vi "参数生成器.vi"() -> ()   [LabVIEW 2013]
uses:
  <vilib>/Utility/config.llb/Write Key (String).vi
  <vilib>/Utility/config.llb/Read Key (String).vi
  <vilib>/Utility/file.llb/Read From Spreadsheet File (string).vi
  <vilib>/Utility/config.llb/Write Key (Path).vi
  <vilib>/Utility/config.llb/NI_LVConfig.lvlib
panel:
  in  "均衡参数设置":bool
  in  "error in":errorcluster caption="错误输入"
  out "临时从板数据":string[](array[string])
  in  "自动记录":bool
  in  "通道电压清零":bool
  in  "自动计算通道电压":bool
  out "均衡参数":T1={"充电结束电压(90%)"=3.0, "充电结束电压(91%)"=3.0, "充电结束电压(92%)"=3.0, "充电结束电压(93%)"=3.0, "充电结束电压(94%)"=3.0, "均衡计算-电压高阀值1级"=3.0, "均衡计算-电压高阀值2级"=3.0, "均衡计算-电压低阀值1级"=3.0, "均衡计算-电压低阀值2级"=3.0, "均衡计算-最低电压阀值"=3.0, "均衡停止-最低电压阀值"=3.0, "均衡计算-电压极差阀值"=3.0, "充电结束电压(95%)"=3.0, "充电结束电压(96%)"=3.0, "充电结束电压(97%)"=3.0, "充电结束电压(98%)"=3.0, "充电结束电压(99%)"=3.0, "充电结束电压(100%)"=3.0} {"充电结束电压(100%)" min=0 max=5 format="%#.4f"; "充电结束电压(99%)" min=0 max=5 format="%#.4f"; "充电结束电压(98%)" min=0 max=5 format="%#.4f"; "充电结束电压(97%)" min=0 max=5 format="%#.4f"; "充电结束电压(96%)" min=0 max=5 format="%#.4f"; "充电结束电压(95%)" min=0 max=5 format="%#.4f"; "均衡计算-电压极差阀值" min=0 max=5 format="%#.4f"; "均衡停止-最低电压阀值" min=0 max=5 format="%#.4f"; "均衡计算-最低电压阀值" min=0 max=5 format="%#.4f"; "均衡计算-电压低阀值2级" min=0 max=5 format="%#.4f"; "充电结束电压(94%)" min=0 max=5 format="%#.4f"; "充电结束电压(93%)" min=0 max=5 format="%#.4f"; "均衡计算-电压低阀值1级" min=0 max=5 format="%#.4f"; "均衡计算-电压高阀值1级" min=0 max=5 format="%#.4f"; "均衡计算-电压高阀值2级" min=0 max=5 format="%#.4f"; "充电结束电压(92%)" min=0 max=5 format="%#.4f"; "充电结束电压(91%)" min=0 max=5 format="%#.4f"; "充电结束电压(90%)" min=0 max=5 format="%#.4f"}
  in  "布尔":bool
  in  "全部记录":bool
  in  "查看":bool
  in  "读从板信息":bool
  in  "字符串":string
  out "MD5 message-digest":string="c47cafb9475eca419ba2638971991389" caption="MD5信息摘要"
  out "从板表头":string[](array[string])=["从板板号", "电压个数", "电压起始值", "温度个数", "温度起始值", "第一个保险通道", "第一个保险位置", "第二个保险通道", "第二个保险位置", "第三个保险通道", "第三个保险位置", "第四个保险通道", "第四个保险位置", "第五个保险通道", "第五个保险位置", "第六个保险通道", "第六个保险位置", "第七个保险通道", "第七个保险位置", "第八个保险通道", "第八个保险位置", "第九个保险通道", "第九个保险位置", "第十个保险通道", "第十个保险位置", "第1通道电压个数", "第2通道电压个数", "第3通道电压个数", "第4通道电压个数", "第5通道电压个数", "第6通道电压个数", "第7通道电压个数", "第8通道电压个数", "第9通道电压个数", "第10通道电压个数", "第11通道电压个数", "第12通道电压个数", "第13通道电压个数", "第14通道电压个数", "第15通道电压个数", "第16通道电压个数", "第17通道电压个数", "第18通道电压个数", "第19通道电压个数", "第20通道电压个数", "风机开启温度", "风机关闭温度", "加热开启温度", "加热关闭温度", "风机开启温差", "风机关闭温差", "加热关闭温差", "电压过高一级", "电压过低一级", "温度过高一级", "温度过低一级", "电压不均衡一级", "温度不均衡一级", "SOC过低一级", "电压过高二级", "电压过低二级", "温度过高二级", "温度过低二级", "电压不均衡二级", "温度不均衡二级", "SOC过低二级", "电压过高三级", "电压过低三级", "温度过高三级", "温度过低三级", "电压不均衡三级", "温度不均衡三级", "SOC过低三级", "均衡计算-电压高阀值1级", "均衡计算-电压高阀值2级", "均衡计算-电压低阀值1级", "均衡计算-电压低阀值2级", "均衡计算-最低电压阀值", "均衡停止-最低电压阀值", "均衡计算-电压极差阀值", "充电结束电压(90%)", "充电结束电压(91%)", "充电结束电压(92%)", "充电结束电压(93%)", "充电结束电压(94%)", "充电结束电压(95%)", "充电结束电压(96%)", "充电结束电压(97%)", "充电结束电压(98%)", "充电结束电压(99%)", "充电结束电压(100%)"]
  out "输出数组":string[][](array[string])=[["1", "2", "3", " ", " ", " ", " ", " ", " ", " ", " ", " ", " ", " ", " ", " ", " ", " ", " ", " ", " ", " ", " ", " ", " ", " ", " ", " ", " ", " "], ["10", "10", "10", " ", " ", " ", " ", " ", " ", " ", " ", " ", " ", " ", " ", " ", " ", " ", " ", " ", " ", " ", " ", " ", " ", " ", " ", " ", " ", " "], ["", "0", "0", " ", " ", " ", " ", " ", " ", " ", " ", " ", " ", " ", " ", " ", " ", " ", " ", " ", " ", " ", " ", " ", " ", " ", " ", " ", " ", " "], ["2", "2", "2", " ", " ", " ", " ", " ", " ", " ", " ", " ", " ", " ", " ", " ", " ", " ", " ", " ", " ", " ", " ", " ", " ", " ", " ", " ", " ", " "], ["", "0", "0", " ", " ", " ", " ", " ", " ", " ", " ", " ", " ", " ", " ", " ", " ", " ", " ", " ", " ", " ", " ", " ", " ", " ", " ", " ", " ", " "], [" ", " ", " ", " ", " ", " ", " ", " ", " ", " ", " ", " ", " ", " ", " ", " ", " ", " ", " ", " ", " ", " ", " ", " ", " ", " ", " ", " ", " ", " "], [" ", " ", " ", " ", " ", " ", " ", " ", " ", " ", " ", " ", " ", " ", " ", " ", " ", " ", " ", " ", " ", " ", " ", " ", " ", " ", " ", " ", " ", " "], [" ", " ", " ", " ", " ", " ", " ", " ", " ", " ", " ", " ", " ", " ", " ", " ", " ", " ", " ", " ", " ", " ", " ", " ", " ", " ", " ", " ", " ", " "], [" ", " ", " ", " ", " ", " ", " ", " ", " ", " ", " ", " ", " ", " ", " ", " ", " ", " ", " ", " ", " ", " ", " ", " ", " ", " ", " ", " ", " ", " "], [" ", " ", " ", " ", " ", " ", " ", " ", " ", " ", " ", " ", " ", " ", " ", " ", " ", " ", " ", " ", " ", " ", " ", " ", " ", " ", " ", " ", " ", " "], [" ", " ", " ", " ", " ", " ", " ", " ", " ", " ", " ", " ", " ", " ", " ", " ", " ", " ", " ", " ", " ", " ", " ", " ", " ", " ", " ", " ", " ", " "], [" ", " ", " ", " ", " ", " ", " ", " ", " ", " ", " ", " ", " ", " ", " ", " ", " ", " ", " ", " ", " ", " ", " ", " ", " ", " ", " ", " ", " ", " "], [" ", " ", " ", " ", " ", " ", " ", " ", " ", " ", " ", " ", " ", " ", " ", " ", " ", " ", " ", " ", " ", " ", " ", " ", " ", " ", " ", " ", " ", " "], [" ", " ", " ", " ", " ", " ", " ", " ", " ", " ", " ", " ", " ", " ", " ", " ", " ", " ", " ", " ", " ", " ", " ", " ", " ", " ", " ", " ", " ", " "], [" ", " ", " ", " ", " ", " ", " ", " ", " ", " ", " ", " ", " ", " ", " ", " ", " ", " ", " ", " ", " ", " ", " ", " ", " ", " ", " ", " ", " ", " "], [" ", " ", " ", " ", " ", " ", " ", " ", " ", " ", " ", " ", " ", " ", " ", " ", " ", " ", " ", " ", " ", " ", " ", " ", " ", " ", " ", " ", " ", " "], [" ", " ", " ", " ", " ", " ", " ", " ", " ", " ", " ", " ", " ", " ", " ", " ", " ", " ", " ", " ", " ", " ", " ", " ", " ", " ", " ", " ", " ", " "], [" ", " ", " ", " ", " ", " ", " ", " ", " ", " ", " ", " ", " ", " ", " ", " ", " ", " ", " ", " ", " ", " ", " ", " ", " ", " ", " ", " ", " ", " "], [" ", " ", " ", " ", " ", " ", " ", " ", " ", " ", " ", " ", " ", " ", " ", " ", " ", " ", " ", " ", " ", " ", " ", " ", " ", " ", " ", " ", " ", " "], [" ", " ", " ", " ", " ", " ", " ", " ", " ", " ", " ", " ", " ", " ", " ", " ", " ", " ", " ", " ", " ", " ", " ", " ", " ", " ", " ", " ", " ", " "], [" ", " ", " ", " ", " ", " ", " ", " ", " ", " ", " ", " ", " ", " ", " ", " ", " ", " ", " ", " ", " ", " ", " ", " ", " ", " ", " ", " ", " ", " "], [" ", " ", " ", " ", " ", " ", " ", " ", " ", " ", " ", " ", " ", " ", " ", " ", " ", " ", " ", " ", " ", " ", " ", " ", " ", " ", " ", " ", " ", " "], [" ", " ", " ", " ", " ", " ", " ", " ", " ", " ", " ", " ", " ", " ", " ", " ", " ", " ", " ", " ", " ", " ", " ", " ", " ", " ", " ", " ", " ", " "], [" ", " ", " ", " ", " ", " ", " ", " ", " ", " ", " ", " ", " ", " ", " ", " ", " ", " ", " ", " ", " ", " ", " ", " ", " ", " ", " ", " ", " ", " "], [" ", " ", " ", " ", " ", " ", " ", " ", " ", " ", " ", " ", " ", " ", " ", " ", " ", " ", " ", " ", " ", " ", " ", " ", " ", " ", " ", " ", " ", " "], [" ", " ", " ", " ", " ", " ", " ", " ", " ", " ", " ", " ", " ", " ", " ", " ", " ", " ", " ", " ", " ", " ", " ", " ", " ", " ", " ", " ", " ", " "], [" ", " ", " ", " ", " ", " ", " ", " ", " ", " ", " ", " ", " ", " ", " ", " ", " ", " ", " ", " ", " ", " ", " ", " ", " ", " ", " ", " ", " ", " "], [" ", " ", " ", " ", " ", " ", " ", " ", " ", " ", " ", " ", " ", " ", " ", " ", " ", " ", " ", " ", " ", " ", " ", " ", " ", " ", " ", " ", " ", " "], [" ", " ", " ", " ", " ", " ", " ", " ", " ", " ", " ", " ", " ", " ", " ", " ", " ", " ", " ", " ", " ", " ", " ", " ", " ", " ", " ", " ", " ", " "], [" ", " ", " ", " ", " ", " ", " ", " ", " ", " ", " ", " ", " ", " ", " ", " ", " ", " ", " ", " ", " ", " ", " ", " ", " ", " ", " ", " ", " ", " "], [" ", " ", " ", " ", " ", " ", " ", " ", " ", " ", " ", " ", " ", " ", " ", " ", " ", " ", " ", " ", " ", " ", " ", " ", " ", " ", " ", " ", " ", " "], [" ", " ", " ", " ", " ", " ", " ", " ", " ", " ", " ", " ", " ", " ", " ", " ", " ", " ", " ", " ", " ", " ", " ", " ", " ", " ", " ", " ", " ", " "], [" ", " ", " ", " ", " ", " ", " ", " ", " ", " ", " ", " ", " ", " ", " ", " ", " ", " ", " ", " ", " ", " ", " ", " ", " ", " ", " ", " ", " ", " "], [" ", " ", " ", " ", " ", " ", " ", " ", " ", " ", " ", " ", " ", " ", " ", " ", " ", " ", " ", " ", " ", " ", " ", " ", " ", " ", " ", " ", " ", " "], [" ", " ", " ", " ", " ", " ", " ", " ", " ", " ", " ", " ", " ", " ", " ", " ", " ", " ", " ", " ", " ", " ", " ", " ", " ", " ", " ", " ", " ", " "], [" ", " ", " ", " ", " ", " ", " ", " ", " ", " ", " ", " ", " ", " ", " ", " ", " ", " ", " ", " ", " ", " ", " ", " ", " ", " ", " ", " ", " ", " "], [" ", " ", " ", " ", " ", " ", " ", " ", " ", " ", " ", " ", " ", " ", " ", " ", " ", " ", " ", " ", " ", " ", " ", " ", " ", " ", " ", " ", " ", " "], [" ", " ", " ", " ", " ", " ", " ", " ", " ", " ", " ", " ", " ", " ", " ", " ", " ", " ", " ", " ", " ", " ", " ", " ", " ", " ", " ", " ", " ", " "], [" ", " ", " ", " ", " ", " ", " ", " ", " ", " ", " ", " ", " ", " ", " ", " ", " ", " ", " ", " ", " ", " ", " ", " ", " ", " ", " ", " ", " ", " "], [" ", " ", " ", " ", " ", " ", " ", " ", " ", " ", " ", " ", " ", " ", " ", " ", " ", " ", " ", " ", " ", " ", " ", " ", " ", " ", " ", " ", " ", " "], [" ", " ", " ", " ", " ", " ", " ", " ", " ", " ", " ", " ", " ", " ", " ", " ", " ", " ", " ", " ", " ", " ", " ", " ", " ", " ", " ", " ", " ", " "], [" ", " ", " ", " ", " ", " ", " ", " ", " ", " ", " ", " ", " ", " ", " ", " ", " ", " ", " ", " ", " ", " ", " ", " ", " ", " ", " ", " ", " ", " "], [" ", " ", " ", " ", " ", " ", " ", " ", " ", " ", " ", " ", " ", " ", " ", " ", " ", " ", " ", " ", " ", " ", " ", " ", " ", " ", " ", " ", " ", " "], [" ", " ", " ", " ", " ", " ", " ", " ", " ", " ", " ", " ", " ", " ", " ", " ", " ", " ", " ", " ", " ", " ", " ", " ", " ", " ", " ", " ", " ", " "], [" ", " ", " ", " ", " ", " ", " ", " ", " ", " ", " ", " ", " ", " ", " ", " ", " ", " ", " ", " ", " ", " ", " ", " ", " ", " ", " ", " ", " ", " "], ["35", "35", "35", " ", " ", " ", " ", " ", " ", " ", " ", " ", " ", " ", " ", " ", " ", " ", " ", " ", " ", " ", " ", " ", " ", " ", " ", " ", " ", " "], ["30", "30", "30", " ", " ", " ", " ", " ", " ", " ", " ", " ", " ", " ", " ", " ", " ", " ", " ", " ", " ", " ", " ", " ", " ", " ", " ", " ", " ", " "], ["0", "0", "0", " ", " ", " ", " ", " ", " ", " ", " ", " ", " ", " ", " ", " ", " ", " ", " ", " ", " ", " ", " ", " ", " ", " ", " ", " ", " ", " "], ["5", "5", "5", " ", " ", " ", " ", " ", " ", " ", " ", " ", " ", " ", " ", " ", " ", " ", " ", " ", " ", " ", " ", " ", " ", " ", " ", " ", " ", " "], ["5", "5", "5", " ", " ", " ", " ", " ", " ", " ", " ", " ", " ", " ", " ", " ", " ", " ", " ", " ", " ", " ", " ", " ", " ", " ", " ", " ", " ", " "], ["3", "3", "3", " ", " ", " ", " ", " ", " ", " ", " ", " ", " ", " ", " ", " ", " ", " ", " ", " ", " ", " ", " ", " ", " ", " ", " ", " ", " ", " "], ["10", "10", "10", " ", " ", " ", " ", " ", " ", " ", " ", " ", " ", " ", " ", " ", " ", " ", " ", " ", " ", " ", " ", " ", " ", " ", " ", " ", " ", " "], ["4.23", "4.23", "4.23", " ", " ", " ", " ", " ", " ", " ", " ", " ", " ", " ", " ", " ", " ", " ", " ", " ", " ", " ", " ", " ", " ", " ", " ", " ", " ", " "], ["3", "3", "3", " ", " ", " ", " ", " ", " ", " ", " ", " ", " ", " ", " ", " ", " ", " ", " ", " ", " ", " ", " ", " ", " ", " ", " ", " ", " ", " "], ["50", "50", "50", " ", " ", " ", " ", " ", " ", " ", " ", " ", " ", " ", " ", " ", " ", " ", " ", " ", " ", " ", " ", " ", " ", " ", " ", " ", " ", " "], ["-20", "-20", "-20", " ", " ", " ", " ", " ", " ", " ", " ", " ", " ", " ", " ", " ", " ", " ", " ", " ", " ", " ", " ", " ", " ", " ", " ", " ", " ", " "], ["0.5", "0.5", "0.5", " ", " ", " ", " ", " ", " ", " ", " ", " ", " ", " ", " ", " ", " ", " ", " ", " ", " ", " ", " ", " ", " ", " ", " ", " ", " ", " "], ["25", "25", "25", " ", " ", " ", " ", " ", " ", " ", " ", " ", " ", " ", " ", " ", " ", " ", " ", " ", " ", " ", " ", " ", " ", " ", " ", " ", " ", " "], ["30", "30", "30", " ", " ", " ", " ", " ", " ", " ", " ", " ", " ", " ", " ", " ", " ", " ", " ", " ", " ", " ", " ", " ", " ", " ", " ", " ", " ", " "], ["4.25", "4.25", "4.25", " ", " ", " ", " ", " ", " ", " ", " ", " ", " ", " ", " ", " ", " ", " ", " ", " ", " ", " ", " ", " ", " ", " ", " ", " ", " ", " "], ["2.75", "2.75", "2.75", " ", " ", " ", " ", " ", " ", " ", " ", " ", " ", " ", " ", " ", " ", " ", " ", " ", " ", " ", " ", " ", " ", " ", " ", " ", " ", " "], ["55", "55", "55", " ", " ", " ", " ", " ", " ", " ", " ", " ", " ", " ", " ", " ", " ", " ", " ", " ", " ", " ", " ", " ", " ", " ", " ", " ", " ", " "], ["-30", "-30", "-30", " ", " ", " ", " ", " ", " ", " ", " ", " ", " ", " ", " ", " ", " ", " ", " ", " ", " ", " ", " ", " ", " ", " ", " ", " ", " ", " "], ["1", "1", "1", " ", " ", " ", " ", " ", " ", " ", " ", " ", " ", " ", " ", " ", " ", " ", " ", " ", " ", " ", " ", " ", " ", " ", " ", " ", " ", " "], ["30", "30", "30", " ", " ", " ", " ", " ", " ", " ", " ", " ", " ", " ", " ", " ", " ", " ", " ", " ", " ", " ", " ", " ", " ", " ", " ", " ", " ", " "], ["20", "20", "20", " ", " ", " ", " ", " ", " ", " ", " ", " ", " ", " ", " ", " ", " ", " ", " ", " ", " ", " ", " ", " ", " ", " ", " ", " ", " ", " "], ["4.3", "4.3", "4.3", " ", " ", " ", " ", " ", " ", " ", " ", " ", " ", " ", " ", " ", " ", " ", " ", " ", " ", " ", " ", " ", " ", " ", " ", " ", " ", " "], ["2.5", "2.5", "2.5", " ", " ", " ", " ", " ", " ", " ", " ", " ", " ", " ", " ", " ", " ", " ", " ", " ", " ", " ", " ", " ", " ", " ", " ", " ", " ", " "], ["60", "60", "60", " ", " ", " ", " ", " ", " ", " ", " ", " ", " ", " ", " ", " ", " ", " ", " ", " ", " ", " ", " ", " ", " ", " ", " ", " ", " ", " "], ["-40", "-40", "-40", " ", " ", " ", " ", " ", " ", " ", " ", " ", " ", " ", " ", " ", " ", " ", " ", " ", " ", " ", " ", " ", " ", " ", " ", " ", " ", " "], ["1.5", "1.5", "1.5", " ", " ", " ", " ", " ", " ", " ", " ", " ", " ", " ", " ", " ", " ", " ", " ", " ", " ", " ", " ", " ", " ", " ", " ", " ", " ", " "], ["35", "35", "35", " ", " ", " ", " ", " ", " ", " ", " ", " ", " ", " ", " ", " ", " ", " ", " ", " ", " ", " ", " ", " ", " ", " ", " ", " ", " ", " "], ["10", "10", "10", " ", " ", " ", " ", " ", " ", " ", " ", " ", " ", " ", " ", " ", " ", " ", " ", " ", " ", " ", " ", " ", " ", " ", " ", " ", " ", " "], ["3", "4.23", "4.23", " ", " ", " ", " ", " ", " ", " ", " ", " ", " ", " ", " ", " ", " ", " ", " ", " ", " ", " ", " ", " ", " ", " ", " ", " ", " ", " "], ["3", "3", "3", " ", " ", " ", " ", " ", " ", " ", " ", " ", " ", " ", " ", " ", " ", " ", " ", " ", " ", " ", " ", " ", " ", " ", " ", " ", " ", " "], ["3", "50", "50", " ", " ", " ", " ", " ", " ", " ", " ", " ", " ", " ", " ", " ", " ", " ", " ", " ", " ", " ", " ", " ", " ", " ", " ", " ", " ", " "], ["3", "-20", "-20", " ", " ", " ", " ", " ", " ", " ", " ", " ", " ", " ", " ", " ", " ", " ", " ", " ", " ", " ", " ", " ", " ", " ", " ", " ", " ", " "], ["3", "0.5", "0.5", " ", " ", " ", " ", " ", " ", " ", " ", " ", " ", " ", " ", " ", " ", " ", " ", " ", " ", " ", " ", " ", " ", " ", " ", " ", " ", " "], ["3", "25", "25", " ", " ", " ", " ", " ", " ", " ", " ", " ", " ", " ", " ", " ", " ", " ", " ", " ", " ", " ", " ", " ", " ", " ", " ", " ", " ", " "], ["3", "30", "30", " ", " ", " ", " ", " ", " ", " ", " ", " ", " ", " ", " ", " ", " ", " ", " ", " ", " ", " ", " ", " ", " ", " ", " ", " ", " ", " "], ["3", "4.25", "4.25", " ", " ", " ", " ", " ", " ", " ", " ", " ", " ", " ", " ", " ", " ", " ", " ", " ", " ", " ", " ", " ", " ", " ", " ", " ", " ", " "], ["3", "2.75", "2.75", " ", " ", " ", " ", " ", " ", " ", " ", " ", " ", " ", " ", " ", " ", " ", " ", " ", " ", " ", " ", " ", " ", " ", " ", " ", " ", " "], ["3", "55", "55", " ", " ", " ", " ", " ", " ", " ", " ", " ", " ", " ", " ", " ", " ", " ", " ", " ", " ", " ", " ", " ", " ", " ", " ", " ", " ", " "], ["3", "-30", "-30", " ", " ", " ", " ", " ", " ", " ", " ", " ", " ", " ", " ", " ", " ", " ", " ", " ", " ", " ", " ", " ", " ", " ", " ", " ", " ", " "], ["3", "1", "1", " ", " ", " ", " ", " ", " ", " ", " ", " ", " ", " ", " ", " ", " ", " ", " ", " ", " ", " ", " ", " ", " ", " ", " ", " ", " ", " "], ["3", "30", "30", " ", " ", " ", " ", " ", " ", " ", " ", " ", " ", " ", " ", " ", " ", " ", " ", " ", " ", " ", " ", " ", " ", " ", " ", " ", " ", " "], ["3", "20", "20", " ", " ", " ", " ", " ", " ", " ", " ", " ", " ", " ", " ", " ", " ", " ", " ", " ", " ", " ", " ", " ", " ", " ", " ", " ", " ", " "], ["3", "4.3", "4.3", " ", " ", " ", " ", " ", " ", " ", " ", " ", " ", " ", " ", " ", " ", " ", " ", " ", " ", " ", " ", " ", " ", " ", " ", " ", " ", " "], ["3", "2.5", "2.5", " ", " ", " ", " ", " ", " ", " ", " ", " ", " ", " ", " ", " ", " ", " ", " ", " ", " ", " ", " ", " ", " ", " ", " ", " ", " ", " "], ["3", "60", "60", " ", " ", " ", " ", " ", " ", " ", " ", " ", " ", " ", " ", " ", " ", " ", " ", " ", " ", " ", " ", " ", " ", " ", " ", " ", " ", " "], ["3", "-40", "-40", " ", " ", " ", " ", " ", " ", " ", " ", " ", " ", " ", " ", " ", " ", " ", " ", " ", " ", " ", " ", " ", " ", " ", " ", " ", " ", " "], [" ", "1.5", "1.5", " ", " ", " ", " ", " ", " ", " ", " ", " ", " ", " ", " ", " ", " ", " ", " ", " ", " ", " ", " ", " ", " ", " ", " ", " ", " ", " "], [" ", "35", "35", " ", " ", " ", " ", " ", " ", " ", " ", " ", " ", " ", " ", " ", " ", " ", " ", " ", " ", " ", " ", " ", " ", " ", " ", " ", " ", " "], [" ", "10", "10", " ", " ", " ", " ", " ", " ", " ", " ", " ", " ", " ", " ", " ", " ", " ", " ", " ", " ", " ", " ", " ", " ", " ", " ", " ", " ", " "], [" ", "3", "4.23", " ", " ", " ", " ", " ", " ", " ", " ", " ", " ", " ", " ", " ", " ", " ", " ", " ", " ", " ", " ", " ", " ", " ", " ", " ", " ", " "], [" ", "3", "3", " ", " ", " ", " ", " ", " ", " ", " ", " ", " ", " ", " ", " ", " ", " ", " ", " ", " ", " ", " ", " ", " ", " ", " ", " ", " ", " "], [" ", "3", "50", " ", " ", " ", " ", " ", " ", " ", " ", " ", " ", " ", " ", " ", " ", " ", " ", " ", " ", " ", " ", " ", " ", " ", " ", " ", " ", " "], [" ", "3", "-20", " ", " ", " ", " ", " ", " ", " ", " ", " ", " ", " ", " ", " ", " ", " ", " ", " ", " ", " ", " ", " ", " ", " ", " ", " ", " ", " "], [" ", "3", "0.5", " ", " ", " ", " ", " ", " ", " ", " ", " ", " ", " ", " ", " ", " ", " ", " ", " ", " ", " ", " ", " ", " ", " ", " ", " ", " ", " "], [" ", "3", "25", " ", " ", " ", " ", " ", " ", " ", " ", " ", " ", " ", " ", " ", " ", " ", " ", " ", " ", " ", " ", " ", " ", " ", " ", " ", " ", " "]]
  in  "退出":bool
  in  "工程代号":string="B32615"
  in  "选项卡控件":enum32{"主板", "从板", "预览"}(tab)=enum."从板"
  in  "分流器型号":T2(ring)=enum."300A"
  in  "全部清零(主板)":bool
  in  "默认值":bool
  in  "读主板参数":bool
  in  "加热控制参数":T3={"风机开启温度(℃)"=30.0, "风机关闭温度(℃)"=20.0, "加热开启温度(℃)"=10.0, "加热关闭温度(℃)"=15.0, "风机开启温差(℃)"=5.0, "风机关闭温差(℃)"=3.0, "加热关闭温差(℃)"=10.0}
  in  "设电池信息主板":bool
  in  "电池信息":string[][](table)=[["电池串联", "92"], ["电池并联", "2"], ["电池包额定容量", "67"], ["电池包额定能量", "0"], ["电池包额定总电压", "340"], ["实际容量", "67"], ["电池厂家", "普莱德"], ["电池类型", "磷酸铁锂"], ["电池生产日期", "2013-12-11 11:34:30"], ["电池包组号", "0"], ["累计充电总安时", "0"], ["累计放电总安时", "0"], ["电池放空次数", "0"], ["电池充满次数", "0"], ["电池充电次数", "0"]]
  in  "一级故障":dbl[][](array[numeric])=[[389.0, 391.0, 395.0], [276.0, 253.0, 230.0], [50.0, 55.0, 60.0], [-20.0, -30.0, -40.0], [0.5, 1.0, 1.5], [0.5, 1.0, 1.5], [25.0, 30.0, 35.0], [25.0, 30.0, 35.0], [4.23, 4.25, 4.3], [3.0, 2.75, 2.5], [110.0, 132.0, 165.0], [250.0, 270.0, 300.0], [101.0, 101.0, 101.0], [30.0, 20.0, 10.0], [3.0, 5.0, 10.0], [50.0, 55.0, 60.0], [90.0, 80.0, 70.0]]
  in  "从板个数":dbl=3.0
  in  "主板信息":string[][](table)=[["电池额定容量", "0"], ["电池实际容量", "0"], ["SOC", "0"], ["SOH", "0"], ["产品编号", ""], ["车架(牌)号", ""], ["配置文件版本", ""], ["从板1电池节数", "10"], ["从板2电池节数", "10"], ["从板3电池节数", "10"], ["从板1温度个数", "2"], ["从板2温度个数", "2"], ["从板3温度个数", "2"]]
  in  "单个写入":bool
  in  "充电控制参数":T4={"最大允许单体电压(V)"=4.15, "最大允许总电压(V)"=382.0, "最小允许单体电压(V)"=2.75, "最大允许充电电流(A)"=50.0, "最小允许充电电流(A)"=3.0, "最大允许充电温度(℃)"=55.0, "最小允许充电温度(℃)"=-15.0, "电流步长"=5.0}
  in  "温度个数":dbl
  in  "电压个数":dbl
  in  "粘贴":bool
  in  "复制":T5
  in  "保险位置清零":bool
  in  "5个通道电压个数(最少5个电压)":u8[](array[numeric])=[0, 0, 0, 0, 0, 0, 0, 0, 0, 0, 0, 0, 0, 0, 0, 0, 0, 0, 0, 0] max=12
  in  "保险位置":T6
  in  "全部清零(从板)":bool
  in  "读从板参数":bool
  in  "从板板号":dbl=1.0 min=1.0 max=3.0 step=1.0
  in  "从板信息电压温度通道配置":string[][](table)=[["电压个数", "10"], ["电压起始值", ""], ["温度个数", "2"], ["温度起始值", ""], ["第一个保险通道", " "], ["第一个保险位置", " "], ["第二个保险通道", " "], ["第二个保险位置", " "], ["第三个保险通道", " "], ["第三个保险位置", " "], ["第四个保险通道", " "], ["第四个保险位置", " "], ["第五个保险通道", " "], ["第五个保险位置", " "], ["第六个保险通道", " "], ["第六个保险位置", " "], ["第七个保险通道", " "], ["第七个保险位置", " "], ["第八个保险通道", " "], ["第八个保险位置", " "], ["第九个保险通道", " "], ["第九个保险位置", " "], ["第十个保险通道", " "], ["第十个保险位置", " "], ["第1通道电压个数", " "], ["第2通道电压个数", " "], ["第3通道电压个数", " "], ["第4通道电压个数", " "], ["第5通道电压个数", " "], ["", " "], ["", " "], ["", " "], ["", " "], ["", " "], ["", " "], ["", " "], ["", " "], ["", " "], ["", " "], ["", " "], ["", " "], ["", " "], ["", " "], ["", " "]]
  in  "默认值 2":bool
  out "结果":i32(listbox)=-1
  in  "保存当前从板配置":T5
  in  "一级故障 2":dbl[][](array[numeric])=[[4.23, 4.25, 4.3], [3.0, 2.75, 2.5], [50.0, 55.0, 60.0], [-20.0, -30.0, -40.0], [0.5, 1.0, 1.5], [25.0, 30.0, 35.0], [30.0, 20.0, 10.0]] caption="一级故障"
  in  "加热控制参数 2":T3={"风机开启温度(℃)"=35.0, "风机关闭温度(℃)"=30.0, "加热开启温度(℃)"=0.0, "加热关闭温度(℃)"=5.0, "风机开启温差(℃)"=5.0, "风机关闭温差(℃)"=3.0, "加热关闭温差(℃)"=10.0}
  in  "主从板":enum32{"单选选项2", "单选选项1"}(radio)
  in  "读取(ini)":bool
  in  "预览":bool
  in  "工号":string="123"
  in  "写配置文件":bool
  # "操作说明 \n1） 输入从板1参数\n2） 完成后点“记录”\n3） 把参数更改成从板2参数\n4） 再点击“记录”\n5） 以此类推，直到完成所有从板"
  # "参数设置上位机"
  # "Step7->"
  # "<-Step3"
  # "Step2->"
  # "每个项目需要确认6个步骤都设置正确!"
  # "二级故障"
  # "三级故障"
  # "总电压过高(V)"
  # "Step1->"
  # "总电压过低(V)"
  # "温度过高(℃)"
  # "温度过低(℃)"
  # "<-Step4"
  # "整组电压不均衡(V)"
  # "单组电压不均衡(V)"
  # "整组温度不均衡(V)"
  # "单组温度不均衡(V)"
  # "单体电压过高(V)"
  # "单体电压过低(V)"
  # "<-Step5"
  # "充电电流过高(A)"
  # "Step6->"
  # "放电电流过高(A)"
  # "SOC过高(%)"
  # "SOC过低(%)"
  # "内阻过大(mΩ)"
  # "极柱温度过高(℃)"
  # "SOH过低(%)"
  # "Step1->"
  # "Step2->"
  # "1"
  # "2"
  # "3"
  # "4"
  # "5"
  # "Step3->"
  # "Step4->"
  # "Step5->"
  # "Step6->"
  # "1"
  # "2"
  # "3"
  # "7"
  # "4"
  # "5"
  # "6"
  # "8"
  # "9"
  # "10"
  # "11"
  # "12"
  # "通道1"
  # "通道2"
  # "通道3"
  # "通道4"
  # "通道5"
  # "二级故障"
  # "三级故障"
  # "电压过高(V)"
  # "电压过低(V)"
  # "温度过高(℃)"
  # "温度过低(℃)"
  # "电压不均衡(V)"
  # "温度不均衡(℃)"
  # "SOC过低(%)"
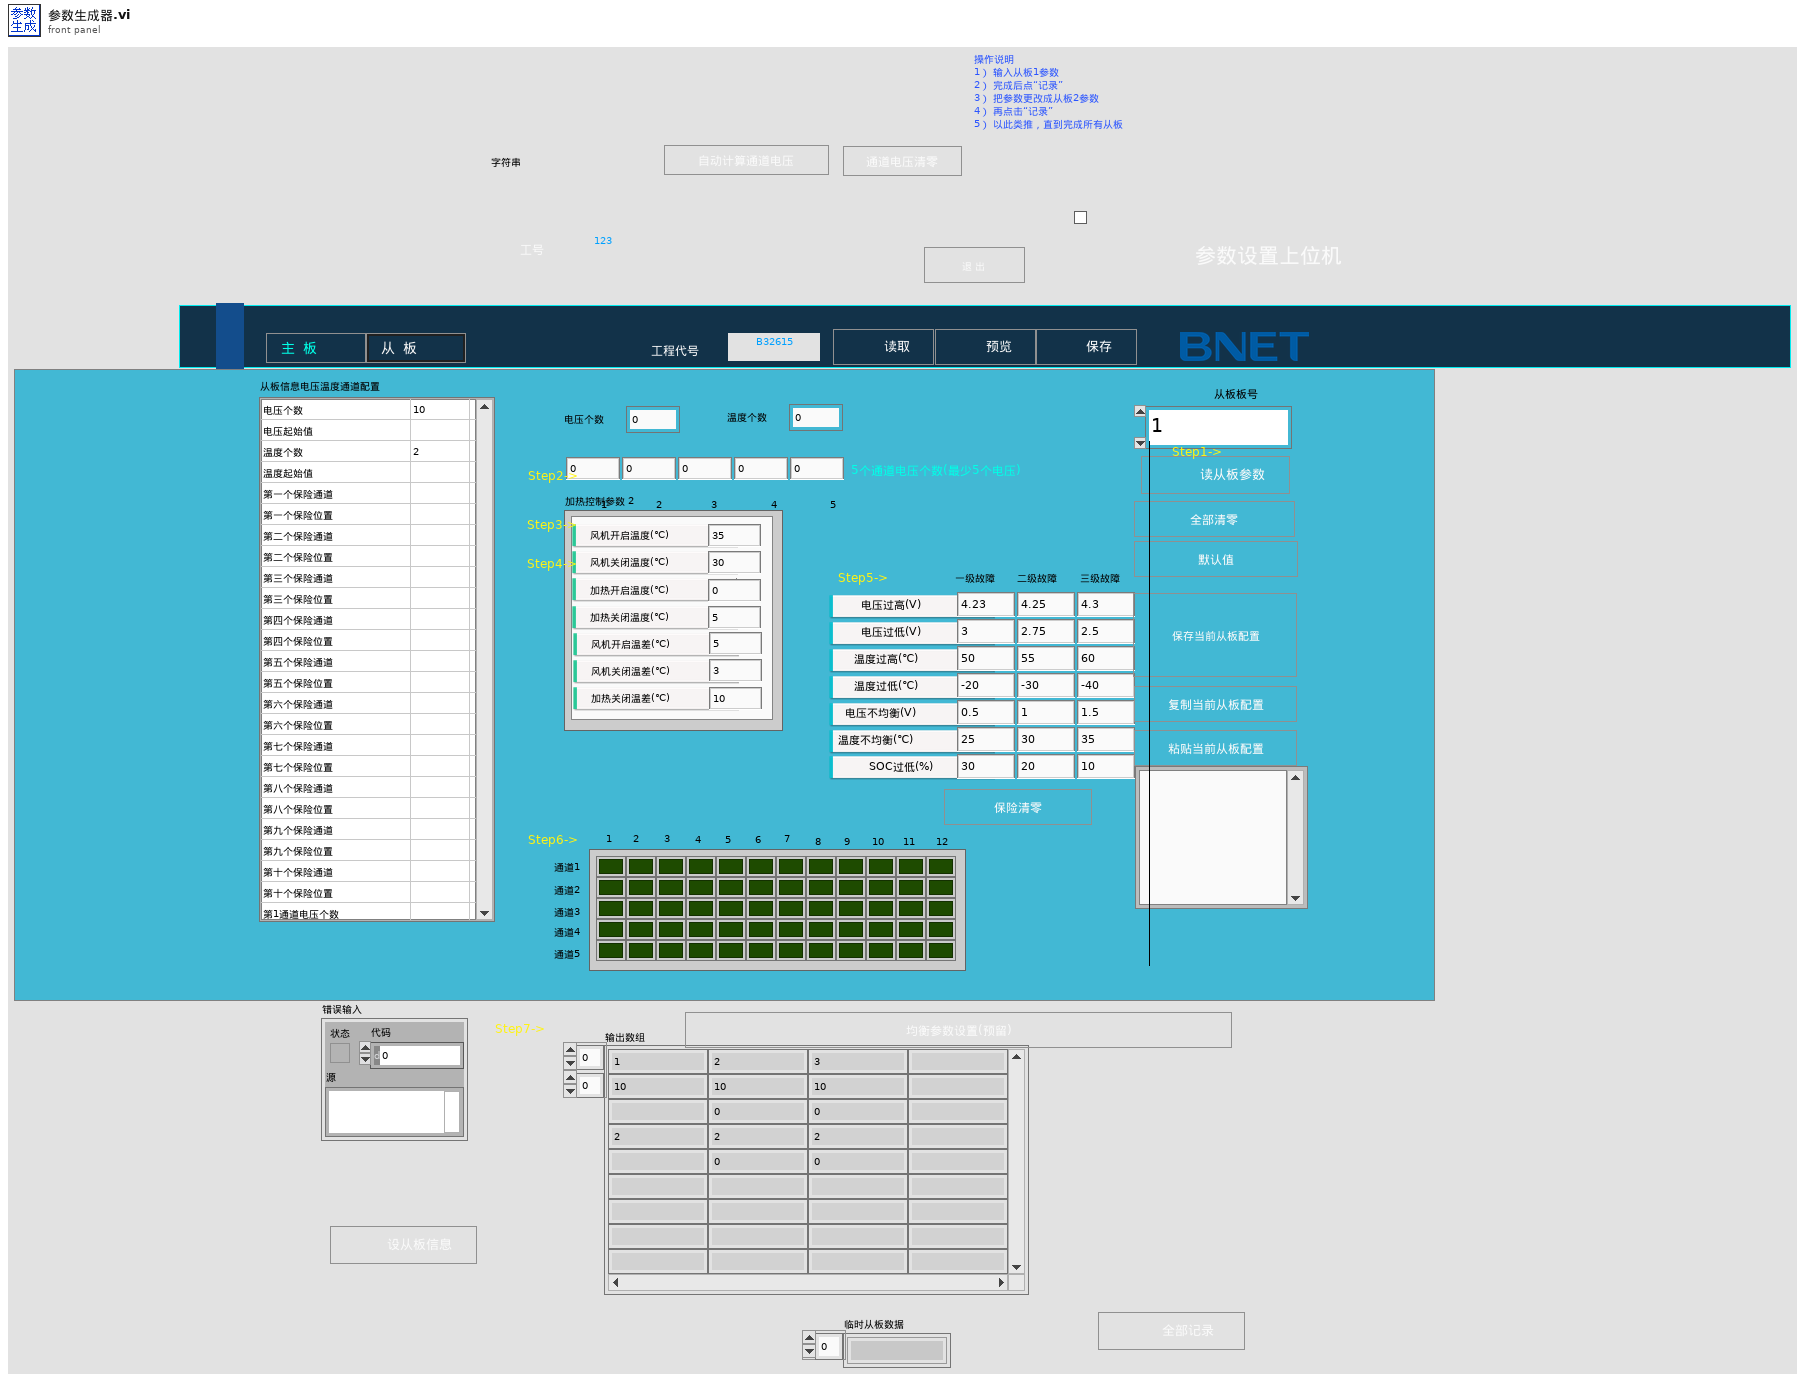
[diagram p1: front panel]
types:
  T1 = cluster{"充电结束电压(90%)":sgl, "充电结束电压(91%)":sgl, "充电结束电压(92%)":sgl, "充电结束电压(93%)":sgl, "充电结束电压(94%)":sgl, "均衡计算-电压高阀值1级":sgl, "均衡计算-电压高阀值2级":sgl, "均衡计算-电压低阀值1级":sgl, "均衡计算-电压低阀值2级":sgl, "均衡计算-最低电压阀值":sgl, "均衡停止-最低电压阀值":sgl, "均衡计算-电压极差阀值":sgl, "充电结束电压(95%)":sgl, "充电结束电压(96%)":sgl, "充电结束电压(97%)":sgl, "充电结束电压(98%)":sgl, "充电结束电压(99%)":sgl, "充电结束电压(100%)":sgl}
  T2 = enum16{"选择分流器型号", "100A", "200A", "300A", "400A", "500A", "600A", "700A", "800A", "900A", "1000A", "50A"}
  T3 = cluster{"风机开启温度(℃)":dbl, "风机关闭温度(℃)":dbl, "加热开启温度(℃)":dbl, "加热关闭温度(℃)":dbl, "风机开启温差(℃)":dbl, "风机关闭温差(℃)":dbl, "加热关闭温差(℃)":dbl}
  T4 = cluster{"最大允许单体电压(V)":dbl, "最大允许总电压(V)":dbl, "最小允许单体电压(V)":dbl, "最大允许充电电流(A)":dbl, "最小允许充电电流(A)":dbl, "最大允许充电温度(℃)":dbl, "最小允许充电温度(℃)":dbl, "电流步长":dbl}
  T5 = typedef "button.ctl" = bool
  T6 = typedef "111.ctl" = T7[][]
  T7 = typedef "保险位置.ctl" = bool
  T8 = cluster{"风机开启温度(℃)":dbl, "风机关闭温度(℃)":dbl, "加热开启温度(℃)":dbl, "加热关闭温度(℃)":dbl, "风机开启温差(℃)":dbl, "风机开启温度(℃)":dbl, "加热关闭温差(℃)":dbl}
  T9 = cluster{"风机开启温度":dbl, "风机关闭温度":dbl, "加热开启温度":dbl, "加热关闭温度":dbl, "风机开启温差":dbl, "风机关闭温差":dbl, "加热关闭温差":dbl}
  T10 = cluster{"[0]":dbl, "[1]":dbl, "[2]":dbl, "[3]":dbl, "[4]":dbl, "[5]":dbl, "[6]":dbl}
  T11 = typedef "NI_LVConfig.lvlib/Config Data RefNum.ctl" = refnum<k1>
  T12 = cluster{"[0]":dbl, "[1]":dbl, "[2]":dbl, "[3]":dbl, "[4]":dbl, "[5]":dbl, "[6]":dbl, "[7]":dbl}
  T13 = cluster{"[0]":dbl, "[1]":dbl, "[2]":dbl, "[3]":dbl, "[4]":dbl, "[5]":dbl, "[6]":dbl, "[7]":dbl, "[8]":dbl, "[9]":dbl, "[10]":dbl, "[11]":dbl, "[12]":dbl, "[13]":dbl, "[14]":dbl, "[15]":dbl, "[16]":dbl, "[17]":dbl}
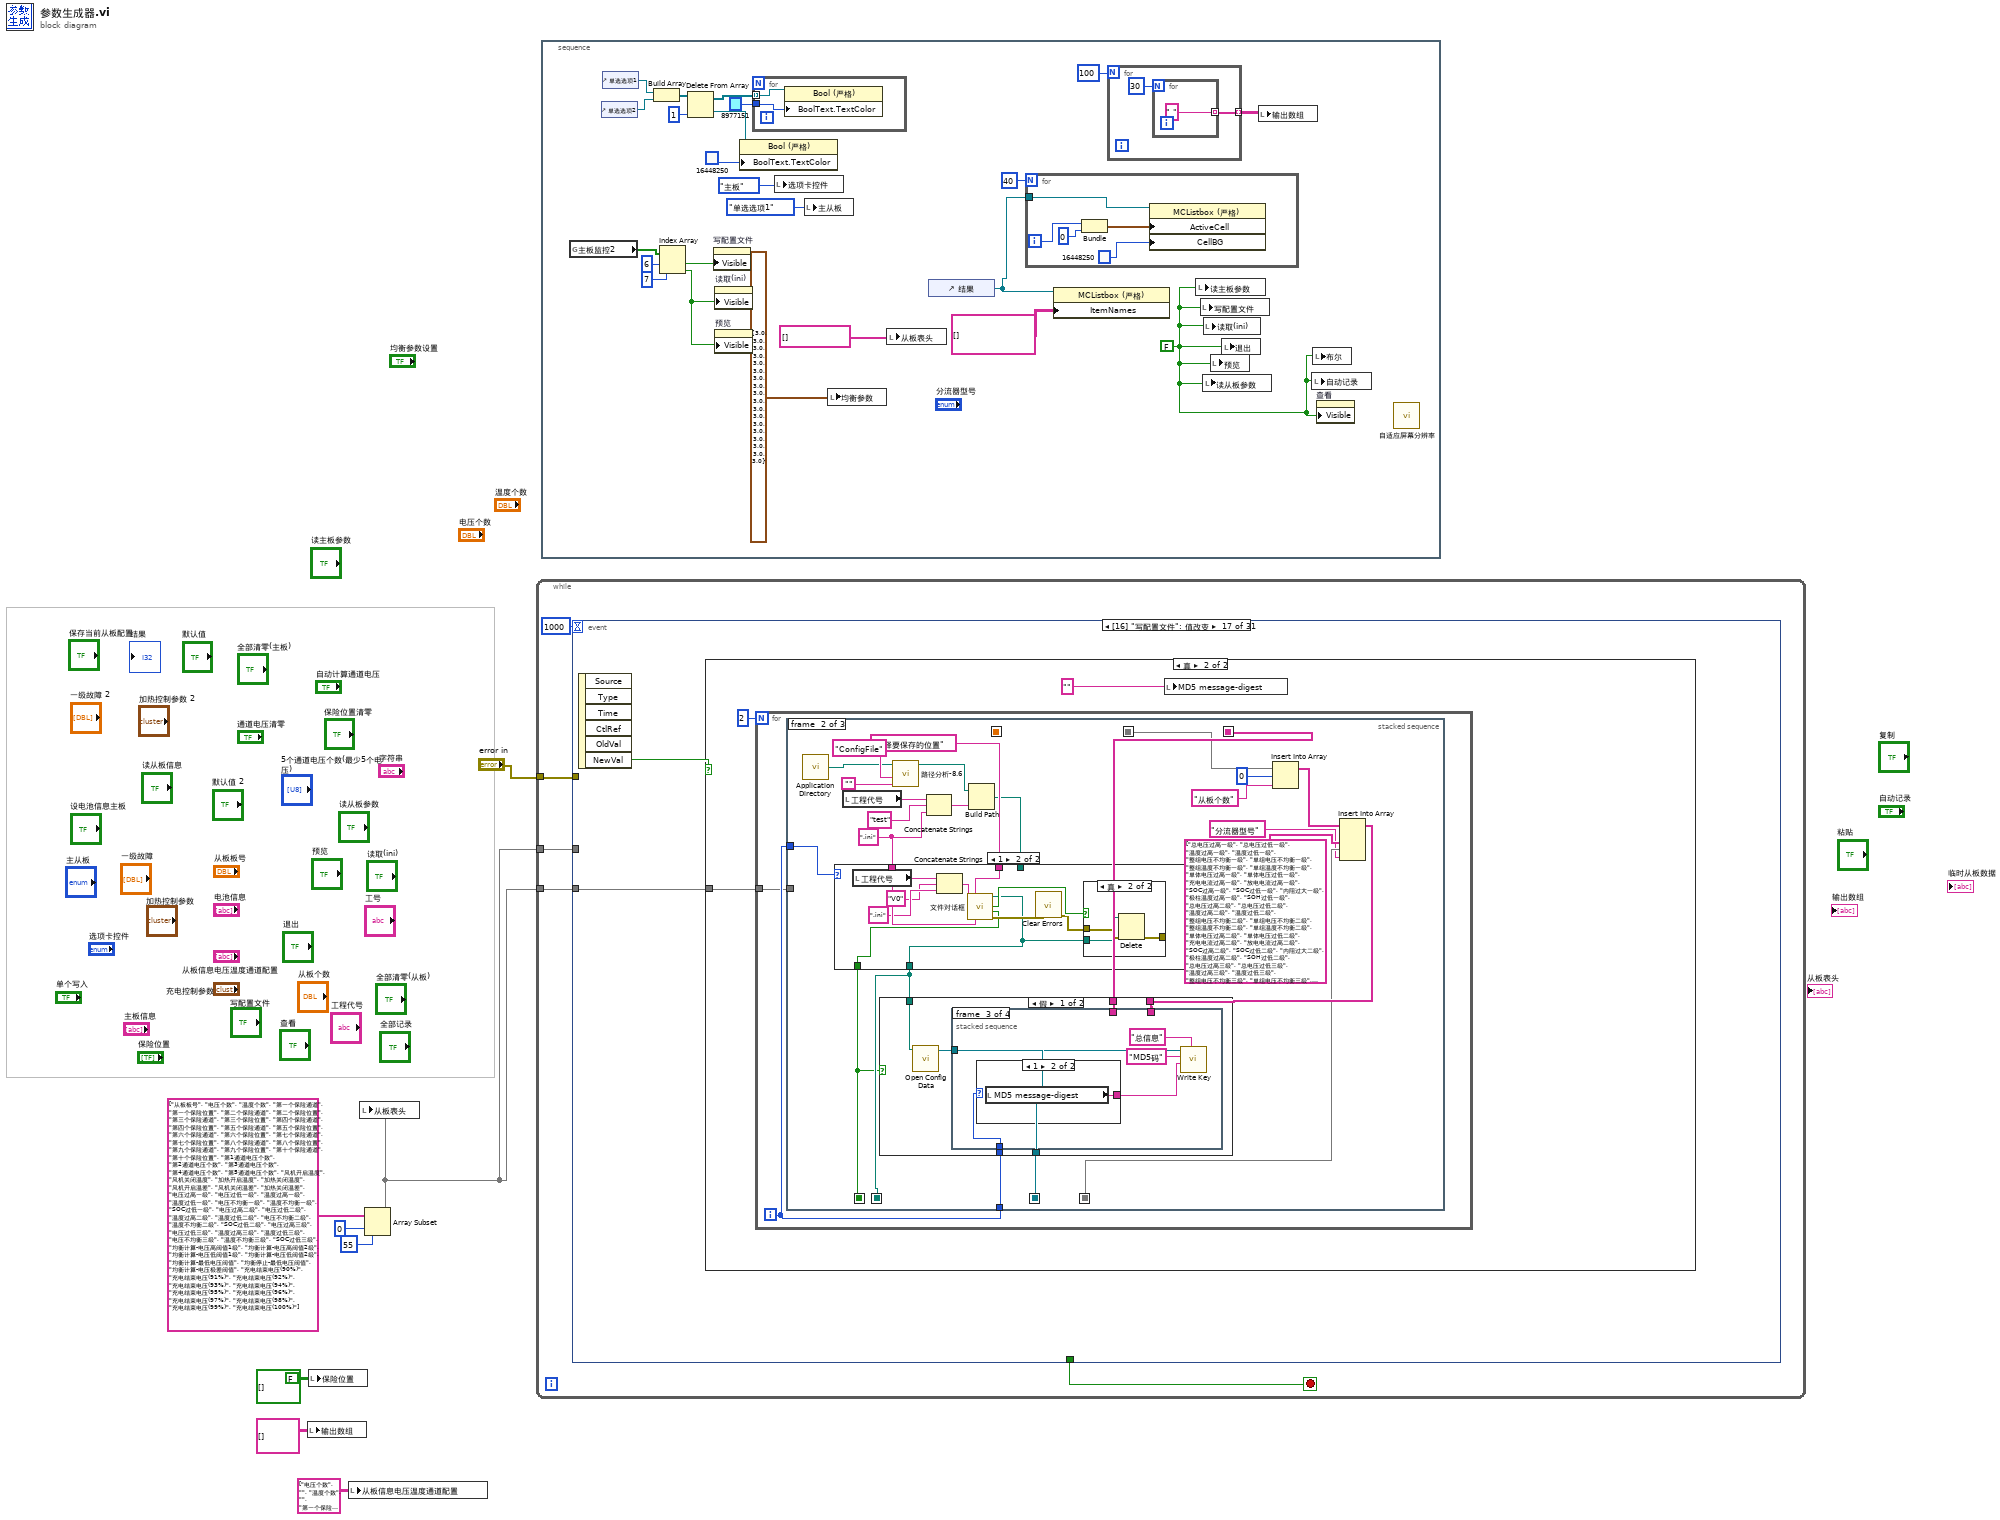
[diagram p0: block diagram]
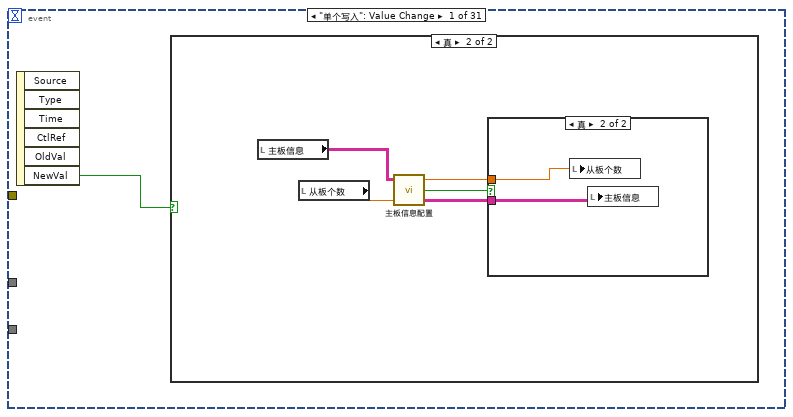
[diagram p2: hidden frame]
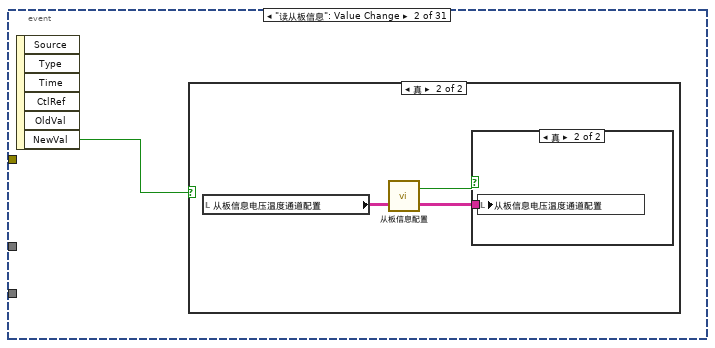
[diagram p5: hidden frame]
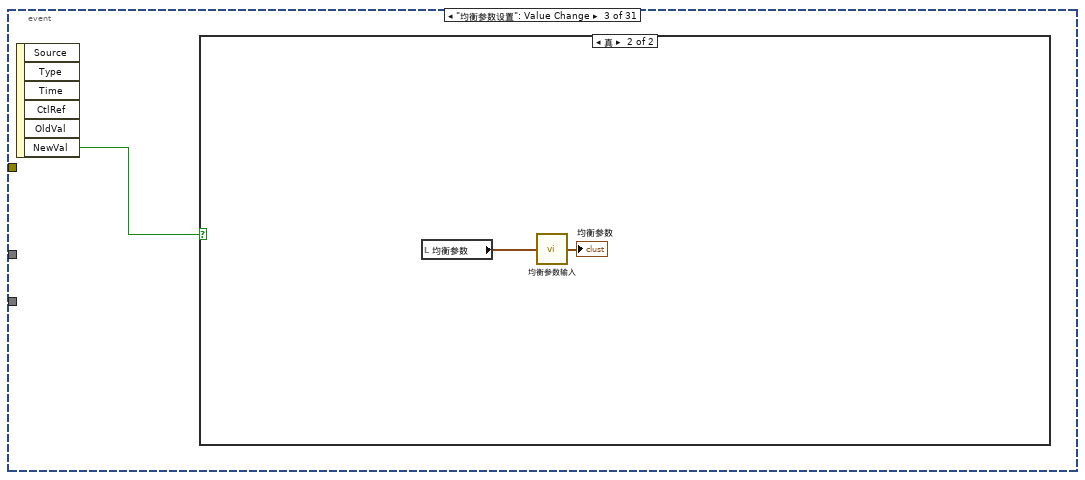
[diagram p8: hidden frame]
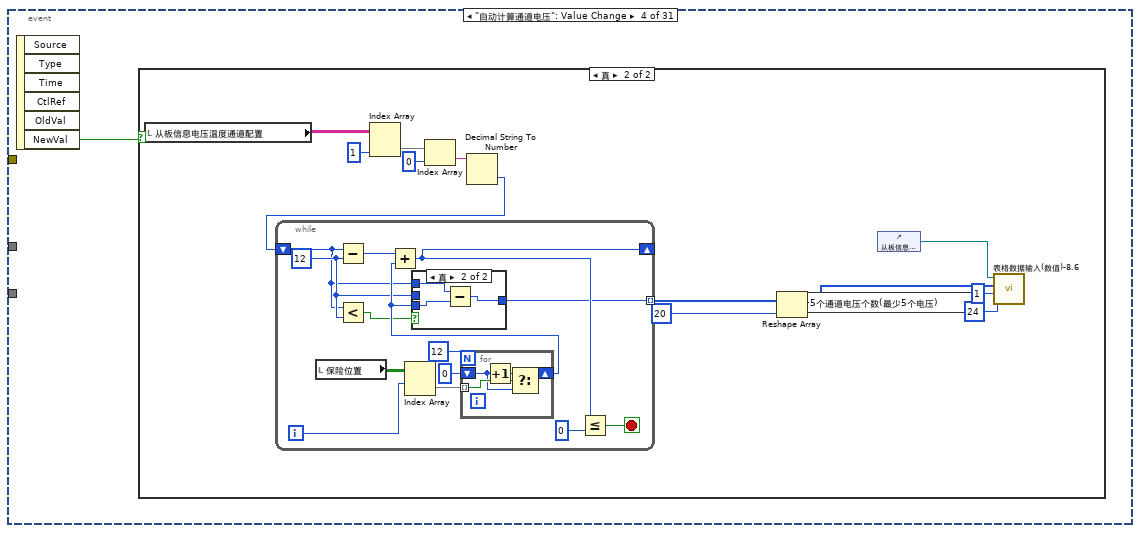
[diagram p10: hidden frame]
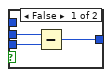
[diagram p12: hidden frame]
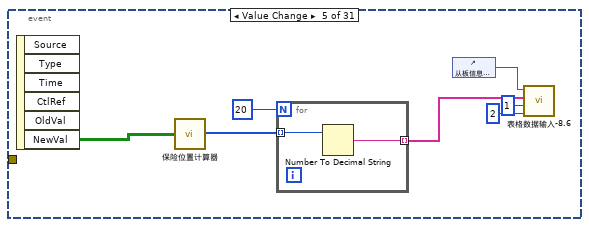
[diagram p13: hidden frame]
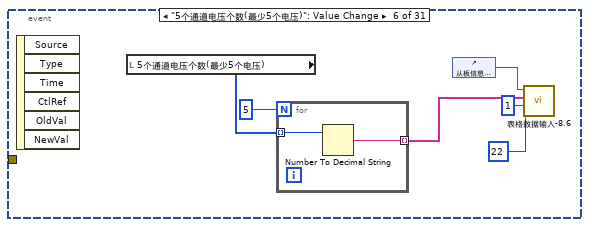
[diagram p14: hidden frame]
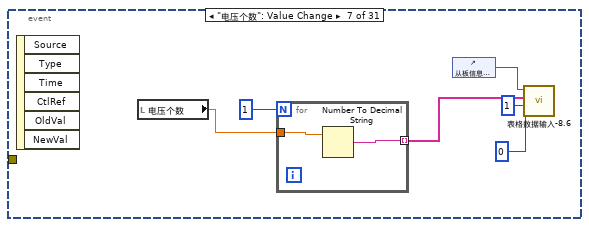
[diagram p15: hidden frame]
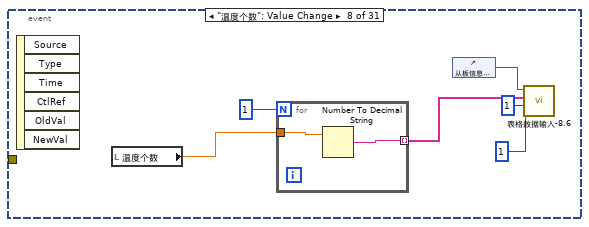
[diagram p16: hidden frame]
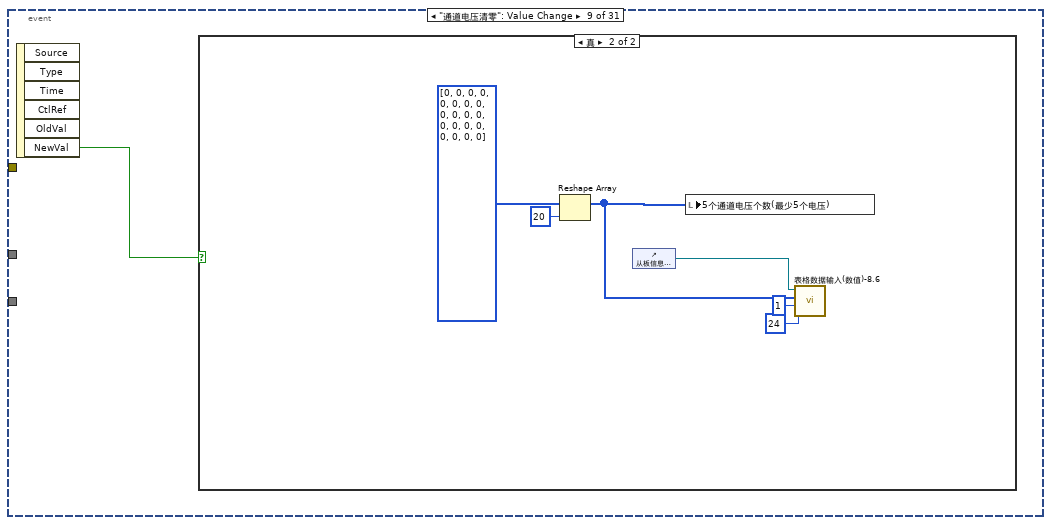
[diagram p17: hidden frame]
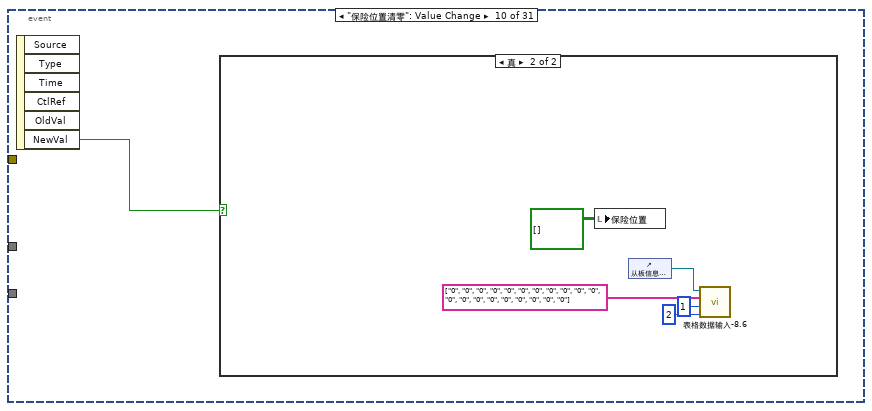
[diagram p19: hidden frame]
diagram:
  (unwired) T7 FALSE ("布尔")
  n1 = local write "输出数组"(string[][] [] ("输出数组")) -> ()
  n2 = local write "保险位置"(T6 [] ("保险位置")) -> ()
  n3 = local write "从板信息电压温度通道配置"(string[][] [["电压个数", ""], ["温度个数", ""], ["第一个保险通道", "0"], ["第一个保险位置", "0"], ["第二个保险通道", "0"], ["第二个保险位置", "0"], ["第三个保险通道", "0"], ["第三个保险位置", "0"], ["第四个保险通道", "0"], ["第四个保险位置", "0"], ["第五个保险通道", "0"], ["第五个保险位置", "0"], ["第六个保险通道", "0"], ["第六个保险位置", "0"], ["第七个保险通道", "0"], ["第七个保险位置", "0"], ["第八个保险通道", "0"], ["第八个保险位置", "0"], ["第九个保险通道", "0"], ["第九个保险位置", "0"], ["第十个保险通道", "0"], ["第十个保险位置", "0"], ["第1通道电压个数", ""], ["第2通道电压个数", ""], ["第3通道电压个数", ""], ["第4通道电压个数", ""], ["第5通道电压个数", ""]] ("从板信息电压温度通道配置")) -> ()
  n4 = Array Subset(array=string[] ["从板板号", "电压个数", "温度个数", "第一个保险通道", "第一个保险位置", "第二个保险通道", "第二个保险位置", "第三个保险通道", "第三个保险位置", "第四个保险通道", "第四个保险位置", "第五个保险通道", "第五个保险位置", "第六个保险通道", "第六个保险位置", "第七个保险通道", "第七个保险位置", "第八个保险通道", "第八个保险位置", "第九个保险通道", "第九个保险位置", "第十个保险通道", "第十个保险位置", "第1通道电压个数", "第2通道电压个数", "第3通道电压个数", "第4通道电压个数", "第5通道电压个数", "风机开启温度", "风机关闭温度", "加热开启温度", "加热关闭温度", "风机开启温差", "风机关闭温差", "加热关闭温差", "电压过高一级", "电压过低一级", "温度过高一级", "温度过低一级", "电压不均衡一级", "温度不均衡一级", "SOC过低一级", "电压过高二级", "电压过低二级", "温度过高二级", "温度过低二级", "电压不均衡二级", "温度不均衡二级", "SOC过低二级", "电压过高三级", "电压过低三级", "温度过高三级", "温度过低三级", "电压不均衡三级", "温度不均衡三级", "SOC过低三级", "均衡计算-电压高阀值1级", "均衡计算-电压高阀值2级", "均衡计算-电压低阀值1级", "均衡计算-电压低阀值2级", "均衡计算-最低电压阀值", "均衡停止-最低电压阀值", "均衡计算-电压极差阀值", "充电结束电压(90%)", "充电结束电压(91%)", "充电结束电压(92%)", "充电结束电压(93%)", "充电结束电压(94%)", "充电结束电压(95%)", "充电结束电压(96%)", "充电结束电压(97%)", "充电结束电压(98%)", "充电结束电压(99%)", "充电结束电压(100%)"] ("从板表头"), index=0 ("索引"), length=55 ("长度")) -> (w1:string[])
  n5 = local write "从板表头"(w1) -> ()
  n6 = while {
    tunnel: "error in" -> [w11]
    tunnel: w1 -> [w10]
    tunnel: w1 -> [w9]
    stop <- w13 stop-if-true
    n7 = event shown="[16] \"写配置文件\": 值改变" {
      selector: _ -> [_ _ _ _ _ _ _ _ _ _ _ _ _ _ _ _ _ _ _ _ _ _ _ _ _ _ _ _ _ _ _]
      dyn-events: _ -> [_ _ _ _ _ _ _ _ _ _ _ _ _ _ _ _ _ _ _ _ _ _ _ _ _ _ _ _ _ _ _]
      timeout: 1000 -> [_ _ _ _ _ _ _ _ _ _ _ _ _ _ _ _ _ _ _ _ _ _ _ _ _ _ _ _ _ _ _]
      tunnel: [_ _ _ _ _ _ _ _ _ _ _ _ _ _ _ _ _ _ _ _ _ _ _ _ _ _ TRUE TRUE _ _ _] -> w13
      tunnel: w11 -> [_ _ _ _ _ _ _ _ _ _ _ _ _ _ _ _ _ _ _ _ _ w990 w1185 _ _ _ _ _ _ _ _]
      tunnel: w10 -> [_ _ _ _ _ _ _ _ _ _ _ _ _ _ _ _ _ w548 _ _ _ _ w1184 _ _ _ _ _ _ _ _]
      tunnel: w9 -> [_ _ _ _ _ _ _ _ _ _ _ _ w215 _ _ _ w371 _ _ _ _ _ _ _ w1388 _ _ _ _ _ _]
      event "单个写入": Value Change {
        n8 = event-data() -> ("NewVal"=w14:bool)  [unwired: 1 in, 5 out]
        n9 = case shown="真" w14 {
          frame False {
          }
          frame True {
            n10 = local read "主板信息"() -> (w16:string[][])
            n11 = local read "从板个数"() -> (w19:dbl)
            n12 = call "主板信息配置.vi"("从板个数"=w19, "主板信息查看"=w16) -> ("输出数组"=w18:string[][], "布尔"=w15:bool, "从板个数 2"=w17:dbl)  [unwired: 1 in]
            n13 = case shown="真" w15 {
              tunnel: w18 -> [_ w21]
              tunnel: w17 -> [_ w20]
              frame False {
              }
              frame True {
                n14 = local write "从板个数"(w20) -> ()
                n15 = local write "主板信息"(w21) -> ()
              }
            }
          }
        }
      }
      event "读从板信息": Value Change {
        n16 = event-data() -> ("NewVal"=w22:bool)  [unwired: 1 in, 5 out]
        n17 = case shown="真" w22 {
          frame False {
          }
          frame True {
            n18 = local read "从板信息电压温度通道配置"() -> (w24:string[][])
            n19 = call "从板信息配置.vi"("从板信息查看"=w24) -> ("输出数组"=w25:string[][], "布尔"=w23:bool)  [unwired: 1 in]
            n20 = case shown="真" w23 {
              tunnel: w25 -> [_ w26]
              frame False {
              }
              frame True {
                n21 = local write "从板信息电压温度通道配置"(w26) -> ()
              }
            }
          }
        }
      }
      event "均衡参数设置": Value Change {
        n22 = event-data() -> ("NewVal"=w27:bool)  [unwired: 1 in, 5 out]
        n23 = case shown="真" w27 {
          frame False {
          }
          frame True {
            n24 = local read "均衡参数"() -> (w29:T1)
            n25 = call "均衡参数输入.vi"("均衡参数"=w29) -> ("均衡参数 2"=→"均衡参数":T1)
          }
        }
      }
      event "自动计算通道电压": Value Change {
        n26 = event-data() -> ("NewVal"=w30:bool)  [unwired: 1 in, 5 out]
        n27 = case shown="真" w30 {
          frame False {
          }
          frame True {
            n28 = local read "从板信息电压温度通道配置"() -> (w35:string[][])
            n29 = Index Array(array=w35, index (col)=1 ("禁用的索引 (列)")) -> (element=w41:string[])  [unwired: 1 in]
            n30 = Index Array(array=w41, index=0 ("索引")) -> (element=w39:string)
            n31 = Decimal String To Number(string=w39) -> (number=w38:i32)  [unwired: 2 in, 1 out]
            n32 = while {
              shift-right: [w49] -> _
              shift-left: w38 -> [w44]
              tunnel: [w47] -> w37 mode=indexing
              i -> [w56]
              stop <- w50 stop-if-true
              w46 = 12 ("y")
              n33 = local read "保险位置"() -> (w43:T6)
              n34 = Subtract(x=w44, y=w46) -> (x-y=w52:i32)
              n35 = Less?(x=w44, y=w46) -> (x < y?=w45:bool)
              n36 = Index Array(array=w43, index (row)=w56) -> (element=w55:T7[])  [unwired: 1 in]
              n37 = for {
                N: 12 -> [_]
                tunnel: w55 -> [w65] mode=indexing
                shift-right: [w66] -> w48
                shift-left: 0 -> [w63]
                n38 = Increment(x=w63) -> (x+1=w64:i32)
                n39 = Select(t=w64, s=w65, f=w63) -> (s? t:f=w66:i32)
              }
              n40 = Add(x=w52, y=w48) -> (x+y=w49:i32)
              n41 = case shown="真" w45 {
                tunnel: w48 -> [w59 w62]
                tunnel: [w58 w60] -> w47
                tunnel: w46 -> [w57 _]
                tunnel: w44 -> [_ w61]
                frame False {
                  n42 = Subtract(x=w57, y=w59) -> (x-y=w58:i32)
                }
                frame True {
                  n43 = Subtract(x=w61, y=w62) -> (x-y=w60:i32)
                }
              }
              n44 = Less Or Equal?(x=w49, y=0) -> (x <= y?=w50:bool)
            }
            n45 = Reshape Array(w37, 20 ("维数大小")) -> (w33:i32[])
            n46 = local write "5个通道电压个数(最少5个电压)"(w33) -> ()
            n47 = control-ref of="从板信息电压温度通道配置"() -> (w34:refnum<vi>)
            n48 = call "表格数据输入(数值)-8.6.vi"("行数"=u32 24, "列数"=u32 1, "数值数组"=w33, "表格引用"=w34) -> ()  [unwired: 8 in]
          }
        }
      }
      event Value Change {
        n49 = event-data() -> ("NewVal"=w71:T6)  [unwired: 1 in, 5 out]
        n50 = call "保险位置计算器.vi"("保险位置"=w71) -> ("输出数组"=w73:i32[])
        n51 = for {
          N: 20 -> [_]
          tunnel: w73 -> [w75] mode=indexing
          tunnel: [w74] -> w69 mode=indexing
          n52 = Number To Decimal String(number=w75) -> (decimal integer string=w74:string)  [unwired: 1 in]
        }
        n53 = control-ref of="从板信息电压温度通道配置"() -> (w70:refnum<vi>)
        n54 = call "表格数据输入-8.6.vi"("行数"=u32 2, "列数"=u32 1, "字符串数组"=w69, "表格引用"=w70) -> ()  [unwired: 8 in]
      }
      event "5个通道电压个数(最少5个电压)": Value Change {
        n55 = event-data() -> ()  [unwired: 1 in, 6 out]
        n56 = local read "5个通道电压个数(最少5个电压)"() -> (w76:u8[])
        n57 = for {
          N: 5 -> [_]
          tunnel: w76 -> [w83] mode=indexing
          tunnel: [w82] -> w79 mode=indexing
          n58 = Number To Decimal String(number=w83) -> (decimal integer string=w82:string)  [unwired: 1 in]
        }
        n59 = control-ref of="从板信息电压温度通道配置"() -> (w80:refnum<vi>)
        n60 = call "表格数据输入-8.6.vi"("行数"=u32 22, "列数"=u32 1, "字符串数组"=w79, "表格引用"=w80) -> ()  [unwired: 8 in]
      }
      event "电压个数": Value Change {
        n61 = event-data() -> ()  [unwired: 1 in, 6 out]
        n62 = local read "电压个数"() -> (w84:dbl)
        n63 = for {
          N: 1 -> [_]
          tunnel: w84 -> [w91]
          tunnel: [w90] -> w87 mode=indexing
          n64 = Number To Decimal String(number=w91) -> (decimal integer string=w90:string)  [unwired: 1 in]
        }
        n65 = control-ref of="从板信息电压温度通道配置"() -> (w88:refnum<vi>)
        n66 = call "表格数据输入-8.6.vi"("行数"=u32 0, "列数"=u32 1, "字符串数组"=w87, "表格引用"=w88) -> ()  [unwired: 8 in]
      }
      event "温度个数": Value Change {
        n67 = event-data() -> ()  [unwired: 1 in, 6 out]
        n68 = local read "温度个数"() -> (w92:dbl)
        n69 = for {
          N: 1 -> [_]
          tunnel: w92 -> [w99]
          tunnel: [w98] -> w95 mode=indexing
          n70 = Number To Decimal String(number=w99) -> (decimal integer string=w98:string)  [unwired: 1 in]
        }
        n71 = control-ref of="从板信息电压温度通道配置"() -> (w96:refnum<vi>)
        n72 = call "表格数据输入-8.6.vi"("行数"=u32 1, "列数"=u32 1, "字符串数组"=w95, "表格引用"=w96) -> ()  [unwired: 8 in]
      }
      event "通道电压清零": Value Change {
        n73 = event-data() -> ("NewVal"=w100:bool)  [unwired: 1 in, 5 out]
        n74 = case shown="真" w100 {
          frame False {
          }
          frame True {
            n75 = Reshape Array(u8[] [0, 0, 0, 0, 0, 0, 0, 0, 0, 0, 0, 0, 0, 0, 0, 0, 0, 0, 0, 0] ("20个通道电压个数"), 20 ("维数大小")) -> (w101:u8[])
            n76 = control-ref of="从板信息电压温度通道配置"() -> (w104:refnum<vi>)
            n77 = local write "5个通道电压个数(最少5个电压)"(w101) -> ()
            n78 = call "表格数据输入(数值)-8.6.vi"("行数"=u32 24, "列数"=u32 1, "数值数组"=w101, "表格引用"=w104) -> ()  [unwired: 8 in]
          }
        }
      }
      event "保险位置清零": Value Change {
        n79 = event-data() -> ("NewVal"=w107:bool)  [unwired: 1 in, 5 out]
        n80 = case shown="真" w107 {
          frame False {
          }
          frame True {
            n81 = local write "保险位置"(bool[][] [] ("保险位置")) -> ()
            n82 = control-ref of="从板信息电压温度通道配置"() -> (w111:refnum<vi>)
            n83 = call "表格数据输入-8.6.vi"("行数"=u32 2, "列数"=u32 1, "字符串数组"=string[] ["0", "0", "0", "0", "0", "0", "0", "0", "0", "0", "0", "0", "0", "0", "0", "0", "0", "0", "0", "0"], "表格引用"=w111) -> ()  [unwired: 8 in]
          }
        }
      }
      event Value Change {
        n84 = event-data() -> ("NewVal"=w113:T5)  [unwired: 1 in, 5 out]
        n85 = case shown="真" w113 {
          frame False {
          }
          frame True {
            n86 = local read "从板信息电压温度通道配置"() -> (w136:string[][])
            n87 = local read "一级故障 2"() -> (w133:dbl[][])
            n88 = local read "均衡参数"() -> (w115:T1)
            n89 = local read "加热控制参数 2"() -> (w135:T3)
            n90 = Transpose 2D Array(2D array=w133) -> (transposed array=w120:dbl[][])
            n91 = Cluster To Array(cluster=w115) -> (array=w114:sgl[])
            n92 = Array Subset(array=w136, index (row)=0 ("索引"), index (col)=0 ("索引"), length (col)=2 ("索引")) -> (w131:string[][])  [unwired: 1 in]
            n93 = for {
              tunnel: w120 -> [w155] mode=indexing
              shift-right: [w154] -> w129
              shift-left: string[] [] -> [w152]
              n94 = for {
                N: 7 -> [_]
                tunnel: w155 -> [w158] mode=indexing
                tunnel: [w156] -> w153 mode=indexing
                n95 = Format Into String(format string="%#f" ("格式字符串"), w158) -> (resulting string=w156:string)  [unwired: 2 in, 1 out]
              }
              n96 = Insert Into Array(array=w152, new element=w153) -> (w154:string[])  [unwired: 1 in]
            }
            n97 = Cluster To Array(cluster=w135) -> (array=w134:dbl[])
            n98 = for {
              tunnel: w114 -> [w142] mode=indexing
              tunnel: [w140] -> _ mode=indexing
              n99 = Format Into String(format string="%#f" ("格式字符串"), w142) -> (resulting string=w140:string)  [unwired: 2 in, 1 out]
            }
            n100 = Index Array(array=w131, index (col) #2=1 ("索引 (列)")) -> (element #2=w117:string[])  [unwired: 3 in, 1 out]
            n101 = for {
              tunnel: w134 -> [w161] mode=indexing
              tunnel: [w159] -> w130 mode=indexing
              n102 = Format Into String(format string="%#f" ("格式字符串"), w161) -> (resulting string=w159:string)  [unwired: 2 in, 1 out]
            }
            n103 = local read "从板板号"() -> (w124:dbl)
            n104 = Array Subset(array=w117, length=27 ("长度")) -> (w118:string[])  [unwired: 1 in]
            n105 = Number To Decimal String(number=w124) -> (decimal integer string=w122:string)  [unwired: 1 in]
            n106 = Insert Into Array(array=w118, new element #1=w130, new element #2=w129) -> (w128:string[])  [unwired: 1 in]
            n107 = Decrement(x=w124) -> (x-1=w119:dbl)
            n108 = local read "输出数组"() -> (w126:string[][])
            n109 = Insert Into Array(array=w128, index=0 ("索引"), new element=w122) -> (w125:string[])
            n110 = Replace Array Subset(array=w126, new element=w125, index (col)=w119) -> (w123:string[][])  [unwired: 1 in]
            n111 = stacked-sequence {
              tunnel: w123 -> [w143]
              tunnel: w122 -> [w148]
              frame #0 {
                n112 = control-ref of="结果"() -> (w150:refnum<vi>)
                n113 = Concatenate Strings("从板", w148, "保存成功") -> (w146:string)
                n114 = local write "输出数组"(w143) -> ()
                n115 = Build Array(w146) -> (w144:string[])
                n116 = call "表格编辑.vi"("新元素/子数组"=w144, "活动单元格:单元格背景色"=u32 6618880, "MCListbox引用句柄"=w150) -> ()  [unwired: 9 in]
              }
            }
          }
        }
      }
      event "全部记录": Value Change {
        n117 = event-data() -> ("NewVal"=w162:bool)  [unwired: 1 in, 5 out]
        n118 = case shown="真" w162 {
          frame False {
          }
          frame True {
            n119 = local read "从板个数"() -> (w166:dbl)
            n120 = for {
              N: w166 -> [_]
              tunnel: [w174] -> w165 mode=indexing
              i -> [w175]
              n121 = local read "从板信息电压温度通道配置"() -> (w190:string[][])
              n122 = local read "一级故障 2"() -> (w187:dbl[][])
              n123 = local read "加热控制参数 2"() -> (w189:T3)
              n124 = local read "均衡参数"() -> (w170:T1)
              n125 = Transpose 2D Array(2D array=w187) -> (transposed array=w178:dbl[][])
              n126 = Array Subset(array=w190, index (row)=0 ("索引"), index (col)=0 ("索引"), length (col)=2 ("索引")) -> (w185:string[][])  [unwired: 1 in]
              n127 = for {
                tunnel: w178 -> [w208] mode=indexing
                shift-right: [w207] -> w182
                shift-left: string[] [] -> [w205]
                n128 = for {
                  N: 7 -> [_]
                  tunnel: w208 -> [w211] mode=indexing
                  tunnel: [w209] -> w206 mode=indexing
                  n129 = Format Into String(format string="%#f" ("格式字符串"), w211) -> (resulting string=w209:string)  [unwired: 2 in, 1 out]
                }
                n130 = Insert Into Array(array=w205, new element=w206) -> (w207:string[])  [unwired: 1 in]
              }
              n131 = Cluster To Array(cluster=w170) -> (array=w169:sgl[])
              n132 = Cluster To Array(cluster=w189) -> (array=w188:dbl[])
              n133 = Index Array(array=w185, index (col) #1=0 ("禁用的索引 (列)"), index (col) #2=1 ("索引 (列)")) -> (element #2=w172:string[])  [unwired: 2 in, 1 out]
              n134 = for {
                tunnel: w188 -> [w214] mode=indexing
                tunnel: [w212] -> w183 mode=indexing
                n135 = Format Into String(format string="%#f" ("格式字符串"), w214) -> (resulting string=w212:string)  [unwired: 2 in, 1 out]
              }
              n136 = for {
                tunnel: w169 -> [w196] mode=indexing
                tunnel: [w194] -> w168 mode=indexing
                n137 = Format Into String(format string="%#f" ("格式字符串"), w196) -> (resulting string=w194:string)  [unwired: 2 in, 1 out]
              }
              n138 = Array Subset(array=w172, length=44 ("长度")) -> (w173:string[])  [unwired: 1 in]
              n139 = Increment(x=w175) -> (x+1=w177:i32)
              n140 = Number To Decimal String(number=w177) -> (decimal integer string=w180:string)  [unwired: 1 in]
              n141 = Insert Into Array(array=w173, new element #1=w183, new element #2=w182, new element #3=w168) -> (w181:string[])  [unwired: 1 in]
              n142 = stacked-sequence {
                tunnel: w180 -> [w201]
                frame #0 {
                  n143 = control-ref of="结果"() -> (w203:refnum<vi>)
                  n144 = Concatenate Strings("从板", w201, "记录完成") -> (w199:string)
                  n145 = Build Array(w199) -> (w197:string[])
                  n146 = call "表格编辑.vi"("新元素/子数组"=w197, "活动单元格:单元格背景色"=u32 6618880, "MCListbox引用句柄"=w203) -> ()  [unwired: 9 in]
                }
              }
              n147 = Insert Into Array(array=w181, index=0 ("索引"), new element=w180) -> (w174:string[])
            }
            n148 = local write "从板表头"(string[] ["从板板号", "电压个数", "电压起始值", "温度个数", "温度起始值", "第一个保险通道", "第一个保险位置", "第二个保险通道", "第二个保险位置", "第三个保险通道", "第三个保险位置", "第四个保险通道", "第四个保险位置", "第五个保险通道", "第五个保险位置", "第六个保险通道", "第六个保险位置", "第七个保险通道", "第七个保险位置", "第八个保险通道", "第八个保险位置", "第九个保险通道", "第九个保险位置", "第十个保险通道", "第十个保险位置", "第1通道电压个数", "第2通道电压个数", "第3通道电压个数", "第4通道电压个数", "第5通道电压个数", "第6通道电压个数", "第7通道电压个数", "第8通道电压个数", "第9通道电压个数", "第10通道电压个数", "第11通道电压个数", "第12通道电压个数", "第13通道电压个数", "第14通道电压个数", "第15通道电压个数", "第16通道电压个数", "第17通道电压个数", "第18通道电压个数", "第19通道电压个数", "第20通道电压个数", "风机开启温度", "风机关闭温度", "加热开启温度", "加热关闭温度", "风机开启温差", "风机关闭温差", "加热关闭温差", "电压过高一级", "电压过低一级", "温度过高一级", "温度过低一级", "电压不均衡一级", "温度不均衡一级", "SOC过低一级", "电压过高二级", "电压过低二级", "温度过高二级", "温度过低二级", "电压不均衡二级", "温度不均衡二级", "SOC过低二级", "电压过高三级", "电压过低三级", "温度过高三级", "温度过低三级", "电压不均衡三级", "温度不均衡三级", "SOC过低三级", "均衡计算-电压高阀值1级", "均衡计算-电压高阀值2级", "均衡计算-电压低阀值1级", "均衡计算-电压低阀值2级", "均衡计算-最低电压阀值", "均衡停止-最低电压阀值", "均衡计算-电压极差阀值", "充电结束电压(90%)", "充电结束电压(91%)", "充电结束电压(92%)", "充电结束电压(93%)", "充电结束电压(94%)", "充电结束电压(95%)", "充电结束电压(96%)", "充电结束电压(97%)", "充电结束电压(98%)", "充电结束电压(99%)", "充电结束电压(100%)"] ("从板表头")) -> ()
            n149 = property on="查看" class="Bool (严格)"("Visible"=TRUE ("可见")) -> ()  [unwired: 2 in, 2 out]
            n150 = Transpose 2D Array(2D array=w165) -> (transposed array=w164:string[][])
            n151 = local write "输出数组"(w164) -> ()
          }
        }
      }
      event "主从板": Value Change {
        n152 = event-data() -> ()  [unwired: 1 in, 6 out]
        n153 = control-ref of="单选选项2"() -> (w221:refnum<vi>)
        n154 = control-ref of="单选选项1"() -> (w220:refnum<vi>)
        n155 = local read "主从板"() -> (w216:enum32{"单选选项2", "单选选项1"})
        n156 = case shown="\"单选选项2\"" w216 {
          tunnel: w215 -> [w225 _]
          frame "单选选项2" {
            n157 = case shown="假" TRUE {
              tunnel: w225 -> [w227 _]
              frame False {
                n158 = stacked-sequence {
                  seq-local: [w231 _] -> [_ _]
                  seq-local: [w230 _] -> [_ w299]
                  tunnel: w227 -> [_ w291]
                  frame #0 {
                    n159 = local read "主板信息"() -> (w237:string[][])
                    n160 = local read "从板个数"() -> (w232:dbl)
                    n161 = Index Array(array=w237, index (col) #1=0 ("禁用的索引 (列)"), index (col) #2=1 ("索引 (列)")) -> (element #1=w234:string[], element #2=w233:string[])  [unwired: 2 in]
                    n162 = for {
                      N: w232 -> [_]
                      tunnel: w234 -> [w273]
                      tunnel: w233 -> [w265]
                      tunnel: [w250] -> w229
                      tunnel: [w257] -> w228
                      i -> [w250]
                      n163 = Cluster To Array(cluster=T8 {"风机开启温度(℃)"=35.0, "风机关闭温度(℃)"=30.0, "加热开启温度(℃)"=0.0, "加热关闭温度(℃)"=5.0, "风机开启温差(℃)"=5.0, "风机开启温度(℃)"=3.0, "加热关闭温差(℃)"=10.0} ("加热控制参数")) -> (array=w252:dbl[])
                      n164 = local read "输出数组"() -> (w251:string[][])
                      n165 = Transpose 2D Array(2D array=dbl[][] [[4.23, 4.25, 4.3], [3.0, 2.75, 2.5], [50.0, 55.0, 60.0], [-20.0, -30.0, -40.0], [0.5, 1.0, 1.5], [25.0, 30.0, 35.0], [30.0, 20.0, 10.0]] ("一级故障 2")) -> (transposed array=w253:dbl[][])
                      n166 = Search 1D Array(1D array=w273, element="从板1电池节数" ("元素")) -> (index of element=w270:i32)  [unwired: 1 in]
                      n167 = Search 1D Array(1D array=w273, element="从板1电压起始值" ("元素")) -> (index of element=w268:i32)  [unwired: 1 in]
                      n168 = Search 1D Array(1D array=w273, element="从板1温度个数" ("元素")) -> (index of element=w264:i32)  [unwired: 1 in]
                      n169 = Search 1D Array(1D array=w273, element="从板1温度起始值" ("元素")) -> (index of element=w263:i32)  [unwired: 1 in]
                      n170 = for {
                        tunnel: w252 -> [w290] mode=indexing
                        tunnel: [w288] -> w245 mode=indexing
                        n171 = Format Into String(format string="%#f" ("格式字符串"), w290) -> (resulting string=w288:string)  [unwired: 2 in, 1 out]
                      }
                      n172 = for {
                        tunnel: w253 -> [w284] mode=indexing
                        shift-right: [w283] -> w241
                        shift-left: _ -> [w281]
                        n173 = for {
                          N: 7 -> [_]
                          tunnel: w284 -> [w287] mode=indexing
                          tunnel: [w285] -> w282 mode=indexing
                          n174 = Format Into String(format string="%#f" ("格式字符串"), w287) -> (resulting string=w285:string)  [unwired: 2 in, 1 out]
                        }
                        n175 = Insert Into Array(array=w281, new element=w282) -> (w283:string[])  [unwired: 1 in]
                      }
                      n176 = Add(x=w270, y=w250) -> (x+y=w271:i32)
                      n177 = Add(x=w268, y=w250) -> (x+y=w269:i32)
                      n178 = Add(x=w263, y=w250) -> (x+y=w266:i32)
                      n179 = Add(x=w264, y=w250) -> (x+y=w267:i32)
                      n180 = Index Array(array=w251, index (col)=w250) -> (element=w249:string[])  [unwired: 1 in]
                      n181 = Index Array(array=w265, index=w271) -> (element=w262:string)
                      n182 = Index Array(array=w265, index=w269) -> ()  [unwired: 1 out]
                      n183 = Index Array(array=w265, index=w266) -> ()  [unwired: 1 out]
                      n184 = Index Array(array=w265, index=w267) -> (element=w261:string)
                      n185 = local read "均衡参数"() -> (w244:T1)
                      n186 = Array Subset(array=w249, index=3 ("索引"), length=27 ("长度")) -> (w246:string[])
                      n187 = Increment(x=w250) -> (x+1=w256:i32)
                      n188 = Number To Decimal String(number=w256) -> (decimal integer string=w260:string)  [unwired: 1 in]
                      n189 = Cluster To Array(cluster=w244) -> (array=w243:sgl[])
                      n190 = local read "输出数组"() -> (w259:string[][])
                      n191 = for {
                        tunnel: w243 -> [w279] mode=indexing
                        tunnel: [w277] -> w242 mode=indexing
                        n192 = Format Into String(format string="%#f" ("格式字符串"), w279) -> (resulting string=w277:string)  [unwired: 2 in, 1 out]
                      }
                      n193 = Build Array (concatenate)(w260, w262, w261, w246, w245, w241, w242) -> (w258:string[])
                      n194 = Replace Array Subset(array=w259, new element=w258, index (col)=w250) -> (w257:string[][])  [unwired: 1 in]
                      n195 = local write "输出数组"(w257) -> ()
                    }
                    n196 = stacked-sequence {
                      tunnel: [w238] -> w231
                      tunnel: [w239] -> w230
                      tunnel: w229 -> [_]
                      tunnel: w228 -> [w239]
                      frame #0 {
                        n197 = disable-structure shown="禁用" {
                          disable-tunnel: [w240 _] -> w238
                          frame Disabled {
                            w240 = string[] ["从板板号", "电压个数", "温度个数", "第一个保险通道", "第一个保险位置", "第二个保险通道", "第二个保险位置", "第三个保险通道", "第三个保险位置", "第四个保险通道", "第四个保险位置", "第五个保险通道", "第五个保险位置", "第六个保险通道", "第六个保险位置", "第七个保险通道", "第七个保险位置", "第八个保险通道", "第八个保险位置", "第九个保险通道", "第九个保险位置", "第十个保险通道", "第十个保险位置", "第1通道电压个数", "第2通道电压个数", "第3通道电压个数", "第4通道电压个数", "第5通道电压个数", "风机开启温度", "风机关闭温度", "加热开启温度", "加热关闭温度", "风机开启温差", "风机关闭温差", "加热关闭温差", "电压过高一级", "电压过低一级", "温度过高一级", "温度过低一级", "电压不均衡一级", "温度不均衡一级", "SOC过低一级", "电压过高二级", "电压过低二级", "温度过高二级", "温度过低二级", "电压不均衡二级", "温度不均衡二级", "SOC过低二级", "电压过高三级", "电压过低三级", "温度过高三级", "温度过低三级", "电压不均衡三级", "温度不均衡三级", "SOC过低三级", "均衡计算-电压高阀值1级", "均衡计算-电压高阀值2级", "均衡计算-电压低阀值1级", "均衡计算-电压低阀值2级", "均衡计算-最低电压阀值", "均衡停止-最低电压阀值", "均衡计算-电压极差阀值", "充电结束电压(90%)", "充电结束电压(91%)", "充电结束电压(92%)", "充电结束电压(93%)", "充电结束电压(94%)", "充电结束电压(95%)", "充电结束电压(96%)", "充电结束电压(97%)", "充电结束电压(98%)", "充电结束电压(99%)", "充电结束电压(100%)"] ("从板表头")
                            n198 = local write "从板表头"(w240) -> ()
                          }
                          frame Enabled {
                          }
                        }
                      }
                    }
                  }
                  frame #1 {
                    (unwired) string[] ["从板板号", "电压个数", "电压起始值", "温度个数", "温度起始值", "第一个保险通道", "第一个保险位置", "第二个保险通道", "第二个保险位置", "第三个保险通道", "第三个保险位置", "第四个保险通道", "第四个保险位置", "第五个保险通道", "第五个保险位置", "第六个保险通道", "第六个保险位置", "第七个保险通道", "第七个保险位置", "第八个保险通道", "第八个保险位置", "第九个保险通道", "第九个保险位置", "第十个保险通道", "第十个保险位置", "第1通道电压个数", "第2通道电压个数", "第3通道电压个数", "第4通道电压个数", "第5通道电压个数", "第6通道电压个数", "第7通道电压个数", "第8通道电压个数", "第9通道电压个数", "第10通道电压个数", "第11通道电压个数", "第12通道电压个数", "第13通道电压个数", "第14通道电压个数", "第15通道电压个数", "第16通道电压个数", "第17通道电压个数", "第18通道电压个数", "第19通道电压个数", "第20通道电压个数", "风机开启温度", "风机关闭温度", "加热开启温度", "加热关闭温度", "风机开启温差", "风机关闭温差", "加热关闭温差", "电压过高一级", "电压过低一级", "温度过高一级", "温度过低一级", "电压不均衡一级", "温度不均衡一级", "SOC过低一级", "电压过高二级", "电压过低二级", "温度过高二级", "温度过低二级", "电压不均衡二级", "温度不均衡二级", "SOC过低二级", "电压过高三级", "电压过低三级", "温度过高三级", "温度过低三级", "电压不均衡三级", "温度不均衡三级", "SOC过低三级", "均衡计算-电压高阀值1级", "均衡计算-电压高阀值2级", "均衡计算-电压低阀值1级", "均衡计算-电压低阀值2级", "均衡计算-最低电压阀值", "均衡停止-最低电压阀值", "均衡计算-电压极差阀值", "充电结束电压(90%)", "充电结束电压(91%)", "充电结束电压(92%)", "充电结束电压(93%)", "充电结束电压(94%)", "充电结束电压(95%)", "充电结束电压(96%)", "充电结束电压(97%)", "充电结束电压(98%)", "充电结束电压(99%)", "充电结束电压(100%)"] ("从板表头")
                    n199 = local read "从板板号"() -> (w298:dbl)
                    n200 = Decrement(x=w298) -> (x-1=w297:dbl)
                    n201 = Search 1D Array(1D array=w291, element="风机开启温度" ("元素")) -> (index of element=w319:i32)  [unwired: 1 in]
                    n202 = Search 1D Array(1D array=w291, element="电压过高一级" ("元素"), start index (0)=w319) -> (index of element=w317:i32)
                    n203 = Index Array(array=w299, index (col)=w297) -> (element=w296:string[])  [unwired: 1 in]
                    n204 = Decrement(x=w319) -> (x-1=w321:i32)
                    n205 = Array Subset(array=w296, index=1 ("索引"), length=w321) -> (w323:string[])
                    n206 = Array Subset(array=w296, index=w317, length=21 ("长度")) -> (w303:string[])
                    n207 = Array Subset(array=w296, index=w319, length=7 ("长度")) -> (w315:string[])
                    n208 = for {
                      tunnel: w303 -> [w327] mode=indexing
                      tunnel: [w326] -> w302 mode=indexing
                      n209 = Fract/Exp String To Number(string=w327) -> (number=w326:dbl)  [unwired: 3 in, 1 out]
                    }
                    n210 = for {
                      tunnel: w315 -> [w329] mode=indexing
                      tunnel: [w328] -> w300 mode=indexing
                      n211 = Fract/Exp String To Number(string=w329) -> (number=w328:dbl)  [unwired: 3 in, 1 out]
                    }
                    n212 = Array Subset(array=string[] ["从板板号", "电压个数", "温度个数", "第一个保险通道", "第一个保险位置", "第二个保险通道", "第二个保险位置", "第三个保险通道", "第三个保险位置", "第四个保险通道", "第四个保险位置", "第五个保险通道", "第五个保险位置", "第六个保险通道", "第六个保险位置", "第七个保险通道", "第七个保险位置", "第八个保险通道", "第八个保险位置", "第九个保险通道", "第九个保险位置", "第十个保险通道", "第十个保险位置", "第1通道电压个数", "第2通道电压个数", "第3通道电压个数", "第4通道电压个数", "第5通道电压个数", "第6通道电压个数", "第7通道电压个数", "第8通道电压个数", "第9通道电压个数", "第10通道电压个数", "第11通道电压个数", "第12通道电压个数", "第13通道电压个数", "第14通道电压个数", "第15通道电压个数", "第16通道电压个数", "第17通道电压个数", "第18通道电压个数", "第19通道电压个数", "第20通道电压个数", "风机开启温度", "风机关闭温度", "加热开启温度", "加热关闭温度", "风机开启温差", "风机关闭温差", "加热关闭温差", "电压过高一级", "电压过低一级", "温度过高一级", "温度过低一级", "电压不均衡一级", "温度不均衡一级", "SOC过低一级", "电压过高二级", "电压过低二级", "温度过高二级", "温度过低二级", "电压不均衡二级", "温度不均衡二级", "SOC过低二级", "电压过高三级", "电压过低三级", "温度过高三级", "温度过低三级", "电压不均衡三级", "温度不均衡三级", "SOC过低三级", "均衡计算-电压高阀值1级", "均衡计算-电压高阀值2级", "均衡计算-电压低阀值1级", "均衡计算-电压低阀值2级", "均衡计算-最低电压阀值", "均衡停止-最低电压阀值", "均衡计算-电压极差阀值", "充电结束电压(90%)", "充电结束电压(91%)", "充电结束电压(92%)", "充电结束电压(93%)", "充电结束电压(94%)", "充电结束电压(95%)", "充电结束电压(96%)", "充电结束电压(97%)", "充电结束电压(98%)", "充电结束电压(99%)", "充电结束电压(100%)"] ("从板表头"), index=1 ("长度"), length=27 ("长度")) -> (w292:string[])
                    n213 = Delete From Array(array=w302, length=7 ("长度"), index=0 ("索引")) -> (deleted portion=w311:dbl[], array with subset deleted=w310:dbl[])
                    n214 = Build Array(w292, w323) -> (w322:string[][])
                    n215 = Array To Cluster(array=w300) -> (cluster=w314:T10)
                    n216 = Delete From Array(array=w310, length=7 ("长度"), index=0 ("索引")) -> (deleted portion=w307:dbl[], array with subset deleted=w306:dbl[])
                    n217 = Transpose 2D Array(2D array=w322) -> (transposed array=w301:string[][])
                    n218 = local write "加热控制参数 2"(w314) -> ()
                    n219 = Build Array(w311, w307, w306) -> (w305:dbl[][])
                    n220 = local write "从板信息电压温度通道配置"(w301) -> ()
                    n221 = Transpose 2D Array(2D array=w305) -> (transposed array=w304:dbl[][])
                    n222 = local write "一级故障 2"(w304) -> ()
                  }
                }
              }
              frame True {
              }
            }
          }
          frame "单选选项1", Default {
          }
        }
        n223 = Build Array(w220, w221) -> (w222:refnum<vi>[])
        n224 = case shown="\"单选选项2\", 默认" w216 {
          selector: w216 -> [w334 w339]
          tunnel: [enum32{"主板", "从板", "预览"}."从板" ("选项卡控件") enum32{"主板", "从板", "预览"}."主板" ("选项卡控件")] -> w219
          tunnel: w222 -> [w335 w340]
          tunnel: [w333 w338] -> w223
          tunnel: [w332 w337] -> w224
          frame "单选选项2", Default {
            n225 = Delete From Array(array=w335, index=w334) -> (deleted portion=w332:refnum<vi>, array with subset deleted=w333:refnum<vi>[])  [unwired: 1 in]
          }
          frame "单选选项1" {
            n226 = Delete From Array(array=w340, index=w339) -> (deleted portion=w337:refnum<vi>, array with subset deleted=w338:refnum<vi>[])  [unwired: 1 in]
          }
        }
        n227 = for {
          tunnel: u32 65511 -> [w331]
          tunnel: w223 -> [w330] mode=indexing
          n228 = property class="Bool (严格)"(reference=w330, "BoolText.TextColor"=w331) -> ()  [unwired: 1 in, 2 out]
        }
        n229 = local write "选项卡控件"(w219) -> ()
        n230 = property class="Bool (严格)"(reference=w224, "BoolText.TextColor"=u32 16119285) -> ()  [unwired: 1 in, 2 out]
      }
      event "默认值 2": Value Change {
        n231 = event-data() -> ("NewVal"=w342:bool)  [unwired: 1 in, 5 out]
        n232 = case shown="真" w342 {
          frame False {
          }
          frame True {
            n233 = local write "保险位置"(bool[][] [] ("保险位置")) -> ()
            n234 = local write "一级故障 2"(dbl[][] [[4.23, 4.25, 4.3], [3.0, 2.75, 2.5], [50.0, 55.0, 60.0], [-20.0, -30.0, -40.0], [0.5, 1.0, 1.5], [25.0, 30.0, 35.0], [30.0, 20.0, 10.0]] ("一级故障 2")) -> ()
            n235 = local write "加热控制参数 2"(T8 {"风机开启温度(℃)"=35.0, "风机关闭温度(℃)"=30.0, "加热开启温度(℃)"=0.0, "加热关闭温度(℃)"=5.0, "风机开启温差(℃)"=5.0, "风机开启温度(℃)"=3.0, "加热关闭温差(℃)"=10.0} ("加热控制参数")) -> ()
            n236 = Reshape Array(u8[] [0, 0, 0, 0, 0, 0, 0, 0, 0, 0, 0, 0, 0, 0, 0, 0, 0, 0, 0, 0] ("20个通道电压个数"), 5 ("维数大小")) -> (w347:u8[])
            n237 = local write "5个通道电压个数(最少5个电压)"(w347) -> ()
            n238 = control-ref of="从板信息电压温度通道配置"() -> (w343:refnum<vi>)
            n239 = call "表格数据输入-8.6.vi"("行数"=u32 4, "列数"=u32 1, "字符串数组"=string[] ["", "", "", "", "", "", "", "", "", "", "", "", "", "", "", "", "", ""], "表格引用"=w343) -> ()  [unwired: 8 in]
            n240 = call "表格数据输入(数值)-8.6.vi"("行数"=u32 22, "列数"=u32 1, "数值数组"=w347, "表格引用"=w343) -> ()  [unwired: 8 in]
          }
        }
      }
      event "全部清零(从板)": Value Change {
        n241 = event-data() -> ("NewVal"=w355:bool)  [unwired: 1 in, 5 out]
        n242 = case shown="真" w355 {
          frame False {
          }
          frame True {
            n243 = control-ref of="从板信息电压温度通道配置"() -> (w361:refnum<vi>)
            n244 = local write "一级故障 2"(dbl[][] [[0.0, 0.0, 0.0], [0.0, 0.0, 0.0], [0.0, 0.0, 0.0], [0.0, 0.0, 0.0], [0.0, 0.0, 0.0], [0.0, 0.0, 0.0], [0.0, 0.0, 0.0]] ("一级故障 2")) -> ()
            n245 = call "表格数据输入-8.6.vi"("行数"=u32 0, "列数"=u32 1, "字符串数组"=string[] ["", "", "", "", "", "", "", "", "", "", "", "", "", "", "", "", "", "", "", "", "", "", "", "", "", "", "", " "], "表格引用"=w361) -> ()  [unwired: 8 in]
            n246 = local write "加热控制参数 2"(T8 {"风机开启温度(℃)"=0.0, "风机关闭温度(℃)"=0.0, "加热开启温度(℃)"=0.0, "加热关闭温度(℃)"=0.0, "风机开启温差(℃)"=0.0, "风机开启温度(℃)"=0.0, "加热关闭温差(℃)"=0.0} ("加热控制参数")) -> ()
            n247 = Reshape Array(u8[] [0, 0, 0, 0, 0, 0, 0, 0, 0, 0, 0, 0, 0, 0, 0, 0, 0, 0, 0, 0] ("20个通道电压个数"), 20 ("维数大小")) -> (w357:u8[])
            n248 = local write "5个通道电压个数(最少5个电压)"(w357) -> ()
            n249 = local write "保险位置"(bool[][] [] ("保险位置")) -> ()
          }
        }
      }
      event "设电池信息主板": Value Change {
        n250 = event-data() -> ("NewVal"=w366:bool)  [unwired: 1 in, 5 out]
        n251 = case shown="真" w366 {
          frame False {
          }
          frame True {
            n252 = local read "电池信息"() -> (w368:string[][])
            n253 = call "主板电池信息配置.vi"("电池信息查看"=w368) -> ("输出数组"=w369:string[][], "布尔"=w367:bool)  [unwired: 1 in]
            n254 = case shown="真" w367 {
              tunnel: w369 -> [_ w370]
              frame False {
              }
              frame True {
                n255 = local write "电池信息"(w370) -> ()
              }
            }
          }
        }
      }
      event "写配置文件": Value Change {
        n256 = event-data() -> ("NewVal"=w372:bool)  [unwired: 1 in, 5 out]
        n257 = case shown="真" w372 {
          tunnel: w371 -> [_ w373]
          frame False {
          }
          frame True {
            n258 = for {
              N: 2 -> [_]
              tunnel: w373 -> [w376]
              i -> [w377]
              n259 = stacked-sequence {
                seq-local: [w405 _ _] -> [_ w461 _]
                seq-local: [w403 _ _] -> [_ w455 _]
                seq-local: [w401 _ _] -> [_ w457 _]
                seq-local: [_ w456 _] -> [_ _ w509]
                seq-local: [w400 _ _] -> [_ _ w508]
                seq-local: [_ w451 _] -> [_ _ w507]
                seq-local: [_ w450 _] -> [_ _ w506]
                tunnel: w377 -> [_ w449 _]
                tunnel: w377 -> [_ w448 w505]
                tunnel: w376 -> [_ _ w504]
                frame #0 {
                  n260 = local read "一级故障"() -> (w417:dbl[][])
                  n261 = local read "充电控制参数"() -> (w389:T4)
                  n262 = local read "主板信息"() -> (w418:string[][])
                  n263 = local read "电池信息"() -> (w408:string[][])
                  n264 = local read "加热控制参数"() -> (w414:T3)
                  n265 = Array Subset(array=w418, index (row)=0 ("索引"), index (col)=0 ("索引"), length (col)=2 ("索引")) -> (w420:string[][])  [unwired: 1 in]
                  n266 = Transpose 2D Array(2D array=w417) -> (transposed array=w399:dbl[][])
                  n267 = for {
                    tunnel: w399 -> [w434] mode=indexing
                    shift-right: [w433] -> w393
                    shift-left: string[] [] -> [w431]
                    n268 = for {
                      N: 17 -> [_]
                      tunnel: w434 -> [w437] mode=indexing
                      tunnel: [w435] -> w432 mode=indexing
                      n269 = Format Into String(format string="%#f" ("格式字符串"), w437) -> (resulting string=w435:string)  [unwired: 2 in, 1 out]
                    }
                    n270 = Insert Into Array(array=w431, new element=w432) -> (w433:string[])  [unwired: 1 in]
                  }
                  n271 = Unbundle(w389) -> ("最大允许单体电压(V)"=w388:dbl, "最大允许总电压(V)"=w384:dbl, "最小允许单体电压(V)"=w387:dbl, "最大允许充电电流(A)"=w386:dbl, "最小允许充电电流(A)"=w385:dbl, "最大允许充电温度(℃)"=w383:dbl, "最小允许充电温度(℃)"=w382:dbl, "电流步长"=w381:dbl)
                  n272 = Index Array(array=w420, index (col) #1=1 ("禁用的索引 (列)"), index (col) #2=0 ("索引 (列)")) -> (element #1=w398:string[], element #2=w403:string[])  [unwired: 2 in]
                  n273 = local read "从板个数"() -> (w400:dbl)
                  n274 = Array Subset(array=w408, index (row)=0 ("索引"), index (col)=0 ("索引"), length (col)=2 ("索引")) -> (w412:string[][])  [unwired: 1 in]
                  n275 = Cluster To Array(cluster=w414) -> (array=w415:dbl[])
                  n276 = local read "分流器型号"() -> (w379:T2)
                  n277 = for {
                    tunnel: w415 -> [w429] mode=indexing
                    tunnel: [w427] -> w397 mode=indexing
                    n278 = Format Into String(format string="%#f" ("格式字符串"), w429) -> (resulting string=w427:string)  [unwired: 2 in, 1 out]
                  }
                  n279 = Build Array(w388, w387, w386, w385, w384, w383, w382, w381) -> (w380:dbl[])
                  n280 = Index Array(array=w412, index (col) #1=0 ("禁用的索引 (列)"), index (col) #2=1 ("禁用的索引 (列)")) -> (element #1=w401:string[], element #2=w395:string[])  [unwired: 2 in]
                  n281 = for {
                    tunnel: w380 -> [w426] mode=indexing
                    tunnel: [w424] -> w396 mode=indexing
                    n282 = Format Into String(format string="%#f" ("格式字符串"), w426) -> (resulting string=w424:string)  [unwired: 2 in, 1 out]
                  }
                  n283 = Number To Decimal String(number=w400) -> (decimal integer string=w407:string)  [unwired: 1 in]
                  n284 = Number To Decimal String(number=w379) -> (decimal integer string=w378:string)  [unwired: 1 in]
                  n285 = Array Subset(array=w393, index=0 ("索引"), length=51 ("长度")) -> (w390:string[])
                  n286 = Insert Into Array(array=w398, new element #1=w390, new element #2=w397, new element #3=w396, new element #4=w395, new element #5=w378) -> (w394:string[])  [unwired: 1 in]
                  n287 = Insert Into Array(array=w394, index=0 ("索引"), new element=w407) -> (w405:string[])
                }
                frame #1 {
                  w442 = ".ini" ("pattern (all files)")
                  n288 = call <vilib>:"Application Directory.vi"() -> ("Application Directory"=w445:path)
                  n289 = local read "工程代号"() -> (w443:string)
                  n290 = call "路径分析-8.6.vi"("第二个文件夹"="", "第一个文件夹"="ConfigFile", "输入路径"=w445) -> ("输出路径"=w441:path)  [unwired: 8 in]
                  n291 = Concatenate Strings(w443, "test" ("字符串"), w442) -> (w439:string)
                  n292 = Build Path(base path=w441, name or relative path=w439) -> (appended path=w440:path)
                  n293 = case shown="1" w448 {
                    tunnel: "选择要保存的位置" ("prompt") -> [_ w473]
                    tunnel: [w462 w464] -> w451
                    tunnel: [_ w471] -> w450
                    tunnel: w440 -> [w462 _]
                    tunnel: w442 -> [_ w470]
                    frame 0, Default {
                    }
                    frame 1 {
                      n294 = local read "工程代号"() -> (w468:string)
                      n295 = Concatenate Strings(w468, "V0" ("字符串"), ".ini" ("pattern (all files)")) -> (w466:string)
                      n296 = call "文件对话框"("prompt"=w473, "default name"=w466, "pattern (all files)"=w470) -> ("selected path"=w464:path, "exists"=w465:bool, "cancelled"=w471:bool, "error out"=w472:errorcluster)  [unwired: 9 in]
                      n297 = call <vilib>:"Clear Errors.vi"("error in (no error)"=w472) -> ("error out"=w463:errorcluster)  [unwired: 6 in]
                      n298 = case shown="真" w465 {
                        tunnel: w464 -> [_ w476]
                        tunnel: w463 -> [_ w475]
                        tunnel: [_ w474] -> _
                        frame False {
                        }
                        frame True {
                          n299 = Delete(path (use dialog)=w476, error in=w475) -> (error out=w474:errorcluster)  [unwired: 3 in, 2 out]
                        }
                      }
                    }
                  }
                  n300 = Insert Into Array(array=w455, index=0 ("索引"), new element="从板个数" ("新元素/子数组")) -> (w454:string[])
                  n301 = Insert Into Array(array=w454, new element #1=string[] ["总电压过高一级", "总电压过低一级", "温度过高一级", "温度过低一级", "整组电压不均衡一级", "单组电压不均衡一级", "整组温度不均衡一级", "单组温度不均衡一级", "单体电压过高一级", "单体电压过低一级", "充电电流过高一级", "放电电流过高一级", "SOC过高一级", "SOC过低一级", "内阻过大一级", "极柱温度过高一级", "SOH过低一级", "总电压过高二级", "总电压过低二级", "温度过高二级", "温度过低二级", "整组电压不均衡二级", "单组电压不均衡二级", "整组温度不均衡二级", "单组温度不均衡二级", "单体电压过高二级", "单体电压过低二级", "充电电流过高二级", "放电电流过高二级", "SOC过高二级", "SOC过低二级", "内阻过大二级", "极柱温度过高二级", "SOH过低二级", "总电压过高三级", "总电压过低三级", "温度过高三级", "温度过低三级", "整组电压不均衡三级", "单组电压不均衡三级", "整组温度不均衡三级", "单组温度不均衡三级", "单体电压过高三级", "单体电压过低三级", "充电电流过高三级", "放电电流过高三级", "SOC过高三级", "SOC过低三级", "内阻过大三级", "极柱温度过高三级", "SOH过低三级", "风机开启温度", "风机关闭温度", "加热开启温度", "加热关闭温度", "风机开启温差", "风机关闭温差", "加热关闭温差", "最大允许单体电压", "最小允许单体电压", "最大允许充电电流", "最小允许充电电流", "最大允许总电压", "最大允许充电温度", "最小允许充电温度", "电流步长"], new element #2=w457, new element #3="分流器型号") -> (w458:string[])  [unwired: 1 in]
                  n302 = case shown="假" w450 {
                    tunnel: w461 -> [w481 _]
                    tunnel: w458 -> [w480 _]
                    tunnel: [w479 _] -> w456
                    tunnel: w451 -> [w478 _]
                    tunnel: w449 -> [w477 _]
                    frame False {
                      n303 = call <vilib>:"Open Config Data.vi"("configuration file path"=w478) -> ("refnum"=w479:T11)  [unwired: 8 in, 2 out]
                      n304 = stacked-sequence {
                        tunnel: w481 -> [_ _ _ w499]
                        tunnel: w480 -> [_ _ _ w498]
                        tunnel: w479 -> [w485 w489 w494 w497]
                        tunnel: w477 -> [_ _ w491 _]
                        frame #0 {
                          n305 = local read "工号"() -> (w482:string)
                          n306 = call-poly <vilib>:"Write Key.vi"("section"="总信息" ("key"), "value"=w482, "key"="工号", "refnum"=w485) -> ()  [unwired: 5 in, 3 out]
                        }
                        frame #1 {
                          n307 = local read "工程代号"() -> (w486:string)
                          n308 = call-poly <vilib>:"Write Key.vi"("section"="总信息" ("key"), "value"=w486, "key"="工程代号", "refnum"=w489) -> ()  [unwired: 5 in, 3 out]
                        }
                        frame #2 {
                          n309 = case shown="1" w491 {
                            tunnel: ["MD5码" ("key") w496] -> w490
                            frame 0, Default {
                            }
                            frame 1 {
                              n310 = local read "MD5 message-digest"() -> (w496:string)
                            }
                          }
                          n311 = call-poly <vilib>:"Write Key.vi"("section"="总信息" ("key"), "value"=w490, "key"="MD5码", "refnum"=w494) -> ()  [unwired: 5 in, 3 out]
                        }
                        frame #3 {
                          n312 = for {
                            tunnel: w497 -> [w503]
                            tunnel: w499 -> [w502] mode=indexing
                            tunnel: w498 -> [w500] mode=indexing
                            n313 = call-poly <vilib>:"Write Key.vi"("section"="主板" ("key"), "value"=w502, "key"=w500, "refnum"=w503) -> ()  [unwired: 5 in, 3 out]
                          }
                        }
                      }
                    }
                    frame True {
                    }
                  }
                }
                frame #2 {
                  n314 = case shown="假" w506 {
                    tunnel: w509 -> [w511 _]
                    tunnel: w508 -> [w516 _]
                    tunnel: w507 -> [w515 _]
                    tunnel: w505 -> [w513 _]
                    tunnel: w504 -> [w510 _]
                    frame False {
                      n315 = local read "输出数组"() -> (w517:string[][])
                      n316 = Transpose 2D Array(2D array=w517) -> (transposed array=w514:string[][])
                      n317 = for {
                        N: w516 -> [_]
                        tunnel: w514 -> [w541] mode=indexing
                        tunnel: w511 -> [w540]
                        tunnel: [w534] -> _
                        tunnel: [w533] -> w512
                        tunnel: w510 -> [w532]
                        i -> [w539]
                        n318 = Increment(x=w539) -> (x+1=w538:i32)
                        n319 = Number To Decimal String(number=w538) -> (decimal integer string=w537:string)  [unwired: 1 in]
                        n320 = Concatenate Strings("从板", w537) -> (w535:string)
                        n321 = for {
                          tunnel: w541 -> [w543] mode=indexing
                          tunnel: w540 -> [w547]
                          tunnel: w535 -> [w546]
                          tunnel: [w545] -> w534
                          tunnel: [w544] -> w533
                          tunnel: w532 -> [w542] mode=indexing
                          n322 = call-poly <vilib>:"Write Key.vi"("section"=w546, "value"=w543, "key"=w542, "refnum"=w547) -> ("error out"=w544:errorcluster, "refnum out"=w545:T11)  [unwired: 5 in, 1 out]
                        }
                      }
                      n323 = stacked-sequence {
                        tunnel: w512 -> [_ _ _]
                        tunnel: w515 -> [_ w521 w523]
                        tunnel: w513 -> [_ _ w522]
                        tunnel: w511 -> [w518 _ _]
                        frame #0 {
                          n324 = call <vilib>:"Close Config Data.vi"("refnum"=w518) -> ("error out"=w519:errorcluster)  [unwired: 9 in, 1 out]
                          n325 = call <vilib>:"Clear Errors.vi"("error in (no error)"=w519) -> ()  [unwired: 6 in, 1 out]
                        }
                        frame #1 {
                          n326 = call <vilib>:"MD5Checksum File.vi"("Path"=w521) -> ("MD5 message-digest"=→"MD5 message-digest":string)  [unwired: 9 in, 1 out]
                        }
                        frame #2 {
                          n327 = case shown="1" w522 {
                            tunnel: w523 -> [w524 w528]
                            frame 0, Default {
                              n328 = Delete(path (use dialog)=w524) -> (error out=w525:errorcluster)  [unwired: 4 in, 2 out]
                              n329 = call <vilib>:"Clear Errors.vi"("error in (no error)"=w525) -> ()  [unwired: 6 in, 1 out]
                            }
                            frame 1 {
                              n330 = Path To String(path=w528) -> (string=w527:string)
                              n331 = Concatenate Strings("保存完成，路径为：" ("按钮名称（“确定”）"), "\n", w527) -> (w526:string)
                              n332 = One Button Dialog(message=w526, button name ("OK")="确定" ("按钮名称（“确定”）")) -> ()  [unwired: 1 out]
                            }
                          }
                        }
                      }
                    }
                    frame True {
                    }
                  }
                }
              }
            }
            n333 = local write "MD5 message-digest"("" ("MD5 message-digest")) -> ()
          }
        }
      }
      event "预览": Value Change {
        n334 = event-data() -> ("NewVal"=w549:bool)  [unwired: 1 in, 5 out]
        n335 = case shown="真" w549 {
          tunnel: w548 -> [_ w550]
          frame False {
          }
          frame True {
            n336 = stacked-sequence {
              seq-local: [w578 _ _ _] -> [_ w626 _ _]
              seq-local: [w576 _ _ _] -> [_ w619 _ _]
              seq-local: [w574 _ _ _] -> [_ w620 _ _]
              seq-local: [w573 _ _ _] -> [_ _ w656 _]
              seq-local: [_ w613 _ _] -> [_ _ w652 _]
              tunnel: w550 -> [_ _ w649 _]
              frame #0 {
                n337 = local read "一级故障"() -> (w590:dbl[][])
                n338 = local read "充电控制参数"() -> (w554:T4)
                n339 = local read "主板信息"() -> (w591:string[][])
                n340 = local read "电池信息"() -> (w581:string[][])
                n341 = local read "加热控制参数"() -> (w587:T3)
                n342 = Array Subset(array=w591, index (row)=0 ("索引"), index (col)=0 ("索引"), length (col)=2 ("索引")) -> (w593:string[][])  [unwired: 1 in]
                n343 = Transpose 2D Array(2D array=w590) -> (transposed array=w572:dbl[][])
                n344 = for {
                  tunnel: w572 -> [w607] mode=indexing
                  shift-right: [w606] -> w566
                  shift-left: string[] [] -> [w604]
                  n345 = for {
                    N: 17 -> [_]
                    tunnel: w607 -> [w610] mode=indexing
                    tunnel: [w608] -> w605 mode=indexing
                    n346 = Format Into String(format string="%#f" ("格式字符串"), w610) -> (resulting string=w608:string)  [unwired: 2 in, 1 out]
                  }
                  n347 = Insert Into Array(array=w604, new element=w605) -> (w606:string[])  [unwired: 1 in]
                }
                n348 = Unbundle(w554) -> ("最大允许单体电压(V)"=w562:dbl, "最大允许总电压(V)"=w558:dbl, "最小允许单体电压(V)"=w561:dbl, "最大允许充电电流(A)"=w560:dbl, "最小允许充电电流(A)"=w559:dbl, "最大允许充电温度(℃)"=w557:dbl, "最小允许充电温度(℃)"=w556:dbl, "电流步长"=w555:dbl)
                n349 = Index Array(array=w593, index (col) #1=1 ("禁用的索引 (列)"), index (col) #2=0 ("索引 (列)")) -> (element #1=w571:string[], element #2=w576:string[])  [unwired: 2 in]
                n350 = local read "从板个数"() -> (w573:dbl)
                n351 = Array Subset(array=w581, index (row)=0 ("索引"), index (col)=0 ("索引"), length (col)=2 ("索引")) -> (w585:string[][])  [unwired: 1 in]
                n352 = Cluster To Array(cluster=w587) -> (array=w588:dbl[])
                n353 = local read "分流器型号"() -> (w552:T2)
                n354 = for {
                  tunnel: w588 -> [w602] mode=indexing
                  tunnel: [w600] -> w570 mode=indexing
                  n355 = Format Into String(format string="%#f" ("格式字符串"), w602) -> (resulting string=w600:string)  [unwired: 2 in, 1 out]
                }
                n356 = Build Array(w562, w561, w560, w559, w558, w557, w556, w555) -> (w553:dbl[])
                n357 = Index Array(array=w585, index (col) #1=0 ("禁用的索引 (列)"), index (col) #2=1 ("禁用的索引 (列)")) -> (element #1=w574:string[], element #2=w568:string[])  [unwired: 2 in]
                n358 = for {
                  tunnel: w553 -> [w599] mode=indexing
                  tunnel: [w597] -> w569 mode=indexing
                  n359 = Format Into String(format string="%#f" ("格式字符串"), w599) -> (resulting string=w597:string)  [unwired: 2 in, 1 out]
                }
                n360 = Number To Decimal String(number=w573) -> (decimal integer string=w580:string)  [unwired: 1 in]
                n361 = Number To Decimal String(number=w552) -> (decimal integer string=w551:string)  [unwired: 1 in]
                n362 = Array Subset(array=w566, index=0 ("索引"), length=51 ("长度")) -> (w563:string[])
                n363 = Insert Into Array(array=w571, new element #1=w563, new element #2=w570, new element #3=w569, new element #4=w568, new element #5=w551) -> (w567:string[])  [unwired: 1 in]
                n364 = Insert Into Array(array=w567, index=0 ("索引"), new element=w580) -> (w578:string[])
              }
              frame #1 {
                n365 = call <vilib>:"Application Directory.vi"() -> ("Application Directory"=w627:path)
                n366 = local read "工程代号"() -> (w624:string)
                n367 = call "路径分析-8.6.vi"("第二个文件夹"="", "第一个文件夹"="ConfigFile", "输入路径"=w627) -> ("输出路径"=w614:path)  [unwired: 8 in]
                n368 = Concatenate Strings(w624, "-rc" ("字符串"), ".ini" ("pattern (all files)")) -> (w615:string)
                n369 = Build Path(base path=w614, name or relative path=w615) -> (appended path=w613:path)
                n370 = call <vilib>:"Open Config Data.vi"("configuration file path"=w613) -> ("refnum"=w612:T11)  [unwired: 8 in, 2 out]
                n371 = Insert Into Array(array=w619, index=0 ("索引"), new element="从板个数" ("新元素/子数组")) -> (w618:string[])
                n372 = Insert Into Array(array=w618, new element #1=string[] ["总电压过高一级", "总电压过低一级", "温度过高一级", "温度过低一级", "整组电压不均衡一级", "单组电压不均衡一级", "整组温度不均衡一级", "单组温度不均衡一级", "单体电压过高一级", "单体电压过低一级", "充电电流过高一级", "放电电流过高一级", "SOC过高一级", "SOC过低一级", "内阻过大一级", "极柱温度过高一级", "SOH过低一级", "总电压过高二级", "总电压过低二级", "温度过高二级", "温度过低二级", "整组电压不均衡二级", "单组电压不均衡二级", "整组温度不均衡二级", "单组温度不均衡二级", "单体电压过高二级", "单体电压过低二级", "充电电流过高二级", "放电电流过高二级", "SOC过高二级", "SOC过低二级", "内阻过大二级", "极柱温度过高二级", "SOH过低二级", "总电压过高三级", "总电压过低三级", "温度过高三级", "温度过低三级", "整组电压不均衡三级", "单组电压不均衡三级", "整组温度不均衡三级", "单组温度不均衡三级", "单体电压过高三级", "单体电压过低三级", "充电电流过高三级", "放电电流过高三级", "SOC过高三级", "SOC过低三级", "内阻过大三级", "极柱温度过高三级", "SOH过低三级", "风机开启温度", "风机关闭温度", "加热开启温度", "加热关闭温度", "风机开启温差", "风机关闭温差", "加热关闭温差", "最大允许单体电压", "最小允许单体电压", "最大允许充电电流", "最小允许充电电流", "最大允许总电压", "最大允许充电温度", "最小允许充电温度", "电流步长"], new element #2=w620, new element #3="分流器型号") -> (w621:string[])  [unwired: 1 in]
                n373 = stacked-sequence {
                  tunnel: w626 -> [_ _ w642]
                  tunnel: w621 -> [_ _ w641]
                  tunnel: w612 -> [w630 w634 w640]
                  frame #0 {
                    n374 = local read "工号"() -> (w631:string)
                    n375 = call-poly <vilib>:"Write Key.vi"("section"="总信息" ("key"), "value"=w631, "key"="工号", "refnum"=w630) -> ()  [unwired: 5 in, 3 out]
                  }
                  frame #1 {
                    n376 = local read "工程代号"() -> (w635:string)
                    n377 = call-poly <vilib>:"Write Key.vi"("section"="总信息" ("key"), "value"=w635, "key"="工程代号", "refnum"=w634) -> ()  [unwired: 5 in, 3 out]
                  }
                  frame #2 {
                    n378 = for {
                      tunnel: w640 -> [w648]
                      tunnel: w642 -> [w647] mode=indexing
                      tunnel: w641 -> [w645] mode=indexing
                      tunnel: [w644] -> w639
                      tunnel: [w643] -> w638
                      n379 = call-poly <vilib>:"Write Key.vi"("section"="主板" ("key"), "value"=w647, "key"=w645, "refnum"=w648) -> ("error out"=w643:errorcluster, "refnum out"=w644:T11)  [unwired: 5 in, 1 out]
                    }
                    n380 = call <vilib>:"Close Config Data.vi"("error in (no error)"=w638, "refnum"=w639) -> ()  [unwired: 8 in, 2 out]
                  }
                }
              }
              frame #2 {
                n381 = local read "输出数组"() -> (w655:string[][])
                n382 = Transpose 2D Array(2D array=w655) -> (transposed array=w654:string[][])
                n383 = call <vilib>:"Open Config Data.vi"("configuration file path"=w652) -> ("refnum"=w651:T11)  [unwired: 8 in, 2 out]
                n384 = for {
                  N: w656 -> [_]
                  tunnel: w654 -> [w666] mode=indexing
                  tunnel: w651 -> [w665]
                  tunnel: [w659] -> w650
                  tunnel: [w658] -> w653
                  tunnel: w649 -> [w657]
                  i -> [w664]
                  n385 = Increment(x=w664) -> (x+1=w663:i32)
                  n386 = Number To Decimal String(number=w663) -> (decimal integer string=w662:string)  [unwired: 1 in]
                  n387 = Concatenate Strings("从板", w662) -> (w660:string)
                  n388 = for {
                    tunnel: w666 -> [w668] mode=indexing
                    tunnel: w665 -> [w672]
                    tunnel: w660 -> [w671]
                    tunnel: [w670] -> w659
                    tunnel: [w669] -> w658
                    tunnel: w657 -> [w667] mode=indexing
                    n389 = call-poly <vilib>:"Write Key.vi"("section"=w671, "value"=w668, "key"=w667, "refnum"=w672) -> ("error out"=w669:errorcluster, "refnum out"=w670:T11)  [unwired: 5 in, 1 out]
                  }
                }
                n390 = stacked-sequence {
                  tunnel: w652 -> [_ w676 _]
                  tunnel: w653 -> [_ _ _]
                  tunnel: w650 -> [w673 _ _]
                  frame #0 {
                    n391 = call <vilib>:"Close Config Data.vi"("refnum"=w673) -> ("error out"=w674:errorcluster)  [unwired: 9 in, 1 out]
                    n392 = call <vilib>:"Clear Errors.vi"("error in (no error)"=w674) -> ()  [unwired: 6 in, 1 out]
                  }
                  frame #1 {
                    n393 = Open/Create/Replace File(file path (use dialog)=w676) -> (refnum out=w683:refnum<file>, error out=w682:errorcluster)  [unwired: 5 in, 1 out]
                    n394 = Read from Text File(file (use dialog)=w683, error in=w682) -> (refnum out=w680:refnum<file>, text=w681:string, error out=w679:errorcluster)  [unwired: 2 in, 1 out]
                    n395 = call "预览结果显示.vi"("预览结果"=w681) -> ()  [unwired: 1 out]
                    n396 = Close File(refnum=w680, error in=w679) -> (error out=w677:errorcluster)  [unwired: 1 out]
                    n397 = local write "预览"(FALSE ("预览")) -> ()
                    n398 = Delete(path (use dialog)=w676, error in=w677) -> (error out=w675:errorcluster)  [unwired: 3 in, 2 out]
                    n399 = call <vilib>:"Clear Errors.vi"("error in (no error)"=w675) -> ()  [unwired: 6 in, 1 out]
                  }
                  frame #2 {
                    n400 = disable-structure shown="禁用" {
                      disable-tunnel: _ -> [w686 _]
                      frame Disabled {
                        n401 = Path To String(path=w686) -> (string=w685:string)
                        n402 = Concatenate Strings("保存完成，路径为：" ("按钮名称（“确定”）"), "\n", w685) -> (w684:string)
                        n403 = One Button Dialog(message=w684, button name ("OK")="确定" ("按钮名称（“确定”）")) -> ()  [unwired: 1 out]
                      }
                      frame Enabled {
                      }
                    }
                  }
                }
              }
              frame #3 {
              }
            }
          }
        }
      }
      event "读取(ini)": Value Change {
        n404 = event-data() -> ("NewVal"=w690:bool)  [unwired: 1 in, 5 out]
        n405 = case shown="真" w690 {
          frame False {
          }
          frame True {
            n406 = stacked-sequence {
              seq-local: [w702 _ _ _ _] -> [_ w760 w834 _ _]
              seq-local: [w692 _ _ _ _] -> [_ w759 w832 w923 w965]
              seq-local: [_ w758 _ _ _] -> [_ _ _ _ w964]
              frame #0 {
                n407 = call "文件对话框"("prompt"="选择要读取的文件") -> ("selected path"=w696:path, "cancelled"=w695:bool, "error out"=w701:errorcluster)  [unwired: 11 in, 1 out]
                n408 = Strip Path(path=w696) -> (stripped path=w691:path, name=w700:string)
                n409 = global write "配置文件全局.vi" "参数生成器读取地址"(w691) -> ()
                n410 = Match Pattern(string=w700, regular expression=".ini" ("正则表达式")) -> (offset past match=w698:i32)  [unwired: 1 in, 3 out]
                n411 = Equal?(x=w698, y=-1) -> (x = y?=w694:bool)
                n412 = case shown="假" w694 {
                  tunnel: w696 -> [w716 _]
                  tunnel: [w704 _] -> w693
                  frame False {
                    w727 = "MD5码" ("key")
                    w728 = "总信息" ("section")
                    n413 = Strip Path(path=w716) -> (stripped path=w714:path, name=w713:string)
                    n414 = Match Pattern(string=w713, regular expression=".ini" ("正则表达式")) -> (before substring=w710:string, match substring=w711:string)  [unwired: 1 in, 2 out]
                    n415 = Concatenate Strings(w710, "-rc" ("字符串"), w711) -> (w709:string)
                    n416 = Build Path(base path=w714, name or relative path=w709) -> (appended path=w715:path)
                    n417 = Copy(10:w715, 11:w716) -> (3:w720:path)  [unwired: 3 in, 2 out]
                    n418 = call <vilib>:"Open Config Data.vi"("create file if necessary (T)"=FALSE, "configuration file path"=w720) -> ("refnum"=w730:T11)  [unwired: 7 in, 2 out]
                    n419 = call-poly <vilib>:"Read Key.vi"("section"=w728, "key"=w727, "refnum"=w730) -> ("value"=w707:string, "refnum out"=w729:T11)  [unwired: 5 in, 2 out]
                    n420 = call-poly <vilib>:"Write Key.vi"("section"=w728, "value"=w727, "key"=w727, "refnum"=w729) -> ("error out"=w724:errorcluster, "found?"=w723:bool, "refnum out"=w722:T11)  [unwired: 5 in]
                    n421 = call <vilib>:"Close Config Data.vi"("error in (no error)"=w724, "write file if changed (T)"=w723, "refnum"=w722) -> ("error out"=w721:errorcluster, "file path"=w718:path)  [unwired: 7 in]
                    n422 = call <vilib>:"MD5Checksum File.vi"("error in (no error)"=w721, "Path"=w718) -> ("error out"=w719:errorcluster, "MD5 message-digest"=w726:string)  [unwired: 8 in]
                    n423 = for {
                      N: 2 -> [_]
                      tunnel: w726 -> [w735]
                      tunnel: [w734] -> w725 mode=indexing
                      tunnel: w707 -> [w733]
                      i -> [w732]
                      n424 = case shown="1" w732 {
                        tunnel: w735 -> [w739 w740]
                        tunnel: [w738 w742] -> w734
                        tunnel: w733 -> [w737 w741]
                        frame 0, Default {
                          n425 = To Upper Case(1:w739) -> (0:w736:string)
                          n426 = Equal?(x=w736, y=w737) -> (x = y?=w738:bool)
                        }
                        frame 1 {
                          n427 = Equal?(x=w740, y=w741) -> (x = y?=w742:bool)
                        }
                      }
                    }
                    n428 = Or Array Elements(Boolean array=w725) -> (logical OR=w705:bool)
                    n429 = Not(x=w705) -> (.not. x?=w704:bool)
                    n430 = Delete(path (use dialog)=w718, error in=w719) -> (error out=w717:errorcluster)  [unwired: 3 in, 2 out]
                    n431 = call <vilib>:"Clear Errors.vi"("error in (no error)"=w717) -> ()  [unwired: 6 in, 1 out]
                  }
                  frame True {
                  }
                }
                n432 = call <vilib>:"Clear Errors.vi"("error in (no error)"=w701) -> ()  [unwired: 6 in, 1 out]
                n433 = Compound Arithmetic op=OR(w695, w694, w693) -> (w692:bool)
                n434 = case shown="假" w692 {
                  tunnel: w696 -> [w747 _]
                  tunnel: [w746 _] -> w702
                  frame False {
                    w749 = "总信息" ("section")
                    n435 = call <vilib>:"Open Config Data.vi"("create file if necessary (T)"=FALSE, "configuration file path"=w747) -> ("refnum"=w746:T11)  [unwired: 7 in, 2 out]
                    n436 = call <vilib>:"Get Key Names.vi"("section"=w749, "refnum"=w746) -> ("key names"=w748:string[], "refnum out"=w750:T11)  [unwired: 6 in, 2 out]
                    n437 = for {
                      tunnel: w750 -> [w755]
                      tunnel: w749 -> [w754]
                      tunnel: w748 -> [w753] mode=indexing
                      tunnel: [w752] -> w745 mode=indexing
                      n438 = call-poly <vilib>:"Read Key.vi"("section"=w754, "key"=w753, "refnum"=w755) -> ("value"=w752:string)  [unwired: 5 in, 3 out]
                    }
                    n439 = Index Array(array=w745) -> (element #1=w744:string, element #2=w743:string)  [unwired: 2 in]
                    n440 = local write "工程代号"(w743) -> ()
                    n441 = local write "工号"(w744) -> ()
                  }
                  frame True {
                    n442 = One Button Dialog(message="文件格式错误或文件不正确" ("消息"), button name ("OK")="确定" ("按钮名称（“确定”）")) -> ()  [unwired: 1 out]
                  }
                }
              }
              frame #1 {
                n443 = case shown="假" w759 {
                  tunnel: w760 -> [w785 _]
                  tunnel: [w779 _] -> w758
                  frame False {
                    w789 = 15 ("长度")
                    w821 = "主板" ("section")
                    n444 = call <vilib>:"Get Key Names.vi"("section"=w821, "refnum"=w785) -> ("key names"=w765:string[], "refnum out"=w822:T11)  [unwired: 6 in, 2 out]
                    n445 = for {
                      tunnel: w822 -> [w830]
                      tunnel: w821 -> [w829]
                      tunnel: w765 -> [w828] mode=indexing
                      tunnel: [w827] -> w764 mode=indexing
                      n446 = call-poly <vilib>:"Read Key.vi"("section"=w829, "key"=w828, "refnum"=w830) -> ("value"=w827:string)  [unwired: 5 in, 3 out]
                    }
                    n447 = Search 1D Array(1D array=w765, element="总电压过高一级" ("元素"), start index (0)=0 ("开始索引(0)")) -> (index of element=w798:i32)
                    n448 = Search 1D Array(1D array=w765, element="风机开启温度" ("元素"), start index (0)=w798) -> (index of element=w799:i32)
                    n449 = Search 1D Array(1D array=w765, element="电池串联" ("元素"), start index (0)=w798) -> (index of element=w790:i32)
                    n450 = Search 1D Array(1D array=w765, element="分流器型号" ("元素")) -> (index of element=w763:i32)  [unwired: 1 in]
                    n451 = Decrement(x=w798) -> (x-1=w784:i32)
                    n452 = Index Array(array=w764, index=w763) -> (element=w762:string)
                    n453 = Array Subset(array=w764, index=w799, length=15 ("长度")) -> (w794:string[])
                    n454 = Array Subset(array=w764, index=w798, length=51 ("长度")) -> (w812:string[])
                    n455 = Array Subset(array=w764, index=w790, length=w789) -> (w787:string[])
                    n456 = Array Subset(array=w765, index=1 ("索引"), length=w784) -> (w816:string[])
                    n457 = Array Subset(array=w765, index=w790, length=w789) -> (w788:string[])
                    n458 = Array Subset(array=w764, index=1 ("索引"), length=w784) -> (w815:string[])
                    n459 = Index Array(array=w764, index=0 ("索引")) -> (element=w782:string)
                    n460 = for {
                      tunnel: w812 -> [w826] mode=indexing
                      tunnel: [w825] -> w811 mode=indexing
                      n461 = Fract/Exp String To Number(string=w826) -> (number=w825:dbl)  [unwired: 3 in, 1 out]
                    }
                    n462 = for {
                      tunnel: w794 -> [w824] mode=indexing
                      tunnel: [w823] -> w793 mode=indexing
                      n463 = Fract/Exp String To Number(string=w824) -> (number=w823:dbl)  [unwired: 3 in, 1 out]
                    }
                    n464 = Decimal String To Number(string=w762) -> (number=w761:i32)  [unwired: 2 in, 1 out]
                    n465 = Build Array(w816, w815) -> (w814:string[][])
                    n466 = Decimal String To Number(string=w782) -> (number=w779:i32)  [unwired: 2 in, 1 out]
                    n467 = Build Array(w788, w787) -> (w786:string[][])
                    n468 = local write "分流器型号"(w761) -> ()
                    n469 = Transpose 2D Array(2D array=w814) -> (transposed array=w781:string[][])
                    n470 = Transpose 2D Array(2D array=w786) -> (transposed array=w780:string[][])
                    n471 = Delete From Array(array=w811, length=17 ("长度"), index=0 ("索引")) -> (deleted portion=w808:dbl[], array with subset deleted=w807:dbl[])
                    n472 = Delete From Array(array=w793, length=7 ("长度"), index=0 ("索引")) -> (deleted portion=w792:dbl[], array with subset deleted=w777:dbl[])
                    n473 = Delete From Array(array=w807, length=17 ("长度"), index=0 ("索引")) -> (deleted portion=w778:dbl[], array with subset deleted=w804:dbl[])
                    n474 = local write "主板信息"(w781) -> ()
                    n475 = local write "电池信息"(w780) -> ()
                    n476 = local write "从板个数"(w779) -> ()
                    n477 = Array To Cluster(array=w792) -> (cluster=w791:T10)
                    n478 = Build Array(w808, w778, w804) -> (w803:dbl[][])
                    n479 = Index Array(array=w777) -> (element #1=w774:dbl, element #2=w772:dbl, element #3=w771:dbl, element #4=w770:dbl, element #5=w773:dbl, element #6=w769:dbl, element #7=w768:dbl, element #8=w767:dbl)  [unwired: 8 in]
                    n480 = local write "加热控制参数"(w791) -> ()
                    n481 = Transpose 2D Array(2D array=w803) -> (transposed array=w802:dbl[][])
                    n482 = Build Array(w774, w773, w772, w771, w770, w769, w768, w767) -> (w775:dbl[])
                    n483 = local write "一级故障"(w802) -> ()
                    n484 = Array To Cluster(array=w775) -> (cluster=w776:T12)
                    n485 = local write "充电控制参数"(w776) -> ()
                  }
                  frame True {
                  }
                }
              }
              frame #2 {
                n486 = case shown="真" w832 {
                  tunnel: w834 -> [w901 _]
                  frame False {
                    w836 = string[] ["从板板号", "电压个数", "温度个数", "第一个保险通道", "第一个保险位置", "第二个保险通道", "第二个保险位置", "第三个保险通道", "第三个保险位置", "第四个保险通道", "第四个保险位置", "第五个保险通道", "第五个保险位置", "第六个保险通道", "第六个保险位置", "第七个保险通道", "第七个保险位置", "第八个保险通道", "第八个保险位置", "第九个保险通道", "第九个保险位置", "第十个保险通道", "第十个保险位置", "第1通道电压个数", "第2通道电压个数", "第3通道电压个数", "第4通道电压个数", "第5通道电压个数", "风机开启温度", "风机关闭温度", "加热开启温度", "加热关闭温度", "风机开启温差", "风机关闭温差", "加热关闭温差", "电压过高一级", "电压过低一级", "温度过高一级", "温度过低一级", "电压不均衡一级", "温度不均衡一级", "SOC过低一级", "电压过高二级", "电压过低二级", "温度过高二级", "温度过低二级", "电压不均衡二级", "温度不均衡二级", "SOC过低二级", "电压过高三级", "电压过低三级", "温度过高三级", "温度过低三级", "电压不均衡三级", "温度不均衡三级", "SOC过低三级", "均衡计算-电压高阀值1级", "均衡计算-电压高阀值2级", "均衡计算-电压低阀值1级", "均衡计算-电压低阀值2级", "均衡计算-最低电压阀值", "均衡停止-最低电压阀值", "均衡计算-电压极差阀值", "充电结束电压(90%)", "充电结束电压(91%)", "充电结束电压(92%)", "充电结束电压(93%)", "充电结束电压(94%)", "充电结束电压(95%)", "充电结束电压(96%)", "充电结束电压(97%)", "充电结束电压(98%)", "充电结束电压(99%)", "充电结束电压(100%)"] ("从板表头")
                    (unwired) string[] ["从板板号", "电压个数", "电压起始值", "温度个数", "温度起始值", "第一个保险通道", "第一个保险位置", "第二个保险通道", "第二个保险位置", "第三个保险通道", "第三个保险位置", "第四个保险通道", "第四个保险位置", "第五个保险通道", "第五个保险位置", "第六个保险通道", "第六个保险位置", "第七个保险通道", "第七个保险位置", "第八个保险通道", "第八个保险位置", "第九个保险通道", "第九个保险位置", "第十个保险通道", "第十个保险位置", "第1通道电压个数", "第2通道电压个数", "第3通道电压个数", "第4通道电压个数", "第5通道电压个数", "第6通道电压个数", "第7通道电压个数", "第8通道电压个数", "第9通道电压个数", "第10通道电压个数", "第11通道电压个数", "第12通道电压个数", "第13通道电压个数", "第14通道电压个数", "第15通道电压个数", "第16通道电压个数", "第17通道电压个数", "第18通道电压个数", "第19通道电压个数", "第20通道电压个数", "风机开启温度", "风机关闭温度", "加热开启温度", "加热关闭温度", "风机开启温差", "风机关闭温差", "加热关闭温差", "电压过高一级", "电压过低一级", "温度过高一级", "温度过低一级", "电压不均衡一级", "温度不均衡一级", "SOC过低一级", "电压过高二级", "电压过低二级", "温度过高二级", "温度过低二级", "电压不均衡二级", "温度不均衡二级", "SOC过低二级", "电压过高三级", "电压过低三级", "温度过高三级", "温度过低三级", "电压不均衡三级", "温度不均衡三级", "SOC过低三级", "均衡计算-电压高阀值1级", "均衡计算-电压高阀值2级", "均衡计算-电压低阀值1级", "均衡计算-电压低阀值2级", "均衡计算-最低电压阀值", "均衡停止-最低电压阀值", "均衡计算-电压极差阀值", "充电结束电压(90%)", "充电结束电压(91%)", "充电结束电压(92%)", "充电结束电压(93%)", "充电结束电压(94%)", "充电结束电压(95%)", "充电结束电压(96%)", "充电结束电压(97%)", "充电结束电压(98%)", "充电结束电压(99%)", "充电结束电压(100%)"] ("从板表头")
                    w893 = 1 ("索引")
                    n487 = call <vilib>:"Get Section Names.vi"("refnum"=w901) -> ("section names"=w900:string[], "refnum out"=w896:T11)  [unwired: 8 in, 1 out]
                    n488 = local read "从板板号"() -> (w870:dbl)
                    n489 = Delete From Array(array=w900, length=2 ("长度"), index=0 ("索引")) -> (array with subset deleted=w897:string[])  [unwired: 1 out]
                    n490 = Decrement(x=w870) -> (x-1=w868:dbl)
                    n491 = for {
                      tunnel: w897 -> [w917] mode=indexing
                      tunnel: w896 -> [w918]
                      tunnel: [w910] -> w895 mode=indexing
                      tunnel: [w909] -> w863
                      n492 = call <vilib>:"Get Key Names.vi"("section"=w917, "refnum"=w918) -> ("key names"=w909:string[], "refnum out"=w916:T11)  [unwired: 6 in, 2 out]
                      n493 = for {
                        tunnel: w909 -> [w922] mode=indexing
                        tunnel: w917 -> [w921]
                        tunnel: w916 -> [w920]
                        tunnel: [w919] -> w910 mode=indexing
                        n494 = call-poly <vilib>:"Read Key.vi"("section"=w921, "key"=w922, "refnum"=w920) -> ("value"=w919:string)  [unwired: 5 in, 3 out]
                      }
                      n495 = Index Array(array=w910, index=0 ("索引")) -> (element=w913:string)
                      n496 = local read "输出数组"() -> (w914:string[][])
                      n497 = Decimal String To Number(string=w913) -> (number=w912:i32)  [unwired: 2 in, 1 out]
                      n498 = Decrement(x=w912) -> (x-1=w908:i32)
                      n499 = Replace Array Subset(array=w914, new element=w910, index (col)=w908) -> (w911:string[][])  [unwired: 1 in]
                      n500 = local write "输出数组"(w911) -> ()
                    }
                    n501 = Index Array(array=w895, index (row)=w868) -> (element=w862:string[])  [unwired: 1 in]
                    n502 = Search 1D Array(1D array=w863, element="风机开启温度" ("元素")) -> (index of element=w888:i32)  [unwired: 1 in]
                    n503 = Search 1D Array(1D array=w863, element="电压过高一级" ("元素"), start index (0)=w888) -> (index of element=w864:i32)
                    n504 = Search 1D Array(1D array=w863, element="均衡计算-电压高阀值1级" ("元素"), start index (0)=w864) -> (index of element=w866:i32)
                    n505 = Decrement(x=w888) -> (x-1=w890:i32)
                    n506 = Array Subset(array=w862, index=w893, length=27 ("长度")) -> (w892:string[])
                    n507 = Array Subset(array=w862, index=w864, length=21 ("长度")) -> (w874:string[])
                    n508 = Array Subset(array=w863, index=w893, length=w890) -> ()  [unwired: 1 out]
                    n509 = Array Subset(array=w862, index=w888, length=7 ("长度")) -> (w885:string[])
                    n510 = Array Subset(array=w862, index=w866, length=17 ("长度")) -> (w865:string[])
                    n511 = for {
                      tunnel: w874 -> [w905] mode=indexing
                      tunnel: [w904] -> w873 mode=indexing
                      n512 = Fract/Exp String To Number(string=w905) -> (number=w904:dbl)  [unwired: 3 in, 1 out]
                    }
                    n513 = for {
                      tunnel: w885 -> [w907] mode=indexing
                      tunnel: [w906] -> w884 mode=indexing
                      n514 = Fract/Exp String To Number(string=w907) -> (number=w906:dbl)  [unwired: 3 in, 1 out]
                    }
                    n515 = for {
                      tunnel: w865 -> [w903] mode=indexing
                      tunnel: [w902] -> w842 mode=indexing
                      n516 = Fract/Exp String To Number(string=w903) -> (number=w902:dbl)  [unwired: 3 in, 1 out]
                    }
                    n517 = Array Subset(array=w836, index=1 ("长度"), length=27 ("长度")) -> (w839:string[])
                    n518 = Build Array(w839, w892) -> (w891:string[][])
                    n519 = local write "从板表头"(w836) -> ()
                    n520 = Delete From Array(array=w873, length=7 ("长度"), index=0 ("索引")) -> (deleted portion=w880:dbl[], array with subset deleted=w879:dbl[])
                    n521 = Array To Cluster(array=w884) -> (cluster=w883:T10)
                    n522 = Transpose 2D Array(2D array=w891) -> (transposed array=w871:string[][])
                    n523 = Delete From Array(array=w879, length=7 ("长度"), index=0 ("索引")) -> (deleted portion=w876:dbl[], array with subset deleted=w875:dbl[])
                    n524 = local write "加热控制参数 2"(w883) -> ()
                    n525 = Build Array(w880, w876, w875) -> (w872:dbl[][])
                    n526 = Transpose 2D Array(2D array=w872) -> (transposed array=w869:dbl[][])
                    n527 = local write "从板信息电压温度通道配置"(w871) -> ()
                    n528 = Index Array(array=w842) -> (element #1=w860:dbl, element #2=w859:dbl, element #3=w858:dbl, element #4=w857:dbl, element #5=w856:dbl, element #6=w855:dbl, element #7=w854:dbl, element #8=w853:dbl, element #9=w852:dbl, element #10=w851:dbl, element #11=w850:dbl, element #12=w849:dbl, element #13=w848:dbl, element #14=w847:dbl, element #15=w846:dbl, element #16=w845:dbl, element #17=w844:dbl, element #18=w843:dbl)  [unwired: 18 in]
                    n529 = local write "一级故障 2"(w869) -> ()
                    n530 = local read "均衡参数"() -> (w840:T1)
                    n531 = Bundle(cluster=w840, "充电结束电压(90%)"=w853, "充电结束电压(91%)"=w852, "充电结束电压(92%)"=w851, "充电结束电压(93%)"=w850, "充电结束电压(94%)"=w849, "均衡计算-电压高阀值1级"=w860, "均衡计算-电压高阀值2级"=w859, "均衡计算-电压低阀值1级"=w858, "均衡计算-电压低阀值2级"=w857, "均衡计算-最低电压阀值"=w856, "均衡停止-最低电压阀值"=w855, "均衡计算-电压极差阀值"=w854, "充电结束电压(95%)"=w848, "充电结束电压(96%)"=w847, "充电结束电压(97%)"=w846, "充电结束电压(98%)"=w845, "充电结束电压(99%)"=w844, "充电结束电压(100%)"=w843) -> (w841:T1)
                    n532 = local write "均衡参数"(w841) -> ()
                  }
                  frame True {
                  }
                }
                n533 = local write "读取(ini)"(FALSE ("读取")) -> ()
                n534 = local write "布尔"(TRUE ("布尔")) -> ()
              }
              frame #3 {
                n535 = case shown="假" w923 {
                  frame False {
                    w932 = bool[][] [[FALSE, FALSE, FALSE, FALSE, FALSE, FALSE, FALSE, FALSE, FALSE, FALSE, FALSE, FALSE], [FALSE, FALSE, FALSE, FALSE, FALSE, FALSE, FALSE, FALSE, FALSE, FALSE, FALSE, FALSE], [FALSE, FALSE, FALSE, FALSE, FALSE, FALSE, FALSE, FALSE, FALSE, FALSE, FALSE, FALSE], [FALSE, FALSE, FALSE, FALSE, FALSE, FALSE, FALSE, FALSE, FALSE, FALSE, FALSE, FALSE], [FALSE, FALSE, FALSE, FALSE, FALSE, FALSE, FALSE, FALSE, FALSE, FALSE, FALSE, FALSE], [FALSE, FALSE, FALSE, FALSE, FALSE, FALSE, FALSE, FALSE, FALSE, FALSE, FALSE, FALSE], [FALSE, FALSE, FALSE, FALSE, FALSE, FALSE, FALSE, FALSE, FALSE, FALSE, FALSE, FALSE], [FALSE, FALSE, FALSE, FALSE, FALSE, FALSE, FALSE, FALSE, FALSE, FALSE, FALSE, FALSE], [FALSE, FALSE, FALSE, FALSE, FALSE, FALSE, FALSE, FALSE, FALSE, FALSE, FALSE, FALSE], [FALSE, FALSE, FALSE, FALSE, FALSE, FALSE, FALSE, FALSE, FALSE, FALSE, FALSE, FALSE]]
                    n536 = local read "从板信息电压温度通道配置"() -> (w931:string[][])
                    n537 = Index Array(array=w931, index (col)=1 ("禁用的索引 (列)")) -> (element=w926:string[])  [unwired: 1 in]
                    n538 = Array Subset(array=w926, index=4 ("索引"), length=20 ("长度")) -> (w939:string[])
                    n539 = Array Subset(array=w926, index=24 ("索引"), length=20 ("长度")) -> (w928:string[])
                    n540 = for {
                      tunnel: w928 -> [w944] mode=indexing
                      tunnel: [w943] -> w927 mode=indexing
                      n541 = Fract/Exp String To Number(string=w944, default (0 dbl)=u8 0) -> (number=w943:u8)  [unwired: 2 in, 1 out]
                    }
                    n542 = for {
                      tunnel: w939 -> [w963] mode=indexing
                      shift-right: [w960] -> w933
                      shift-left: i32[] [] -> [w959]
                      n543 = Fract/Exp String To Number(string=w963, default (0 dbl)=u8 0) -> (number=w958:u8)  [unwired: 2 in, 1 out]
                      n544 = Equal To 0?(x=w958) -> (x = 0?=w961:bool)
                      n545 = Insert Into Array(array=w959, new element=w958) -> (w957:i32[])  [unwired: 1 in]
                      n546 = Select(t=w959, s=w961, f=w957) -> (s? t:f=w960:i32[])
                    }
                    n547 = Array Subset(array=w927, length=20 ("维数大小")) -> (w925:u8[])  [unwired: 1 in]
                    n548 = local write "5个通道电压个数(最少5个电压)"(w925) -> ()
                    n549 = Array Size(array=w933) -> (size(s)=w936:i32)
                    n550 = Quotient & Remainder(x=w936, y=2) -> (floor(x/y)=w934:i32)  [unwired: 1 out]
                    n551 = for {
                      N: w934 -> [_]
                      tunnel: w933 -> [w948]
                      tunnel: w932 -> [_]
                      i -> [w947]
                      n552 = Multiply(x=w947, y=2) -> (x*y=w955:i32)
                      n553 = Increment(x=w955) -> (x+1=w954:i32)
                      n554 = Index Array(array=w948, index #1=w955, index #2=w954) -> (element #1=w953:i32, element #2=w952:i32)
                      n555 = local read "保险位置"() -> (w945:T6)
                      n556 = Decrement(x=w953) -> (x-1=w950:i32)
                      n557 = Decrement(x=w952) -> (x-1=w949:i32)
                      n558 = Replace Array Subset(array=w945, new element=TRUE, index (row)=w950, index (col)=w949) -> (w946:T6)
                      n559 = local write "保险位置"(w946) -> ()
                    }
                    n560 = local write "保险位置"(w932) -> ()
                  }
                  frame True {
                  }
                }
              }
              frame #4 {
                n561 = case shown="假" w965 {
                  tunnel: w964 -> [w970 _]
                  frame False {
                    n562 = local write "自动记录"(TRUE ("自动记录")) -> ()
                    n563 = Number To Decimal String(number=w970) -> (decimal integer string=w969:string)  [unwired: 1 in]
                    n564 = Concatenate Strings("读取完成，配置文件为 一主" ("字符串"), w969, "从" ("字符串")) -> (w972:string)
                    n565 = One Button Dialog(message=w972, button name ("OK")="确定" ("按钮名称（“确定”）")) -> ()  [unwired: 1 out]
                  }
                  frame True {
                  }
                }
              }
            }
          }
        }
      }
      event "默认值": Value Change {
        n566 = event-data() -> ("NewVal"=w973:bool)  [unwired: 1 in, 5 out]
        n567 = case shown="真" w973 {
          frame False {
          }
          frame True {
            n568 = local write "加热控制参数"(T3 {"风机开启温度(℃)"=30.0, "风机关闭温度(℃)"=20.0, "加热开启温度(℃)"=10.0, "加热关闭温度(℃)"=15.0, "风机开启温差(℃)"=5.0, "风机关闭温差(℃)"=3.0, "加热关闭温差(℃)"=10.0} ("加热控制参数")) -> ()
            n569 = local write "充电控制参数"(T4 {"最大允许单体电压(V)"=4.15, "最大允许总电压(V)"=382.0, "最小允许单体电压(V)"=2.75, "最大允许充电电流(A)"=50.0, "最小允许充电电流(A)"=3.0, "最大允许充电温度(℃)"=55.0, "最小允许充电温度(℃)"=-15.0, "电流步长"=5.0} ("充电控制参数")) -> ()
            n570 = local write "一级故障"(dbl[][] [[389.0, 391.0, 395.0], [276.0, 253.0, 230.0], [50.0, 55.0, 60.0], [-20.0, -30.0, -40.0], [0.5, 1.0, 1.5], [0.5, 1.0, 1.5], [25.0, 30.0, 35.0], [25.0, 30.0, 35.0], [4.23, 4.25, 4.3], [3.0, 2.75, 2.5], [110.0, 132.0, 165.0], [250.0, 270.0, 300.0], [101.0, 101.0, 101.0], [30.0, 20.0, 10.0], [3.0, 5.0, 10.0], [50.0, 55.0, 60.0], [90.0, 80.0, 70.0]] ("一级故障")) -> ()
            n571 = local write "电池信息"(string[][] [["电池串联", "92"], ["电池并联", "2"], ["电池包额定容量", "67"], ["电池包额定能量", "0"], ["电池包额定总电压", "340"], ["实际容量", "67"], ["电池厂家", "普莱德"], ["电池类型", "磷酸铁锂"], ["电池生产日期", "2013-12-11 11:34:30"], ["电池包组号", "0"], ["累计充电总安时", "0"], ["累计放电总安时", "0"], ["电池放空次数", "0"], ["电池充满次数", "0"], ["电池充电次数", "0"]] ("电池信息")) -> ()
          }
        }
      }
      event "全部清零(主板)": Value Change {
        n572 = event-data() -> ("NewVal"=w978:bool)  [unwired: 1 in, 5 out]
        n573 = case shown="真" w978 {
          frame False {
          }
          frame True {
            n574 = local write "加热控制参数"(T3 {"风机开启温度(℃)"=0.0, "风机关闭温度(℃)"=0.0, "加热开启温度(℃)"=0.0, "加热关闭温度(℃)"=0.0, "风机开启温差(℃)"=0.0, "风机关闭温差(℃)"=0.0, "加热关闭温差(℃)"=0.0} ("加热控制参数")) -> ()
            n575 = control-ref of="主板信息"() -> (w986:refnum<vi>)
            n576 = local write "充电控制参数"(T4 {"最大允许单体电压(V)"=0.0, "最大允许总电压(V)"=0.0, "最小允许单体电压(V)"=0.0, "最大允许充电电流(A)"=0.0, "最小允许充电电流(A)"=0.0, "最大允许充电温度(℃)"=0.0, "最小允许充电温度(℃)"=0.0, "电流步长"=0.0} ("充电控制参数")) -> ()
            n577 = local write "一级故障"(dbl[][] [[0.0, 0.0, 0.0], [0.0, 0.0, 0.0], [0.0, 0.0, 0.0], [0.0, 0.0, 0.0], [0.0, 0.0, 0.0], [0.0, 0.0, 0.0], [0.0, 0.0, 0.0], [0.0, 0.0, 0.0], [0.0, 0.0, 0.0], [0.0, 0.0, 0.0], [0.0, 0.0, 0.0], [0.0, 0.0, 0.0], [0.0, 0.0, 0.0], [0.0, 0.0, 0.0], [0.0, 0.0, 0.0], [0.0, 0.0, 0.0], [0.0, 0.0, 0.0]] ("一级故障")) -> ()
            n578 = control-ref of="电池信息"() -> (w982:refnum<vi>)
            n579 = call "表格数据输入-8.6.vi"("行数"=u32 0, "列数"=u32 1, "字符串数组"=string[] ["", "", "", "", "", "", "", "", "", "", "", "", "", "", ""], "表格引用"=w982) -> ()  [unwired: 8 in]
            n580 = call "表格数据输入-8.6.vi"("行数"=u32 0, "列数"=u32 1, "字符串数组"=string[] ["", "", "", "", "", "", "", "", "", "", "", "", "", "", "", "", "", "", "", "", "", "", "", "", "", "", "", "", "", "", "", "", "", "", "", "", "", "", "", "", "", "", "", "", "", "", "", "", "", "", "", "", "", "", "", "", "", "", "", "", "", "", "", "", "", "", "", "", "", "", "", "", "", "", "", "", "", "", "", "", "", "", "", "", "", "", "", "", "", "", "", "", "", "", "", "", "", "", "", "", "", "", "", "", "", "", "", "", "", "", "", "", "", "", "", "", "", "", "", "", "", "", "", "", "", "", "", "", "", "", "", "", "", "", "", "", "", "", "", "", "", "", "", "", "", "", "", "", "", "", "", "", "", "", "", "", "", "", "", "", "", "", "", "", "", "", "", "", "", "", "", "", "", "", "", "", "", "", "", "", "", "", "", "", "", "", "", "", "", "", "", "", "", "", "", "", "", "", "", "", ""], "表格引用"=w986) -> ()  [unwired: 8 in]
          }
        }
      }
      event "读主板参数": Value Change {
        n581 = event-data() -> ("NewVal"=w991:bool)  [unwired: 1 in, 5 out]
        n582 = case shown="真" w991 {
          tunnel: w990 -> [_ w993]
          frame False {
          }
          frame True {
            n583 = call "文件对话框3"("prompt"="选择要读取的文件", "error in"=w993) -> ("selected path"=w994:path, "cancelled"=w995:bool, "error out"=w992:errorcluster)  [unwired: 10 in, 1 out]
            n584 = case shown="假" w995 {
              tunnel: w994 -> [w1002 _]
              tunnel: w992 -> [_ _]
              frame False {
                n585 = Strip Path(path=w1002) -> (name=w1001:string)  [unwired: 1 out]
                n586 = Match Pattern(string=w1001, regular expression="M" ("正则表达式")) -> (offset past match=w999:i32)  [unwired: 1 in, 3 out]
                n587 = Equal?(x=w999, y=-1) -> (x = y?=w997:bool)
                n588 = case shown="假" w997 {
                  tunnel: w1002 -> [w1003 _]
                  frame False {
                    n589 = stacked-sequence {
                      seq-local: [w1025 _ _ _] -> [_ _ _ w1156]
                      seq-local: [w1010 _ _ _] -> [_ w1040 _ _]
                      seq-local: [w1013 _ _ _] -> [_ w1045 w1112 w1133]
                      seq-local: [string[] ["电池额定容量", "电池实际容量", "SOC", "SOH", "产品编号", "车架(牌)号", "配置文件版本"] _ _ _] -> [_ _ _ w1162]
                      tunnel: w1003 -> [w1035 _ _ _]
                      frame #0 {
                        n590 = call-poly <vilib>:"Read From Spreadsheet File.vi"("file path (dialog if empty)"=w1035) -> ("all rows"=w1013:string[][])  [unwired: 6 in, 4 out]
                        n591 = Index Array(array=w1013, index (col)=3 ("禁用的索引 (列)")) -> (element=w1033:string[])  [unwired: 1 in]
                        n592 = Index Array(array=w1033) -> (element #1=w1032:string, element #2=w1031:string, element #3=w1030:string, element #4=w1029:string, element #5=w1027:string, element #6=w1026:string, element #7=w1028:string, element #9=w1024:string, element #10=w1023:string, element #11=w1022:string, element #12=w1008:string, element #13=w1007:string, element #14=w1006:string, element #15=w1004:string, element #16=w1005:string, element #17=w1021:string, element #18=w1020:string, element #19=w1019:string, element #20=w1018:string, element #21=w1017:string, element #22=w1016:string, element #23=w1015:string, element #24=w1014:string, element #25=w1009:string)  [unwired: 25 in, 1 out]
                        n593 = Build Array(w1032, w1031, w1030, w1029, w1028, w1027, w1026) -> (w1025:string[])
                        n594 = Build Array(w1024, w1023, w1022, w1008, w1006, w1007, w1005, w1004, w1021, w1020, w1019, w1018, w1017, w1016, w1015, w1014, w1009) -> (w1011:string[])
                        n595 = for {
                          tunnel: w1011 -> [w1037] mode=indexing
                          tunnel: [w1036] -> w1010 mode=indexing
                          n596 = Fract/Exp String To Number(string=w1037) -> (number=w1036:dbl)  [unwired: 3 in, 1 out]
                        }
                      }
                      frame #1 {
                        n597 = Index Array(array=w1045, index (col)=7 ("禁用的索引 (列)")) -> (element=w1047:string[])  [unwired: 1 in]
                        n598 = Index Array(array=w1045, index (col)=5 ("禁用的索引 (列)")) -> (element=w1082:string[])  [unwired: 1 in]
                        n599 = Index Array(array=w1047) -> (element #1=w1048:string, element #2=w1049:string, element #3=w1050:string, element #4=w1051:string, element #5=w1053:string, element #6=w1052:string, element #7=w1055:string, element #8=w1054:string, element #9=w1056:string, element #10=w1057:string, element #11=w1058:string, element #12=w1059:string, element #13=w1060:string, element #14=w1061:string, element #15=w1062:string, element #16=w1063:string, element #17=w1064:string)  [unwired: 17 in]
                        n600 = Index Array(array=w1082) -> (element #1=w1081:string, element #2=w1080:string, element #3=w1079:string, element #4=w1078:string, element #5=w1076:string, element #6=w1077:string, element #7=w1074:string, element #8=w1075:string, element #9=w1073:string, element #10=w1072:string, element #11=w1071:string, element #12=w1070:string, element #13=w1069:string, element #14=w1068:string, element #15=w1067:string, element #16=w1066:string, element #17=w1065:string)  [unwired: 17 in]
                        n601 = Build Array(w1048, w1049, w1050, w1051, w1052, w1053, w1054, w1055, w1056, w1057, w1058, w1059, w1060, w1061, w1062, w1063, w1064) -> (w1043:string[])
                        n602 = Build Array(w1081, w1080, w1079, w1078, w1077, w1076, w1075, w1074, w1073, w1072, w1071, w1070, w1069, w1068, w1067, w1066, w1065) -> (w1044:string[])
                        n603 = for {
                          tunnel: w1043 -> [w1085] mode=indexing
                          tunnel: [w1084] -> w1038 mode=indexing
                          n604 = Fract/Exp String To Number(string=w1085) -> (number=w1084:dbl)  [unwired: 3 in, 1 out]
                        }
                        n605 = for {
                          tunnel: w1044 -> [w1087] mode=indexing
                          tunnel: [w1086] -> w1039 mode=indexing
                          n606 = Fract/Exp String To Number(string=w1087) -> (number=w1086:dbl)  [unwired: 3 in, 1 out]
                        }
                        n607 = Build Array(w1040, w1039, w1038) -> (w1042:dbl[][])
                        n608 = Transpose 2D Array(2D array=w1042) -> (transposed array=w1041:dbl[][])
                        n609 = local write "一级故障"(w1041) -> ()
                      }
                      frame #2 {
                        n610 = Index Array(array=w1112, index (col)=11 ("禁用的索引 (列)")) -> (element=w1111:string[])  [unwired: 1 in]
                        n611 = Index Array(array=w1112, index (col)=9 ("禁用的索引 (列)")) -> (element=w1121:string[])  [unwired: 1 in]
                        n612 = Delete From Array(array=w1111, length=6 ("长度"), index=0 ("索引")) -> (deleted portion=w1108:string[], array with subset deleted=w1107:string[])
                        n613 = for {
                          tunnel: w1121 -> [w1124] mode=indexing
                          tunnel: [w1123] -> w1120 mode=indexing
                          n614 = Fract/Exp String To Number(string=w1124) -> (number=w1123:dbl)  [unwired: 3 in, 1 out]
                        }
                        n615 = Index Array(array=w1107) -> (element #1=w1106:string, element #2=w1105:string, element #3=w1096:string, element #4=w1095:string, element #5=w1104:string, element #6=w1103:string, element #7=w1102:string, element #8=w1093:string, element #9=w1094:string, element #10=w1092:string, element #11=w1101:string)  [unwired: 11 in]
                        n616 = Index Array(array=w1108) -> (element #1=w1098:string, element #2=w1100:string, element #3=w1099:string, element #4=w1097:string)  [unwired: 4 in]
                        n617 = Delete From Array(array=w1120, length=7 ("长度"), index=0 ("索引")) -> (deleted portion=w1115:dbl[], array with subset deleted=w1114:dbl[])
                        n618 = Array To Cluster(array=w1114) -> (cluster=w1117:T12)
                        n619 = Array To Cluster(array=w1115) -> (cluster=w1116:T10)
                        n620 = Build Array(w1106, w1105, w1104, w1103, w1102, w1101, w1100, w1099, w1098, w1097, w1096, w1095, w1094, w1093, w1092) -> (w1089:string[])
                        n621 = local write "加热控制参数"(w1116) -> ()
                        n622 = local write "充电控制参数"(w1117) -> ()
                        n623 = Build Array(string[] ["电池串联", "电池并联", "电池包额定容量", "电池包额定能量", "电池包额定总电压", "实际容量", "电池厂家", "电池类型", "电池生产日期", "电池包组号", "累计充电总安时", "累计放电总安时", "电池放空次数", "电池充满次数", "电池充电次数"], w1089) -> (w1091:string[][])
                        n624 = Transpose 2D Array(2D array=w1091) -> (transposed array=w1088:string[][])
                        n625 = local write "电池信息"(w1088) -> ()
                      }
                      frame #3 {
                        w1163 = 20
                        w1173 = 20 ("长度")
                        # "电池信息1"
                        n626 = Index Array(array=w1133, index (col)=1 ("禁用的索引 (列)")) -> (element=w1145:string[])  [unwired: 1 in]
                        n627 = Index Array(array=w1133, index (col)=0 ("禁用的索引 (列)")) -> (element=w1141:string[])  [unwired: 1 in]
                        n628 = Index Array(array=w1145, index=0 ("索引")) -> (element=w1177:string)
                        n629 = Search 1D Array(1D array=w1141, element="主板电压起始值" ("元素")) -> (index of element=w1171:i32)  [unwired: 1 in]
                        n630 = Search 1D Array(1D array=w1141, element="主板电池节数" ("元素")) -> (index of element=w1175:i32)  [unwired: 1 in]
                        n631 = Search 1D Array(1D array=w1141, element="主板温度个数" ("元素")) -> (index of element=w1170:i32)  [unwired: 1 in]
                        n632 = Search 1D Array(1D array=w1141, element="主板温度起始值" ("元素")) -> (index of element=w1167:i32)  [unwired: 1 in]
                        n633 = Search 1D Array(1D array=w1141, element="第1通道电压个数" ("元素")) -> (index of element=w1174:i32)  [unwired: 1 in]
                        n634 = Search 1D Array(1D array=w1141, element="第一个保险通道" ("元素")) -> (index of element=w1165:i32)  [unwired: 1 in]
                        n635 = Decimal String To Number(string=w1177) -> (number=w1142:i32)  [unwired: 2 in, 1 out]
                        n636 = Increment(x=w1142) -> (x+1=w1166:i32)
                        n637 = Array Subset(array=w1145, index=w1174, length=w1173) -> (w1150:string[])
                        n638 = Array Subset(array=w1141, index=w1175, length=w1166) -> (w1146:string[])
                        n639 = Array Subset(array=w1141, index=w1174, length=w1173) -> (w1157:string[])
                        n640 = Array Subset(array=w1145, index=w1171, length=w1166) -> (w1154:string[])
                        n641 = Array Subset(array=w1141, index=w1171, length=w1166) -> (w1161:string[])
                        n642 = Array Subset(array=w1145, index=w1170, length=w1166) -> (w1153:string[])
                        n643 = Array Subset(array=w1145, index=w1167, length=w1166) -> (w1152:string[])
                        n644 = Array Subset(array=w1141, index=w1170, length=w1166) -> (w1160:string[])
                        n645 = Array Subset(array=w1141, index=w1167, length=w1166) -> (w1159:string[])
                        n646 = Array Subset(array=w1145, index=w1165, length=w1163) -> (w1151:string[])
                        n647 = Array Subset(array=w1141, index=w1165, length=w1163) -> (w1158:string[])
                        n648 = Array Subset(array=w1145, index=w1175, length=w1166) -> (w1155:string[])
                        n649 = local write "从板个数"(w1142) -> ()
                        n650 = Insert Into Array(array=w1156, new element #1=w1155, new element #2=w1154, new element #3=w1153, new element #4=w1152, new element #5=w1151, new element #6=w1150) -> (w1148:string[])  [unwired: 1 in]
                        n651 = Multiply(x=w1142, y=2.0) -> (x*y=w1138:dbl)
                        n652 = Array Subset(array=w1145, index=1 ("索引"), length=w1138) -> (w1127:string[])
                        n653 = Insert Into Array(array=w1162, new element #1=w1146, new element #2=w1161, new element #3=w1160, new element #4=w1159, new element #5=w1158, new element #6=w1157) -> (w1149:string[])  [unwired: 1 in]
                        n654 = Array Subset(array=w1141, index=1 ("索引"), length=w1138) -> (w1131:string[])
                        n655 = Build Array(w1149, w1148) -> ()  [unwired: 1 out]
                        n656 = Index Array(array=w1133, index (col)=2 ("禁用的索引 (列)")) -> (element=w1136:string[])  [unwired: 1 in]
                        n657 = Index Array(array=w1133, index (col)=3 ("禁用的索引 (列)")) -> (element=w1135:string[])  [unwired: 1 in]
                        n658 = Array Subset(array=w1136, length=7 ("索引")) -> (w1132:string[])  [unwired: 1 in]
                        n659 = Array Subset(array=w1135, length=7 ("索引")) -> (w1129:string[])  [unwired: 1 in]
                        n660 = Insert Into Array(array=w1132, new element=w1131) -> (w1130:string[])  [unwired: 1 in]
                        n661 = Insert Into Array(array=w1129, new element=w1127) -> (w1128:string[])  [unwired: 1 in]
                        n662 = Build Array(w1130, w1128) -> (w1139:string[][])
                        n663 = Transpose 2D Array(2D array=w1139) -> (transposed array=w1147:string[][])
                        n664 = local write "主板信息"(w1147) -> ()
                      }
                    }
                  }
                  frame True {
                    n665 = One Button Dialog(message="选择文件类型错误" ("消息"), button name ("OK")="确定" ("按钮名称（“确定”）")) -> ()  [unwired: 1 out]
                  }
                }
              }
              frame True {
              }
            }
          }
        }
      }
      event "读从板参数": Value Change {
        n666 = event-data() -> ("NewVal"=w1186:bool)  [unwired: 1 in, 5 out]
        n667 = case shown="真" w1186 {
          tunnel: w1185 -> [_ w1189]
          tunnel: w1184 -> [_ w1187]
          frame False {
          }
          frame True {
            n668 = call "文件对话框4"("prompt"="选择要读取的文件", "error in"=w1189) -> ("selected path"=w1190:path, "cancelled"=w1191:bool, "error out"=w1188:errorcluster)  [unwired: 10 in, 1 out]
            n669 = case shown="假" w1191 {
              tunnel: w1190 -> [w1194 _]
              tunnel: w1188 -> [_ _]
              tunnel: w1187 -> [w1193 _]
              frame False {
                n670 = Strip Path(path=w1194) -> (name=w1199:string)  [unwired: 1 out]
                n671 = Match Pattern(string=w1199, regular expression="S" ("正则表达式")) -> (offset past match=w1197:i32)  [unwired: 1 in, 3 out]
                n672 = Equal?(x=w1197, y=-1) -> (x = y?=w1195:bool)
                n673 = case shown="假" w1195 {
                  tunnel: w1194 -> [w1201 _]
                  tunnel: w1193 -> [w1200 _]
                  frame False {
                    n674 = stacked-sequence {
                      seq-local: [w1219 _ _ _ _] -> [_ w1225 w1258 _ _]
                      seq-local: [w1204 _ _ _ _] -> [_ _ _ _ w1304]
                      seq-local: [w1202 _ _ _ _] -> [_ _ _ _ w1303]
                      seq-local: [_ _ w1243 _ _] -> [_ _ _ _ w1305]
                      seq-local: [_ _ w1242 _ _] -> [_ _ _ w1270 w1306]
                      seq-local: [_ w1224 _ _ _] -> [_ _ _ _ w1298]
                      tunnel: w1201 -> [w1220 _ _ _ _]
                      tunnel: w1200 -> [_ _ w1236 _ _]
                      frame #0 {
                        n675 = call-poly <vilib>:"Read From Spreadsheet File.vi"("file path (dialog if empty)"=w1220) -> ("all rows"=w1219:string[][])  [unwired: 6 in, 4 out]
                        n676 = Index Array(array=w1219, index (col)=3 ("禁用的索引 (列)")) -> (element=w1218:string[])  [unwired: 1 in]
                        n677 = for {
                          tunnel: w1218 -> [w1223] mode=indexing
                          tunnel: [w1222] -> w1217 mode=indexing
                          n678 = Fract/Exp String To Number(string=w1223) -> (number=w1222:dbl)  [unwired: 3 in, 1 out]
                        }
                        n679 = Delete From Array(array=w1217, length=7 ("长度"), index=0 ("索引")) -> (deleted portion=w1205:dbl[], array with subset deleted=w1214:dbl[])
                        n680 = Delete From Array(array=w1214, length=7 ("索引"), index=0 ("索引")) -> (deleted portion=w1208:dbl[], array with subset deleted=w1209:dbl[])
                        n681 = Array To Cluster(array=w1205) -> (cluster=w1204:T10)
                        n682 = Delete From Array(array=w1209, length=7 ("索引"), index=0 ("索引")) -> (deleted portion=w1207:dbl[], array with subset deleted=w1206:dbl[])
                        n683 = local write "加热控制参数 2"(w1204) -> ()
                        n684 = Build Array(w1208, w1207, w1206) -> (w1203:dbl[][])
                        n685 = Transpose 2D Array(2D array=w1203) -> (transposed array=w1202:dbl[][])
                        n686 = local write "一级故障 2"(w1202) -> ()
                      }
                      frame #1 {
                        n687 = disable-structure shown="禁用" {
                          disable-tunnel: w1225 -> [w1229 _]
                          disable-tunnel: [w1228 _] -> w1224
                          frame Disabled {
                            n688 = Index Array(array=w1229, index (col)=7 ("禁用的索引 (列)")) -> (element=w1228:string[])  [unwired: 1 in]
                            n689 = for {
                              tunnel: w1228 -> [w1232] mode=indexing
                              tunnel: [w1231] -> w1227 mode=indexing
                              n690 = Fract/Exp String To Number(string=w1232) -> (number=w1231:dbl)  [unwired: 3 in, 1 out]
                            }
                            n691 = Array To Cluster(array=w1227) -> (cluster=w1226:T13)
                            n692 = local write "均衡参数"(w1226) -> ()
                          }
                          frame Enabled {
                          }
                        }
                      }
                      frame #2 {
                        # "第一个保险位置"
                        # "温度个数"
                        # "通道电压节数"
                        # "电压节数"
                        n693 = Index Array(array=w1258, index (col)=1 ("禁用的索引 (列)")) -> (element=w1240:string[])  [unwired: 1 in]
                        n694 = Index Array(array=w1240, index=0 ("索引")) -> (element=w1257:string)
                        n695 = Decimal String To Number(string=w1257) -> (number=w1243:i32)  [unwired: 2 in, 1 out]
                        n696 = Array Subset(array=w1240, index=3 ("禁用的索引 (列)"), length=20 ("禁用的索引 (列)")) -> (w1244:string[])
                        n697 = Array Subset(array=w1240, index=23 ("禁用的索引 (列)"), length=2 ("禁用的索引 (列)")) -> (w1246:string[])
                        n698 = Array Subset(array=w1240, index=1 ("禁用的索引 (列)"), length=2 ("禁用的索引 (列)")) -> (w1247:string[])
                        n699 = Array Subset(array=w1240, index=25 ("禁用的索引 (列)"), length=20 ("禁用的索引 (列)")) -> (w1245:string[])
                        n700 = local write "从板板号"(w1243) -> ()
                        n701 = Array Subset(array=w1240, index=1 ("索引"), length=27 ("长度")) -> (w1237:string[])
                        n702 = Insert Into Array(array=w1247, new element #1=w1246, new element #2=w1245, new element #3=w1244) -> ()  [unwired: 1 in, 1 out]
                        n703 = Array Subset(array=w1236, index=1 ("索引"), length=27 ("长度")) -> (w1235:string[])
                        n704 = Build Array(w1235, w1237) -> (w1256:string[][])
                        n705 = Transpose 2D Array(2D array=w1256) -> (transposed array=w1242:string[][])
                        n706 = local write "保险位置"(bool[][] [[FALSE, FALSE, FALSE, FALSE, FALSE, FALSE, FALSE, FALSE, FALSE, FALSE, FALSE, FALSE], [FALSE, FALSE, FALSE, FALSE, FALSE, FALSE, FALSE, FALSE, FALSE, FALSE, FALSE, FALSE], [FALSE, FALSE, FALSE, FALSE, FALSE, FALSE, FALSE, FALSE, FALSE, FALSE, FALSE, FALSE], [FALSE, FALSE, FALSE, FALSE, FALSE, FALSE, FALSE, FALSE, FALSE, FALSE, FALSE, FALSE], [FALSE, FALSE, FALSE, FALSE, FALSE, FALSE, FALSE, FALSE, FALSE, FALSE, FALSE, FALSE], [FALSE, FALSE, FALSE, FALSE, FALSE, FALSE, FALSE, FALSE, FALSE, FALSE, FALSE, FALSE], [FALSE, FALSE, FALSE, FALSE, FALSE, FALSE, FALSE, FALSE, FALSE, FALSE, FALSE, FALSE], [FALSE, FALSE, FALSE, FALSE, FALSE, FALSE, FALSE, FALSE, FALSE, FALSE, FALSE, FALSE], [FALSE, FALSE, FALSE, FALSE, FALSE, FALSE, FALSE, FALSE, FALSE, FALSE, FALSE, FALSE], [FALSE, FALSE, FALSE, FALSE, FALSE, FALSE, FALSE, FALSE, FALSE, FALSE, FALSE, FALSE]]) -> ()
                        n707 = local write "从板信息电压温度通道配置"(w1242) -> ()
                      }
                      frame #3 {
                        n708 = Index Array(array=w1270, index (col)=1 ("禁用的索引 (列)")) -> (element=w1262:string[])  [unwired: 1 in]
                        n709 = Array Subset(array=w1262, index=4 ("索引"), length=20 ("长度")) -> (w1273:string[])
                        n710 = Array Subset(array=w1262, index=24 ("索引"), length=20 ("长度")) -> (w1263:string[])
                        n711 = for {
                          tunnel: w1273 -> [w1297] mode=indexing
                          shift-right: [w1294] -> w1266
                          shift-left: i32[] [] -> [w1293]
                          n712 = Fract/Exp String To Number(string=w1297, default (0 dbl)=u8 0) -> (number=w1292:u8)  [unwired: 2 in, 1 out]
                          n713 = Equal To 0?(x=w1292) -> (x = 0?=w1295:bool)
                          n714 = Insert Into Array(array=w1293, new element=w1292) -> (w1291:i32[])  [unwired: 1 in]
                          n715 = Select(t=w1293, s=w1295, f=w1291) -> (s? t:f=w1294:i32[])
                        }
                        n716 = for {
                          tunnel: w1263 -> [w1278] mode=indexing
                          tunnel: [w1277] -> w1261 mode=indexing
                          n717 = Fract/Exp String To Number(string=w1278, default (0 dbl)=u8 0) -> (number=w1277:u8)  [unwired: 2 in, 1 out]
                        }
                        n718 = local write "5个通道电压个数(最少5个电压)"(w1261) -> ()
                        n719 = Array Size(array=w1266) -> (size(s)=w1269:i32)
                        n720 = Quotient & Remainder(x=w1269, y=2) -> (floor(x/y)=w1267:i32)  [unwired: 1 out]
                        n721 = for {
                          N: w1267 -> [_]
                          tunnel: w1266 -> [w1282]
                          i -> [w1281]
                          n722 = Multiply(x=w1281, y=2) -> (x*y=w1289:i32)
                          n723 = Increment(x=w1289) -> (x+1=w1288:i32)
                          n724 = Index Array(array=w1282, index #1=w1289, index #2=w1288) -> (element #1=w1287:i32, element #2=w1286:i32)
                          n725 = local read "保险位置"() -> (w1279:T6)
                          n726 = Decrement(x=w1287) -> (x-1=w1284:i32)
                          n727 = Decrement(x=w1286) -> (x-1=w1283:i32)
                          n728 = Replace Array Subset(array=w1279, new element=TRUE, index (row)=w1284, index (col)=w1283) -> (w1280:T6)
                          n729 = local write "保险位置"(w1280) -> ()
                        }
                      }
                      frame #4 {
                        n730 = Transpose 2D Array(2D array=w1303) -> (transposed array=w1312:dbl[][])
                        n731 = Array Subset(array=w1306, index (row)=0 ("索引"), index (col)=0 ("索引"), length (col)=2 ("索引")) -> (w1323:string[][])  [unwired: 1 in]
                        n732 = for {
                          tunnel: w1312 -> [w1341] mode=indexing
                          shift-right: [w1340] -> w1320
                          shift-left: string[] [] -> [w1338]
                          n733 = for {
                            N: 7 -> [_]
                            tunnel: w1341 -> [w1344] mode=indexing
                            tunnel: [w1342] -> w1339 mode=indexing
                            n734 = Format Into String(format string="%#f" ("格式字符串"), w1344) -> (resulting string=w1342:string)  [unwired: 2 in, 1 out]
                          }
                          n735 = Insert Into Array(array=w1338, new element=w1339) -> (w1340:string[])  [unwired: 1 in]
                        }
                        n736 = Cluster To Array(cluster=w1304) -> (array=w1325:dbl[])
                        n737 = Index Array(array=w1323, index (col) #1=0 ("禁用的索引 (列)"), index (col) #2=1 ("索引 (列)")) -> (element #1=w1311:string[], element #2=w1313:string[])  [unwired: 2 in]
                        n738 = for {
                          tunnel: w1325 -> [w1347] mode=indexing
                          tunnel: [w1345] -> w1321 mode=indexing
                          n739 = Format Into String(format string="%#f" ("格式字符串"), w1347) -> (resulting string=w1345:string)  [unwired: 2 in, 1 out]
                        }
                        n740 = Insert Into Array(array=w1311, index=0 ("索引"), new element="从板板号" ("新元素/子数组")) -> (w1308:string[])
                        n741 = Number To Decimal String(number=w1305) -> (decimal integer string=w1315:string)  [unwired: 1 in]
                        n742 = Insert Into Array(array=w1308, new element=string[] ["从板板号", "电压个数", "电压起始值", "温度个数", "温度起始值", "第一个保险通道", "第一个保险位置", "第二个保险通道", "第二个保险位置", "第三个保险通道", "第三个保险位置", "第四个保险通道", "第四个保险位置", "第五个保险通道", "第五个保险位置", "第六个保险通道", "第六个保险位置", "第七个保险通道", "第七个保险位置", "第八个保险通道", "第八个保险位置", "第九个保险通道", "第九个保险位置", "第十个保险通道", "第十个保险位置", "第1通道电压个数", "第2通道电压个数", "第3通道电压个数", "第4通道电压个数", "第5通道电压个数", "第6通道电压个数", "第7通道电压个数", "第8通道电压个数", "第9通道电压个数", "第10通道电压个数", "第11通道电压个数", "第12通道电压个数", "第13通道电压个数", "第14通道电压个数", "第15通道电压个数", "第16通道电压个数", "第17通道电压个数", "第18通道电压个数", "第19通道电压个数", "第20通道电压个数", "风机开启温度", "风机关闭温度", "加热开启温度", "加热关闭温度", "风机开启温差", "风机关闭温差", "加热关闭温差", "电压过高一级", "电压过低一级", "温度过高一级", "温度过低一级", "电压不均衡一级", "温度不均衡一级", "SOC过低一级", "电压过高二级", "电压过低二级", "温度过高二级", "温度过低二级", "电压不均衡二级", "温度不均衡二级", "SOC过低二级", "电压过高三级", "电压过低三级", "温度过高三级", "温度过低三级", "电压不均衡三级", "温度不均衡三级", "SOC过低三级", "均衡计算-电压高阀值1级", "均衡计算-电压高阀值2级", "均衡计算-电压低阀值1级", "均衡计算-电压低阀值2级", "均衡计算-最低电压阀值", "均衡停止-最低电压阀值", "均衡计算-电压极差阀值", "充电结束电压(90%)", "充电结束电压(91%)", "充电结束电压(92%)", "充电结束电压(93%)", "充电结束电压(94%)", "充电结束电压(95%)", "充电结束电压(96%)", "充电结束电压(97%)", "充电结束电压(98%)", "充电结束电压(99%)", "充电结束电压(100%)"] ("从板表头")) -> (w1302:string[])  [unwired: 1 in]
                        n743 = local read "输出数组"() -> (w1301:string[][])
                        n744 = Insert Into Array(array=w1313, new element #1=w1321, new element #2=w1320, new element #3=w1298) -> (w1319:string[])  [unwired: 1 in]
                        n745 = Decrement(x=w1305) -> (x-1=w1300:i32)
                        n746 = local write "从板表头"(w1302) -> ()
                        n747 = Insert Into Array(array=w1319, index=0 ("索引"), new element=w1315) -> (w1317:string[])
                        n748 = Replace Array Subset(array=w1301, new element=w1317, index (col)=w1300) -> (w1316:string[][])  [unwired: 1 in]
                        n749 = stacked-sequence {
                          tunnel: w1316 -> [w1329]
                          tunnel: w1315 -> [w1334]
                          frame #0 {
                            n750 = control-ref of="结果"() -> (w1336:refnum<vi>)
                            n751 = Concatenate Strings("从板", w1334, "记录完成") -> (w1332:string)
                            n752 = local write "输出数组"(w1329) -> ()
                            n753 = Build Array(w1332) -> (w1330:string[])
                            n754 = call "表格编辑.vi"("新元素/子数组"=w1330, "活动单元格:单元格背景色"=u32 6618880, "MCListbox引用句柄"=w1336) -> ()  [unwired: 9 in]
                          }
                        }
                        n755 = property on="查看" class="Bool (严格)"("Visible"=TRUE ("可见")) -> ()  [unwired: 2 in, 2 out]
                      }
                    }
                  }
                  frame True {
                    n756 = One Button Dialog(message="选择文件类型错误" ("消息"), button name ("OK")="确定" ("按钮名称（“确定”）")) -> ()  [unwired: 1 out]
                  }
                }
              }
              frame True {
              }
            }
          }
        }
      }
      event "从板信息电压温度通道配置": Value Change {
        w1350 = bool[][] [[FALSE, FALSE, FALSE, FALSE, FALSE, FALSE, FALSE, FALSE, FALSE, FALSE, FALSE, FALSE], [FALSE, FALSE, FALSE, FALSE, FALSE, FALSE, FALSE, FALSE, FALSE, FALSE, FALSE, FALSE], [FALSE, FALSE, FALSE, FALSE, FALSE, FALSE, FALSE, FALSE, FALSE, FALSE, FALSE, FALSE], [FALSE, FALSE, FALSE, FALSE, FALSE, FALSE, FALSE, FALSE, FALSE, FALSE, FALSE, FALSE], [FALSE, FALSE, FALSE, FALSE, FALSE, FALSE, FALSE, FALSE, FALSE, FALSE, FALSE, FALSE], [FALSE, FALSE, FALSE, FALSE, FALSE, FALSE, FALSE, FALSE, FALSE, FALSE, FALSE, FALSE], [FALSE, FALSE, FALSE, FALSE, FALSE, FALSE, FALSE, FALSE, FALSE, FALSE, FALSE, FALSE], [FALSE, FALSE, FALSE, FALSE, FALSE, FALSE, FALSE, FALSE, FALSE, FALSE, FALSE, FALSE], [FALSE, FALSE, FALSE, FALSE, FALSE, FALSE, FALSE, FALSE, FALSE, FALSE, FALSE, FALSE], [FALSE, FALSE, FALSE, FALSE, FALSE, FALSE, FALSE, FALSE, FALSE, FALSE, FALSE, FALSE]]
        n757 = event-data() -> ("NewVal"=w1351:string[][])  [unwired: 1 in, 5 out]
        n758 = Index Array(array=w1351, index (col)=1 ("禁用的索引 (列)")) -> (element=w1353:string[])  [unwired: 1 in]
        n759 = Array Subset(array=w1353, index=4 ("索引"), length=20 ("长度")) -> (w1363:string[])
        n760 = Array Subset(array=w1353, index=24 ("索引"), length=20 ("长度")) -> (w1354:string[])
        n761 = for {
          tunnel: w1363 -> [w1387] mode=indexing
          shift-right: [w1384] -> w1357
          shift-left: i32[] [] -> [w1383]
          n762 = Fract/Exp String To Number(string=w1387, default (0 dbl)=u8 0) -> (number=w1382:u8)  [unwired: 2 in, 1 out]
          n763 = Equal To 0?(x=w1382) -> (x = 0?=w1385:bool)
          n764 = Insert Into Array(array=w1383, new element=w1382) -> (w1381:i32[])  [unwired: 1 in]
          n765 = Select(t=w1383, s=w1385, f=w1381) -> (s? t:f=w1384:i32[])
        }
        n766 = for {
          tunnel: w1354 -> [w1368] mode=indexing
          tunnel: [w1367] -> w1352 mode=indexing
          n767 = Fract/Exp String To Number(string=w1368, default (0 dbl)=u8 0) -> (number=w1367:u8)  [unwired: 2 in, 1 out]
        }
        n768 = local write "5个通道电压个数(最少5个电压)"(w1352) -> ()
        n769 = Array Size(array=w1357) -> (size(s)=w1360:i32)
        n770 = Quotient & Remainder(x=w1360, y=2) -> (floor(x/y)=w1358:i32)  [unwired: 1 out]
        n771 = for {
          N: w1358 -> [_]
          tunnel: w1357 -> [w1372]
          tunnel: w1350 -> [_]
          i -> [w1371]
          n772 = Multiply(x=w1371, y=2) -> (x*y=w1379:i32)
          n773 = Increment(x=w1379) -> (x+1=w1378:i32)
          n774 = Index Array(array=w1372, index #1=w1379, index #2=w1378) -> (element #1=w1377:i32, element #2=w1376:i32)
          n775 = local read "保险位置"() -> (w1369:T6)
          n776 = Decrement(x=w1377) -> (x-1=w1374:i32)
          n777 = Decrement(x=w1376) -> (x-1=w1373:i32)
          n778 = Replace Array Subset(array=w1369, new element=TRUE, index (row)=w1374, index (col)=w1373) -> (w1370:T6)
          n779 = local write "保险位置"(w1370) -> ()
        }
        n780 = local write "保险位置"(w1350) -> ()
      }
      event "从板板号": Value Change {
        n781 = event-data() -> ("NewVal"=w1391:dbl)  [unwired: 1 in, 5 out]
        n782 = Decrement(x=w1391) -> (x-1=w1395:dbl)
        n783 = local read "输出数组"() -> (w1396:string[][])
        n784 = Index Array(array=w1396, index (col)=w1395) -> (element=w1394:string[])  [unwired: 1 in]
        n785 = Index Array(array=w1394, index=0 ("索引")) -> (element=w1390:string)
        n786 = Decimal String To Number(string=w1390) -> (number=w1389:i32)  [unwired: 2 in, 1 out]
        n787 = Equal?(x=w1389, y=w1391) -> (x = y?=w1392:bool)
        n788 = case shown="真" w1392 {
          tunnel: w1394 -> [_ w1398]
          tunnel: w1388 -> [_ w1397]
          frame False {
          }
          frame True {
            n789 = stacked-sequence {
              seq-local: [_ w1407 _] -> [_ _ w1444]
              tunnel: w1398 -> [_ w1408 _]
              tunnel: w1397 -> [_ w1402 _]
              frame #0 {
                n790 = local write "一级故障 2"(dbl[][] [[0.0, 0.0, 0.0, 0.0, 0.0, 0.0, 0.0, 0.0, 0.0, 0.0, 0.0, 0.0, 0.0, 0.0, 0.0, 0.0, 0.0]] ("一级故障 2")) -> ()
                n791 = local write "从板信息电压温度通道配置"(string[][] [] ("key names")) -> ()
                n792 = local write "加热控制参数 2"(T9 {"风机开启温度"=0.0, "风机关闭温度"=0.0, "加热开启温度"=0.0, "加热关闭温度"=0.0, "风机开启温差"=0.0, "风机关闭温差"=0.0, "加热关闭温差"=0.0} ("加热控制参数 2")) -> ()
              }
              frame #1 {
                n793 = Search 1D Array(1D array=w1402, element="风机开启温度" ("元素")) -> (index of element=w1427:i32)  [unwired: 1 in]
                n794 = Search 1D Array(1D array=w1402, element="电压过高一级" ("元素"), start index (0)=w1427) -> (index of element=w1425:i32)
                n795 = Decrement(x=w1427) -> (x-1=w1429:i32)
                n796 = Array Subset(array=string[] ["从板板号", "电压个数", "温度个数", "第一个保险通道", "第一个保险位置", "第二个保险通道", "第二个保险位置", "第三个保险通道", "第三个保险位置", "第四个保险通道", "第四个保险位置", "第五个保险通道", "第五个保险位置", "第六个保险通道", "第六个保险位置", "第七个保险通道", "第七个保险位置", "第八个保险通道", "第八个保险位置", "第九个保险通道", "第九个保险位置", "第十个保险通道", "第十个保险位置", "第1通道电压个数", "第2通道电压个数", "第3通道电压个数", "第4通道电压个数", "第5通道电压个数", "第6通道电压个数", "第7通道电压个数", "第8通道电压个数", "第9通道电压个数", "第10通道电压个数", "第11通道电压个数", "第12通道电压个数", "第13通道电压个数", "第14通道电压个数", "第15通道电压个数", "第16通道电压个数", "第17通道电压个数", "第18通道电压个数", "第19通道电压个数", "第20通道电压个数", "风机开启温度", "风机关闭温度", "加热开启温度", "加热关闭温度", "风机开启温差", "风机关闭温差", "加热关闭温差", "电压过高一级", "电压过低一级", "温度过高一级", "温度过低一级", "电压不均衡一级", "温度不均衡一级", "SOC过低一级", "电压过高二级", "电压过低二级", "温度过高二级", "温度过低二级", "电压不均衡二级", "温度不均衡二级", "SOC过低二级", "电压过高三级", "电压过低三级", "温度过高三级", "温度过低三级", "电压不均衡三级", "温度不均衡三级", "SOC过低三级", "均衡计算-电压高阀值1级", "均衡计算-电压高阀值2级", "均衡计算-电压低阀值1级", "均衡计算-电压低阀值2级", "均衡计算-最低电压阀值", "均衡停止-最低电压阀值", "均衡计算-电压极差阀值", "充电结束电压(90%)", "充电结束电压(91%)", "充电结束电压(92%)", "充电结束电压(93%)", "充电结束电压(94%)", "充电结束电压(95%)", "充电结束电压(96%)", "充电结束电压(97%)", "充电结束电压(98%)", "充电结束电压(99%)", "充电结束电压(100%)"] ("从板表头"), index=1 ("长度"), length=27 ("长度")) -> (w1403:string[])
                n797 = Array Subset(array=w1408, index=1 ("索引"), length=w1429) -> (w1431:string[])
                n798 = Array Subset(array=w1408, index=w1425, length=21 ("长度")) -> (w1410:string[])
                n799 = Array Subset(array=w1408, index=w1427, length=7 ("长度")) -> (w1423:string[])
                n800 = for {
                  tunnel: w1410 -> [w1435] mode=indexing
                  tunnel: [w1434] -> w1409 mode=indexing
                  n801 = Fract/Exp String To Number(string=w1435) -> (number=w1434:dbl)  [unwired: 3 in, 1 out]
                }
                n802 = for {
                  tunnel: w1423 -> [w1437] mode=indexing
                  tunnel: [w1436] -> w1422 mode=indexing
                  n803 = Fract/Exp String To Number(string=w1437) -> (number=w1436:dbl)  [unwired: 3 in, 1 out]
                }
                n804 = Build Array(w1403, w1431) -> (w1430:string[][])
                n805 = Delete From Array(array=w1409, length=7 ("长度"), index=0 ("索引")) -> (deleted portion=w1418:dbl[], array with subset deleted=w1417:dbl[])
                n806 = Transpose 2D Array(2D array=w1430) -> (transposed array=w1407:string[][])
                n807 = Array To Cluster(array=w1422) -> (cluster=w1421:T10)
                n808 = Delete From Array(array=w1417, length=7 ("长度"), index=0 ("索引")) -> (deleted portion=w1414:dbl[], array with subset deleted=w1413:dbl[])
                n809 = local write "从板信息电压温度通道配置"(w1407) -> ()
                n810 = local write "加热控制参数 2"(w1421) -> ()
                n811 = Build Array(w1418, w1414, w1413) -> (w1412:dbl[][])
                n812 = Transpose 2D Array(2D array=w1412) -> (transposed array=w1411:dbl[][])
                n813 = local write "一级故障 2"(w1411) -> ()
              }
              frame #2 {
                w1449 = bool[][] [[FALSE, FALSE, FALSE, FALSE, FALSE, FALSE, FALSE, FALSE, FALSE, FALSE, FALSE, FALSE], [FALSE, FALSE, FALSE, FALSE, FALSE, FALSE, FALSE, FALSE, FALSE, FALSE, FALSE, FALSE], [FALSE, FALSE, FALSE, FALSE, FALSE, FALSE, FALSE, FALSE, FALSE, FALSE, FALSE, FALSE], [FALSE, FALSE, FALSE, FALSE, FALSE, FALSE, FALSE, FALSE, FALSE, FALSE, FALSE, FALSE], [FALSE, FALSE, FALSE, FALSE, FALSE, FALSE, FALSE, FALSE, FALSE, FALSE, FALSE, FALSE], [FALSE, FALSE, FALSE, FALSE, FALSE, FALSE, FALSE, FALSE, FALSE, FALSE, FALSE, FALSE], [FALSE, FALSE, FALSE, FALSE, FALSE, FALSE, FALSE, FALSE, FALSE, FALSE, FALSE, FALSE], [FALSE, FALSE, FALSE, FALSE, FALSE, FALSE, FALSE, FALSE, FALSE, FALSE, FALSE, FALSE], [FALSE, FALSE, FALSE, FALSE, FALSE, FALSE, FALSE, FALSE, FALSE, FALSE, FALSE, FALSE], [FALSE, FALSE, FALSE, FALSE, FALSE, FALSE, FALSE, FALSE, FALSE, FALSE, FALSE, FALSE]]
                n814 = Index Array(array=w1444, index (col)=1 ("禁用的索引 (列)")) -> (element=w1443:string[])  [unwired: 1 in]
                n815 = Array Subset(array=w1443, index=4 ("索引"), length=20 ("长度")) -> (w1456:string[])
                n816 = Array Subset(array=w1443, index=22 ("索引"), length=5 ("长度")) -> (w1446:string[])
                n817 = Index Array(array=w1443, index #1=0 ("索引")) -> (element #1=w1441:string, element #2=w1440:string)  [unwired: 1 in]
                n818 = for {
                  tunnel: w1446 -> [w1461] mode=indexing
                  tunnel: [w1460] -> w1445 mode=indexing
                  n819 = Fract/Exp String To Number(string=w1461, default (0 dbl)=u8 0) -> (number=w1460:u8)  [unwired: 2 in, 1 out]
                }
                n820 = for {
                  tunnel: w1456 -> [w1480] mode=indexing
                  shift-right: [w1477] -> w1450
                  shift-left: i32[] [] -> [w1476]
                  n821 = Fract/Exp String To Number(string=w1480, default (0 dbl)=u8 0) -> (number=w1475:u8)  [unwired: 2 in, 1 out]
                  n822 = Equal To 0?(x=w1475) -> (x = 0?=w1478:bool)
                  n823 = Insert Into Array(array=w1476, new element=w1475) -> (w1474:i32[])  [unwired: 1 in]
                  n824 = Select(t=w1476, s=w1478, f=w1474) -> (s? t:f=w1477:i32[])
                }
                n825 = Fract/Exp String To Number(string=w1440) -> (number=w1438:dbl)  [unwired: 3 in, 1 out]
                n826 = Fract/Exp String To Number(string=w1441) -> (number=w1439:dbl)  [unwired: 3 in, 1 out]
                n827 = local write "温度个数"(w1438) -> ()
                n828 = local write "电压个数"(w1439) -> ()
                n829 = local write "5个通道电压个数(最少5个电压)"(w1445) -> ()
                n830 = Array Size(array=w1450) -> (size(s)=w1453:i32)
                n831 = Quotient & Remainder(x=w1453, y=2) -> (floor(x/y)=w1451:i32)  [unwired: 1 out]
                n832 = for {
                  N: w1451 -> [_]
                  tunnel: w1450 -> [w1465]
                  tunnel: w1449 -> [_]
                  i -> [w1464]
                  n833 = Multiply(x=w1464, y=2) -> (x*y=w1472:i32)
                  n834 = Increment(x=w1472) -> (x+1=w1471:i32)
                  n835 = Index Array(array=w1465, index #1=w1472, index #2=w1471) -> (element #1=w1470:i32, element #2=w1469:i32)
                  n836 = local read "保险位置"() -> (w1462:T6)
                  n837 = Decrement(x=w1470) -> (x-1=w1467:i32)
                  n838 = Decrement(x=w1469) -> (x-1=w1466:i32)
                  n839 = Replace Array Subset(array=w1462, new element=TRUE, index (row)=w1467, index (col)=w1466) -> (w1463:T6)
                  n840 = local write "保险位置"(w1463) -> ()
                }
                n841 = local write "保险位置"(w1449) -> ()
              }
            }
          }
        }
      }
      event "查看": Value Change {
        n842 = event-data() -> ("NewVal"=w1481:bool)  [unwired: 1 in, 5 out]
        n843 = case shown="假" w1481 {
          frame False {
            n844 = call "选择从板号"() -> ("从板号"=w1482:dbl, "确定"=w1483:bool)  [unwired: 17 in, 1 out]
            n845 = case shown="真" w1483 {
              tunnel: w1482 -> [_ w1484]
              frame False {
              }
              frame True {
                n846 = local read "从板表头"() -> (w1485:string[])
                n847 = stacked-sequence {
                  tunnel: w1484 -> [_ w1497 w1529]
                  tunnel: w1485 -> [_ w1495 _]
                  frame #0 {
                    n848 = local write "从板信息电压温度通道配置"(string[][] [] ("key names")) -> ()
                    n849 = local write "一级故障 2"(dbl[][] [[0.0, 0.0, 0.0, 0.0, 0.0, 0.0, 0.0, 0.0, 0.0, 0.0, 0.0, 0.0, 0.0, 0.0, 0.0, 0.0, 0.0]] ("一级故障 2")) -> ()
                    n850 = local write "加热控制参数 2"(T9 {"风机开启温度"=0.0, "风机关闭温度"=0.0, "加热开启温度"=0.0, "加热关闭温度"=0.0, "风机开启温差"=0.0, "风机关闭温差"=0.0, "加热关闭温差"=0.0} ("加热控制参数 2")) -> ()
                  }
                  frame #1 {
                    n851 = local read "输出数组"() -> (w1496:string[][])
                    n852 = Decrement(x=w1497) -> (x-1=w1493:dbl)
                    n853 = Index Array(array=w1496, index (col)=w1493) -> (element=w1515:string[])  [unwired: 1 in]
                    n854 = Search 1D Array(1D array=w1495, element="风机开启温度" ("元素")) -> (index of element=w1517:i32)  [unwired: 1 in]
                    n855 = Search 1D Array(1D array=w1495, element="电压过高一级" ("元素"), start index (0)=w1517) -> (index of element=w1514:i32)
                    n856 = Decrement(x=w1517) -> (x-1=w1519:i32)
                    n857 = Array Subset(array=w1515, index=1 ("索引"), length=w1519) -> (w1521:string[])
                    n858 = Array Subset(array=w1515, index=w1514, length=21 ("长度")) -> (w1499:string[])
                    n859 = Array Subset(array=w1515, index=w1517, length=7 ("长度")) -> (w1512:string[])
                    n860 = Array Subset(array=string[] ["从板板号", "电压个数", "电压起始值", "温度个数", "温度起始值", "第一个保险通道", "第一个保险位置", "第二个保险通道", "第二个保险位置", "第三个保险通道", "第三个保险位置", "第四个保险通道", "第四个保险位置", "第五个保险通道", "第五个保险位置", "第六个保险通道", "第六个保险位置", "第七个保险通道", "第七个保险位置", "第八个保险通道", "第八个保险位置", "第九个保险通道", "第九个保险位置", "第十个保险通道", "第十个保险位置", "第1通道电压个数", "第2通道电压个数", "第3通道电压个数", "第4通道电压个数", "第5通道电压个数", "第6通道电压个数", "第7通道电压个数", "第8通道电压个数", "第9通道电压个数", "第10通道电压个数", "第11通道电压个数", "第12通道电压个数", "第13通道电压个数", "第14通道电压个数", "第15通道电压个数", "第16通道电压个数", "第17通道电压个数", "第18通道电压个数", "第19通道电压个数", "第20通道电压个数", "风机开启温度", "风机关闭温度", "加热开启温度", "加热关闭温度", "风机开启温差", "风机关闭温差", "加热关闭温差", "电压过高一级", "电压过低一级", "温度过高一级", "温度过低一级", "电压不均衡一级", "温度不均衡一级", "SOC过低一级", "电压过高二级", "电压过低二级", "温度过高二级", "温度过低二级", "电压不均衡二级", "温度不均衡二级", "SOC过低二级", "电压过高三级", "电压过低三级", "温度过高三级", "温度过低三级", "电压不均衡三级", "温度不均衡三级", "SOC过低三级", "均衡计算-电压高阀值1级", "均衡计算-电压高阀值2级", "均衡计算-电压低阀值1级", "均衡计算-电压低阀值2级", "均衡计算-最低电压阀值", "均衡停止-最低电压阀值", "均衡计算-电压极差阀值", "充电结束电压(90%)", "充电结束电压(91%)", "充电结束电压(92%)", "充电结束电压(93%)", "充电结束电压(94%)", "充电结束电压(95%)", "充电结束电压(96%)", "充电结束电压(97%)", "充电结束电压(98%)", "充电结束电压(99%)", "充电结束电压(100%)"] ("从板表头"), index=1 ("长度"), length=44 ("长度")) -> (w1489:string[])
                    n861 = for {
                      tunnel: w1499 -> [w1525] mode=indexing
                      tunnel: [w1524] -> w1498 mode=indexing
                      n862 = Fract/Exp String To Number(string=w1525) -> (number=w1524:dbl)  [unwired: 3 in, 1 out]
                    }
                    n863 = for {
                      tunnel: w1512 -> [w1527] mode=indexing
                      tunnel: [w1526] -> w1511 mode=indexing
                      n864 = Fract/Exp String To Number(string=w1527) -> (number=w1526:dbl)  [unwired: 3 in, 1 out]
                    }
                    n865 = Build Array(w1489, w1521) -> (w1520:string[][])
                    n866 = Delete From Array(array=w1498, length=7 ("长度"), index=0 ("索引")) -> (deleted portion=w1507:dbl[], array with subset deleted=w1506:dbl[])
                    n867 = Array To Cluster(array=w1511) -> (cluster=w1510:T10)
                    n868 = Transpose 2D Array(2D array=w1520) -> (transposed array=w1494:string[][])
                    n869 = Delete From Array(array=w1506, length=7 ("长度"), index=0 ("索引")) -> (deleted portion=w1503:dbl[], array with subset deleted=w1502:dbl[])
                    n870 = local write "从板信息电压温度通道配置"(w1494) -> ()
                    n871 = local write "加热控制参数 2"(w1510) -> ()
                    n872 = Build Array(w1507, w1503, w1502) -> (w1501:dbl[][])
                    n873 = Transpose 2D Array(2D array=w1501) -> (transposed array=w1500:dbl[][])
                    n874 = local write "一级故障 2"(w1500) -> ()
                  }
                  frame #2 {
                    n875 = Number To Decimal String(number=w1529) -> (decimal integer string=w1528:string)  [unwired: 1 in]
                    n876 = control-ref of="结果"() -> (w1535:refnum<vi>)
                    n877 = Concatenate Strings("从板", w1528, "导出完成") -> (w1532:string)
                    n878 = Build Array(w1532) -> (w1530:string[])
                    n879 = call "表格编辑.vi"("新元素/子数组"=w1530, "活动单元格:单元格背景色"=u32 6618880, "MCListbox引用句柄"=w1535) -> ()  [unwired: 9 in]
                  }
                }
              }
            }
          }
          frame True {
          }
        }
      }
      event "退出": Value Change {
        n880 = event-data() -> ()  [unwired: 1 in, 6 out]
        n881 = global read "配置文件全局.vi" "参数生成器读取地址"() -> (w1540:path)
        n882 = call <vilib>:"Application Directory.vi"() -> ("Application Directory"=w1546:path)
        n883 = Build Path(base path=w1546, name or relative path="config.ini" ("名称或相对路径")) -> (appended path=w1544:path)
        n884 = call <vilib>:"Open Config Data.vi"("configuration file path"=w1544) -> ("error out"=w1539:errorcluster, "refnum"=w1543:T11)  [unwired: 8 in, 1 out]
        n885 = call-poly <vilib>:"Write Key.vi"("section"="总信息", "error in (no error)"=w1539, "value"=w1540, "key"="参数生成器读取地址" ("section"), "refnum"=w1543) -> ("error out"=w1538:errorcluster, "refnum out"=w1537:T11)  [unwired: 4 in, 1 out]
        n886 = call <vilib>:"Close Config Data.vi"("error in (no error)"=w1538, "refnum"=w1537) -> ("error out"=w1536:errorcluster)  [unwired: 8 in, 1 out]
        n887 = call <vilib>:"Clear Errors.vi"("error in (no error)"=w1536) -> ()  [unwired: 6 in, 1 out]
      }
      event Panel Close? {
        n888 = event-data() -> ()  [unwired: 1 in, 4 out]
        n889 = global read "配置文件全局.vi" "参数生成器读取地址"() -> (w1552:path)
        n890 = call <vilib>:"Application Directory.vi"() -> ("Application Directory"=w1558:path)
        n891 = Build Path(base path=w1558, name or relative path="config.ini" ("名称或相对路径")) -> (appended path=w1556:path)
        n892 = call <vilib>:"Open Config Data.vi"("configuration file path"=w1556) -> ("error out"=w1551:errorcluster, "refnum"=w1555:T11)  [unwired: 8 in, 1 out]
        n893 = call-poly <vilib>:"Write Key.vi"("section"="总信息", "error in (no error)"=w1551, "value"=w1552, "key"="参数生成器读取地址" ("section"), "refnum"=w1555) -> ("error out"=w1550:errorcluster, "refnum out"=w1549:T11)  [unwired: 4 in, 1 out]
        n894 = call <vilib>:"Close Config Data.vi"("error in (no error)"=w1550, "refnum"=w1549) -> ("error out"=w1548:errorcluster)  [unwired: 8 in, 1 out]
        n895 = call <vilib>:"Clear Errors.vi"("error in (no error)"=w1548) -> ()  [unwired: 6 in, 1 out]
        n896 = event-data("Discard?"=FALSE ("放弃？")) -> ()  [unwired: 1 in, 1 out]
      }
      event Timeout {
        n897 = event-data() -> ()  [unwired: 1 in, 3 out]
        n898 = local read "从板个数"() -> (w1563:dbl)
        n899 = control-ref of="从板板号"() -> (w1564:refnum<vi>)
        n900 = property class="DigNum (严格)"(reference=w1564, "Maximum"=w1563, "Minimum"=1.0 ("数据输入界限:最小值")) -> ()  [unwired: 1 in, 2 out]
        n901 = case shown="假" FALSE {
          frame False {
          }
          frame True {
            n902 = local read "从板信息电压温度通道配置"() -> (w1588:string[][])
            n903 = local read "加热控制参数 2"() -> (w1587:T3)
            n904 = local read "一级故障 2"() -> (w1585:dbl[][])
            n905 = Transpose 2D Array(2D array=w1585) -> (transposed array=w1574:dbl[][])
            n906 = Cluster To Array(cluster=w1587) -> (array=w1586:dbl[])
            n907 = local read "均衡参数"() -> (w1568:T1)
            n908 = Array Subset(array=w1588, index (row)=0 ("索引"), index (col)=0 ("索引"), length (col)=2 ("索引")) -> (w1583:string[][])  [unwired: 1 in]
            n909 = for {
              tunnel: w1574 -> [w1600] mode=indexing
              shift-right: [w1599] -> w1581
              shift-left: string[] [] -> [w1597]
              n910 = for {
                N: 7 -> [_]
                tunnel: w1600 -> [w1603] mode=indexing
                tunnel: [w1601] -> w1598 mode=indexing
                n911 = Format Into String(format string="%#f" ("格式字符串"), w1603) -> (resulting string=w1601:string)  [unwired: 2 in, 1 out]
              }
              n912 = Insert Into Array(array=w1597, new element=w1598) -> (w1599:string[])  [unwired: 1 in]
            }
            n913 = Index Array(array=w1583, index (col) #2=1 ("索引 (列)")) -> (element #2=w1571:string[])  [unwired: 3 in, 1 out]
            n914 = for {
              tunnel: w1586 -> [w1606] mode=indexing
              tunnel: [w1604] -> w1582 mode=indexing
              n915 = Format Into String(format string="%#f" ("格式字符串"), w1606) -> (resulting string=w1604:string)  [unwired: 2 in, 1 out]
            }
            n916 = Cluster To Array(cluster=w1568) -> (array=w1567:sgl[])
            n917 = for {
              tunnel: w1567 -> [w1595] mode=indexing
              tunnel: [w1593] -> w1566 mode=indexing
              n918 = Format Into String(format string="%#f" ("格式字符串"), w1595) -> (resulting string=w1593:string)  [unwired: 2 in, 1 out]
            }
            n919 = local read "从板板号"() -> (w1577:dbl)
            n920 = Array Subset(array=w1571, length=28 ("长度")) -> (w1572:string[])  [unwired: 1 in]
            n921 = Number To Decimal String(number=w1577) -> (decimal integer string=w1576:string)  [unwired: 1 in]
            n922 = Insert Into Array(array=w1572, new element #1=w1582, new element #2=w1581, new element #3=w1566) -> (w1580:string[])  [unwired: 1 in]
            n923 = Decrement(x=w1577) -> (x-1=w1573:dbl)
            n924 = local read "输出数组"() -> (w1592:string[][])
            n925 = Insert Into Array(array=w1580, index=0 ("索引"), new element=w1576) -> (w1578:string[])
            n926 = Replace Array Subset(array=w1592, new element=w1578, index (col)=w1573) -> (w1565:string[][])  [unwired: 1 in]
            n927 = local write "从板表头"(string[] ["从板板号", "电压个数", "温度个数", "第一个保险通道", "第一个保险位置", "第二个保险通道", "第二个保险位置", "第三个保险通道", "第三个保险位置", "第四个保险通道", "第四个保险位置", "第五个保险通道", "第五个保险位置", "第六个保险通道", "第六个保险位置", "第七个保险通道", "第七个保险位置", "第八个保险通道", "第八个保险位置", "第九个保险通道", "第九个保险位置", "第十个保险通道", "第十个保险位置", "第1通道电压个数", "第2通道电压个数", "第3通道电压个数", "第4通道电压个数", "第5通道电压个数", "风机开启温度", "风机关闭温度", "加热开启温度", "加热关闭温度", "风机开启温差", "风机关闭温差", "加热关闭温差", "电压过高一级", "电压过低一级", "温度过高一级", "温度过低一级", "电压不均衡一级", "温度不均衡一级", "SOC过低一级", "电压过高二级", "电压过低二级", "温度过高二级", "温度过低二级", "电压不均衡二级", "温度不均衡二级", "SOC过低二级", "电压过高三级", "电压过低三级", "温度过高三级", "温度过低三级", "电压不均衡三级", "温度不均衡三级", "SOC过低三级", "均衡计算-电压高阀值1级", "均衡计算-电压高阀值2级", "均衡计算-电压低阀值1级", "均衡计算-电压低阀值2级", "均衡计算-最低电压阀值", "均衡停止-最低电压阀值", "均衡计算-电压极差阀值", "充电结束电压(90%)", "充电结束电压(91%)", "充电结束电压(92%)", "充电结束电压(93%)", "充电结束电压(94%)", "充电结束电压(95%)", "充电结束电压(96%)", "充电结束电压(97%)", "充电结束电压(98%)", "充电结束电压(99%)", "充电结束电压(100%)"] ("从板表头")) -> ()
            n928 = local write "输出数组"(w1565) -> ()
          }
        }
      }
      event Value Change {
        n929 = event-data() -> ("NewVal"=w1607:T5)  [unwired: 1 in, 5 out]
        n930 = case shown="真" w1607 {
          frame False {
          }
          frame True {
            n931 = local read "从板板号"() -> (w1610:dbl)
            n932 = local read "输出数组"() -> (w1611:string[][])
            n933 = Decrement(x=w1610) -> (x-1=w1609:dbl)
            n934 = Index Array(array=w1611, index (col)=w1609) -> (element=w1608:string[])  [unwired: 1 in]
            n935 = local write "临时从板数据"(w1608) -> ()
          }
        }
      }
      event "粘贴": Value Change {
        n936 = event-data() -> ("NewVal"=w1612:bool)  [unwired: 1 in, 5 out]
        n937 = case shown="真" w1612 {
          frame False {
          }
          frame True {
            n938 = local read "临时从板数据"() -> (w1616:string[])
            n939 = local read "从板板号"() -> (w1617:dbl)
            n940 = local read "输出数组"() -> (w1620:string[][])
            n941 = Decrement(x=w1617) -> (x-1=w1618:dbl)
            n942 = Number To Decimal String(number=w1617) -> (decimal integer string=w1614:string)  [unwired: 1 in]
            n943 = Replace Array Subset(array=w1616, new element=w1614, index=0 ("索引")) -> (w1613:string[])
            n944 = Replace Array Subset(array=w1620, new element=w1613, index (col)=w1618) -> (w1619:string[][])  [unwired: 1 in]
            n945 = local write "输出数组"(w1619) -> ()
            n946 = stacked-sequence {
              tunnel: w1614 -> [w1625]
              frame #0 {
                n947 = control-ref of="结果"() -> (w1627:refnum<vi>)
                n948 = Concatenate Strings("从板", w1625, "粘贴并保存成功") -> (w1623:string)
                n949 = Build Array(w1623) -> (w1621:string[])
                n950 = call "表格编辑.vi"("新元素/子数组"=w1621, "活动单元格:单元格背景色"=u32 6618880, "MCListbox引用句柄"=w1627) -> ()  [unwired: 9 in]
              }
            }
          }
        }
      }
    }
  }
  n951 = stacked-sequence {
    frame #0 {
      w1629 = FALSE ("主页按钮")
      n952 = global read "功能码全局.vi" "主板监控2"() -> (w1631:bool[])
      n953 = control-ref of="单选选项2"() -> (w1638:refnum<vi>)
      n954 = control-ref of="单选选项1"() -> (w1637:refnum<vi>)
      n955 = Build Array(w1637, w1638) -> (w1639:refnum<vi>[])
      n956 = Index Array(array=w1631, index #1=6 ("索引"), index #2=7 ("索引")) -> (element #1=w1633:bool, element #2=w1635:bool)
      n957 = Delete From Array(array=w1639, index=1 ("索引")) -> (deleted portion=w1641:refnum<vi>, array with subset deleted=w1640:refnum<vi>[])  [unwired: 1 in]
      n958 = property on="写配置文件" class="Bool (严格)"("Visible"=w1633) -> ()  [unwired: 2 in, 2 out]
      n959 = property on="读取(ini)" class="Bool (严格)"("Visible"=w1635) -> ()  [unwired: 2 in, 2 out]
      n960 = property on="预览" class="Bool (严格)"("Visible"=w1635) -> ()  [unwired: 2 in, 2 out]
      n961 = property class="Bool (严格)"(reference=w1641, "BoolText.TextColor"=u32 16448250) -> ()  [unwired: 1 in, 2 out]
      n962 = for {
        tunnel: u32 8977151 -> [w1652]
        tunnel: w1640 -> [w1651] mode=indexing
        n963 = property class="Bool (严格)"(reference=w1651, "BoolText.TextColor"=w1652) -> ()  [unwired: 1 in, 2 out]
      }
      n964 = local write "选项卡控件"(enum32{"主板", "从板", "预览"}."主板" ("选项卡控件")) -> ()
      n965 = local write "主从板"(enum32{"单选选项2", "单选选项1"}."单选选项1" ("主从板")) -> ()
      n966 = local write "均衡参数"(T1 {"充电结束电压(90%)"=3.0, "充电结束电压(91%)"=3.0, "充电结束电压(92%)"=3.0, "充电结束电压(93%)"=3.0, "充电结束电压(94%)"=3.0, "均衡计算-电压高阀值1级"=3.0, "均衡计算-电压高阀值2级"=3.0, "均衡计算-电压低阀值1级"=3.0, "均衡计算-电压低阀值2级"=3.0, "均衡计算-最低电压阀值"=3.0, "均衡停止-最低电压阀值"=3.0, "均衡计算-电压极差阀值"=3.0, "充电结束电压(95%)"=3.0, "充电结束电压(96%)"=3.0, "充电结束电压(97%)"=3.0, "充电结束电压(98%)"=3.0, "充电结束电压(99%)"=3.0, "充电结束电压(100%)"=3.0} ("均衡参数")) -> ()
      n967 = local write "从板表头"(string[] [] ("key names")) -> ()
      n968 = control-ref of="结果"() -> (w1649:refnum<vi>)
      n969 = for {
        N: 40 -> [_]
        tunnel: w1649 -> [w1660]
        i -> [w1658]
        n970 = Bundle(w1658, 0) -> (w1656:cluster{i32, i32})  [unwired: 1 out]
        n971 = property class="MCListbox (严格)"(reference=w1660, "ActiveCell"=w1656, "CellBG"=u32 16448250) -> ()  [unwired: 1 in, 2 out]
      }
      n972 = property class="MCListbox (严格)"(reference=w1649, "ItemNames"=string[][] [] ("项名")) -> ()  [unwired: 1 in, 2 out]
      n973 = for {
        N: 100 -> [_]
        tunnel: [w1654] -> w1646 mode=indexing
        n974 = for {
          N: 30 -> [_]
          tunnel: [" "] -> w1654 mode=indexing
        }
      }
      n975 = local write "读主板参数"(w1629) -> ()
      n976 = local write "写配置文件"(w1629) -> ()
      n977 = local write "读从板参数"(w1629) -> ()
      n978 = local write "读取(ini)"(w1629) -> ()
      n979 = local write "预览"(w1629) -> ()
      n980 = local write "退出"(w1629) -> ()
      n981 = local write "输出数组"(w1646) -> ()
      n982 = local write "自动记录"(w1629) -> ()
      n983 = local write "布尔"(w1629) -> ()
      n984 = property on="查看" class="Bool (严格)"("Visible"=w1629) -> ()  [unwired: 2 in, 2 out]
      n985 = call "自适应屏幕分辨率.vi"() -> ()  [unwired: 16 in]
    }
  }
